vi "TCE.vi"() -> (11 "placeholder image":T1(plugin-control))   [LabVIEW 2020]
uses:
  <vilib>/vision/Image Controls.llb/IMAQ Image.ctl
  DataCluster_TCAL.ctl
  TCE_Config.ctl
  <vilib>/Utility/file.llb/Read Delimited Spreadsheet (string).vi
  <vilib>/Utility/file.llb/Write Delimited Spreadsheet (string).vi
  <vilib>/Analysis/NI_AALBase.lvlib
panel:
  out "FreezeFract Concatinated":dbl[](array[numeric])
  in  "Correct Data":bool
  out "Offset Applied?":bool
  out "recentPaths":path[](array[path])=[path "D:/OneDrive/OneDrive - Aarhus Universitet/Data/D20_4/Result Data.csv"]
  out "version":string="version 0.0.0.1" caption="Version"
  out "Title":string="Thermal Camera Evaluation" caption="Version"
  in  "Remove_Correction":bool
  out "Offsets":dbl[](array[numeric])
  in  "Calc_All":bool
  in  "Well":i32=251
  in  "ImageIdx":u32(slide)=98 scale=0.0..527.0
  in  "Path":path
  out "MeltTemps":dbl[](array[numeric])=[-5.408275862068933, -5.766551724137912, -5.134827586206882, -4.684827586206836, -7.485172413793066, -5.2834482758620425, -5.345517241379298, -6.320689655172373, -3.992413793103424, -3.7082758620689447, -3.4782758620689265, -5.388275862068895, -5.597241379310333, -4.740689655172389, -4.031034482758571, -4.187241379310308, -6.245172413793114, -4.773793103448213, -4.427586206896535, -3.742413793103424, -4.568965517241338, -5.621379310344764, -4.7503448275861615, -5.029999999999973, -5.895517241379309, -4.551379310344771, -4.0196551724137635, -4.698965517241334, -4.126551724137926, -2.993448275862022, -4.383448275862065, -4.888965517241331, -5.901724137931012, -8.037586206896549, -3.918275862068924, -4.438620689655181, -5.749655172413782, -4.38241379310341, -4.932758620689583, -4.997586206896528, -4.125862068965489, -3.4279310344827536, -5.144482758620654, -2.891379310344803, -2.92999999999995, -3.1620689655172214, -3.216206896551739, -4.3248275862068795, -1.3320689655172373, -2.026551724137903, 0.5675862068965785, -0.5103448275861524, 0.4782758620689833, -1.9634482758620493, -0.1275862068965239, -0.1651724137930728, -0.9937931034482403, -0.6210344827586027, 0.2934482758620902, 0.6917241379310894, 1.3537931034483108, -1.852758620689599, -1.3782758620689037, 1.2606896551724844, -0.0275862068965012, -2.2548275862068294, -1.0710344827585914, -1.4565517241379098, -0.7220689655172237, -0.853793103448254, -0.2686206896551653, -0.5562068965517142, 0.0324137931034443, -0.2768965517241213, 1.1982758620689538, 1.2775862068966148, -0.6427586206896194, 0.5986206896552062, -0.3313793103448006, -0.6034482758620356, -2.0755172413792593, -2.182758620689583, -1.6548275862068635, -0.7234482758620402, -0.6872413793103078, -0.9086206896551516, -0.5427586206895967, -0.0527586206895876, 1.211379310344853, 0.2365517241379393, -0.526551724137903, -0.1537931034482085, 1.1865517241379848, 0.7089655172413813, -1.8837931034482267, 0.5872413793103988, -2.0686206896551766, -2.519310344827545, -2.2079310344827263, -2.2441379310344587, -2.0355172413792957, -2.3782758620689037, -2.0879310344827218, -1.998965517241345, -2.0948275862068613, -2.1227586206896376, -2.195517241379264, -1.969655172413752, -2.0175862068965102, -2.061724137931037, -2.028275862068938, -1.7403448275861706, -2.1765517241378802, -2.432758620689583, -2.186551724137928, -2.063448275862015, -2.331724137931019, -2.1351724137931, -2.0499999999999545, -2.1537931034482085, -2.235172413793066, -2.213793103448211, -2.082758620689617, -2.1703448275861774, -2.0434482758620334, -2.173448275862029, -1.9048275862068635, -1.683793103448238, -1.8931034482758378, -2.165172413793073, -2.068965517241338, -2.1862068965517096, -2.161034482758623, -2.085517241379307, -2.0631034482758537, -2.134137931034445, -2.104827586206852, -2.1775862068965353, -2.2255172413792934, -2.161724137931003, -2.0251724137930864, -2.0106896551724276, -2.211379310344796, -1.9093103448275315, -2.3158620689654867, -1.9827586206895944, -2.258275862068899, -2.2927586206895967, -2.0868965517241236, -2.0810344827585823, -2.17931034482757, -2.134137931034445, -2.151379310344794, -2.101034482758621, -2.2465517241379303, -2.339999999999975, -2.061379310344819, -2.082413793103399, -2.220689655172407, -2.0658620689654867, -2.1337931034482267, -2.0158620689654754, -2.1179310344827513, -2.1999999999999886, -2.130344827586157, -2.0489655172413563, -2.0534482758620243, -2.0851724137930887, -2.1079310344827036, -2.0241379310344882, -2.0693103448275565, -2.1348275862068817, -2.1431034482758378, -2.0268965517241213, -2.0317241379310076, -1.6172413793103146, -2.02103448275858, -2.331724137931019, -2.4068965517241168, -2.2337931034482494, -2.383103448275847, -2.1417241379310212, -2.1768965517240986, -2.2579310344827377, -2.1786206896551334, -2.032068965517226, -2.1162068965517165, -2.2706896551724185, -1.9220689655172123, -2.174482758620684, -2.11206896551721, -2.0858620689654686, -0.1458620689654708, -0.1541379310344837, -0.0103448275861524, -0.2106896551724162, -0.2299999999999613, -0.243448275862022, -0.2624137931034056, -0.2906896551724003, -0.3306896551724208, -0.3089655172413472, -0.2099999999999795, -0.276551724137903, -0.15896551724137, -0.0637931034482335, -0.2572413793103578, 0.1706896551724526, -0.0779310344827309, -0.0958620689654595, 0.0658620689655436, -0.1041379310344723, -0.4631034482758308, -0.1158620689654981, -0.1268965517240872, -0.3313793103448006, -0.2803448275861911, -0.1562068965517369, -0.06793103448274, -0.131379310344812, -0.0282758620689378, 0.0079310344827945, 0.0748275862069363, 0.2665517241379689, 0.0537931034482995, -0.2062068965516914, -0.1179310344827513, -0.3424137931033897, -0.0275862068965012, -0.2003448275861501, -0.1096551724137953, -0.0944827586206429, -0.4137931034482563, -0.5093103448275542, 0.0627586206896922, -0.1789655172413518, -0.0096551724137726, 0.0068965517241395, -0.0334482758620425, 0.2120689655172896, -0.1099999999999568, -0.2282758620689265, -0.1213793103447642, -0.1482758620689424, -0.2106896551724162, -0.0927586206896081, -0.1093103448275201, -0.076206896551696, -0.1593103448275315, -0.0886206896551585, -0.1924137931034124, -0.0558620689654958, -0.0313793103447892, -0.0799999999999841, -0.1262068965517074, 0.2117241379310713, -0.1141379310344632, -0.1796551724137885, -0.2003448275861501, -0.0327586206896058, 0.0655172413793252, -0.1886206896551812, -0.0327586206896058, -0.1424137931034011, -0.2406896551723889, -0.034827586206859, -0.1527586206896103, -0.1848275862068363, -0.0313793103447892, -0.0158620689654754, -0.0372413793103306, 0.2079310344827832, -0.2451724137931137, -0.6586206896551516, -0.0858620689654686, -0.2462068965517119, -0.2631034482758423, -0.0217241379310167, -0.2486206896551266, 0.0455172413793434, -0.2441379310344587, -0.1786206896551334, -0.230689655172398, -0.0131034482758423, -0.2613793103448074, -0.4093103448275315, -0.0124137931034056, 0.1572413793103919, 0.0, 0.0, 0.0, 1.7110344827586346, 1.5944827586206998, 1.9227586206896488, 0.1648275862069113, 1.3268965517241327, 0.0, 0.0, 0.0, 1.441379310344871, 0.8996551724138158, 2.017586206896567, 1.1068965517241622, 2.3413793103448484, 1.119655172413843, 1.9251724137931205, 1.484482758620743, 1.7410344827586641, 1.624137931034511, 1.9227586206896488, 1.88793103448279, 1.3758620689655459, -0.8037931034482426, 1.6562068965517938, 1.90758620689661, 2.0327586206896626, 1.5831034482758923, 2.1006896551724594, 2.216206896551796, 2.153448275862104, 1.9158620689655093, 2.1862068965517665, 1.9189655172414175, 2.0968965517241713, 1.4434482758620675, 1.914482758620693, 1.868620689655188, 1.9841379310345246, 2.0734482758621198, 1.9231034482759242, 1.7982758620689765, 1.852068965517276, 2.086551724137962, 2.055172413793173, 1.9510344827586437, 2.1220689655172578, 2.108620689655197, 2.3431034482758832, 0.0, 1.7272413793103851, 2.039655172413859, 1.9255172413793389, 2.2200000000000273, 1.5868965517241804, 1.914482758620693, 1.9610344827586343, 2.145517241379366, 1.9279310344828102, 1.8203448275862115, 2.199310344827609, 2.312413793103474, 2.407931034482772, 2.4206896551724526, 1.8224137931034647, 2.3637931034483017, 1.6882758620689629, 1.8193103448276133, 1.7324137931034898, 2.3037931034482995, 1.794137931034527, 2.011034482758646, 2.0013793103448734, 1.7558620689655413, 1.8893103448276065, 2.1520689655172873, 1.9962068965517685, 2.3103448275862206, 2.1217241379310963, 1.863103448275922, 1.9231034482759242, 1.5434482758620902, 1.6648275862069113, 1.8944827586207111, 1.63793103448279, 1.8379310344827786, 1.948620689655229, 2.157241379310392, 1.835517241379364, 1.950344827586207, 2.018275862069004, 1.9565517241379666, 1.7651724137931524, 2.068965517241395, 2.168275862068981]
  out "FreezeArray":bool[](array[boolean])=[TRUE, TRUE, TRUE, TRUE, TRUE, TRUE, TRUE, TRUE, TRUE, TRUE, TRUE, TRUE, TRUE, TRUE, TRUE, TRUE, TRUE, TRUE, TRUE, TRUE, TRUE, TRUE, TRUE, TRUE, TRUE, TRUE, TRUE, TRUE, TRUE, TRUE, TRUE, TRUE, TRUE, TRUE, TRUE, TRUE, TRUE, TRUE, TRUE, TRUE, TRUE, TRUE, TRUE, TRUE, TRUE, TRUE, TRUE, TRUE, TRUE, TRUE, TRUE, TRUE, TRUE, TRUE, TRUE, TRUE, TRUE, TRUE, TRUE, TRUE, TRUE, TRUE, TRUE, TRUE, TRUE, TRUE, TRUE, TRUE, TRUE, TRUE, TRUE, TRUE, TRUE, TRUE, TRUE, TRUE, TRUE, TRUE, TRUE, TRUE, TRUE, TRUE, TRUE, TRUE, TRUE, TRUE, TRUE, TRUE, TRUE, TRUE, TRUE, TRUE, TRUE, TRUE, TRUE, TRUE, TRUE, TRUE, TRUE, TRUE, TRUE, TRUE, TRUE, TRUE, TRUE, TRUE, TRUE, TRUE, TRUE, TRUE, TRUE, TRUE, TRUE, TRUE, TRUE, TRUE, TRUE, TRUE, TRUE, TRUE, TRUE, TRUE, TRUE, TRUE, TRUE, TRUE, TRUE, TRUE, TRUE, TRUE, TRUE, TRUE, TRUE, TRUE, TRUE, TRUE, TRUE, TRUE, TRUE, TRUE, TRUE, TRUE, TRUE, TRUE, TRUE, TRUE, TRUE, TRUE, TRUE, TRUE, TRUE, TRUE, TRUE, TRUE, TRUE, TRUE, TRUE, TRUE, TRUE, TRUE, TRUE, TRUE, TRUE, TRUE, TRUE, TRUE, TRUE, TRUE, TRUE, TRUE, TRUE, TRUE, TRUE, TRUE, TRUE, TRUE, TRUE, TRUE, TRUE, TRUE, TRUE, TRUE, TRUE, TRUE, TRUE, TRUE, TRUE, TRUE, TRUE, TRUE, TRUE, TRUE, TRUE, TRUE, TRUE, TRUE, TRUE, TRUE, TRUE, TRUE, TRUE, TRUE, TRUE, TRUE, TRUE, TRUE, TRUE, TRUE, TRUE, TRUE, TRUE, TRUE, TRUE, TRUE, TRUE, TRUE, TRUE, TRUE, TRUE, TRUE, TRUE, TRUE, TRUE, TRUE, TRUE, TRUE, TRUE, TRUE, TRUE, TRUE, TRUE, TRUE, TRUE, TRUE, TRUE, TRUE, TRUE, TRUE, TRUE, TRUE, TRUE, TRUE, TRUE, TRUE, TRUE, TRUE, TRUE, TRUE, TRUE, TRUE, TRUE, TRUE, TRUE, TRUE, TRUE, TRUE, TRUE, TRUE, TRUE, TRUE, TRUE, TRUE, TRUE, TRUE, TRUE, TRUE, TRUE, TRUE, TRUE, TRUE, TRUE, TRUE, TRUE, TRUE, TRUE, TRUE, TRUE, TRUE, TRUE, TRUE, TRUE, TRUE, TRUE, TRUE, TRUE, TRUE, TRUE, TRUE, FALSE, FALSE, FALSE, TRUE, TRUE, TRUE, TRUE, TRUE, FALSE, FALSE, FALSE, TRUE, TRUE, TRUE, TRUE, TRUE, TRUE, TRUE, TRUE, TRUE, TRUE, TRUE, TRUE, TRUE, TRUE, TRUE, TRUE, TRUE, TRUE, TRUE, TRUE, TRUE, TRUE, TRUE, TRUE, TRUE, TRUE, TRUE, TRUE, TRUE, TRUE, TRUE, TRUE, TRUE, TRUE, TRUE, TRUE, TRUE, TRUE, TRUE, FALSE, TRUE, TRUE, TRUE, TRUE, TRUE, TRUE, TRUE, TRUE, TRUE, TRUE, TRUE, TRUE, TRUE, TRUE, TRUE, TRUE, TRUE, TRUE, TRUE, TRUE, TRUE, TRUE, TRUE, TRUE, TRUE, TRUE, TRUE, TRUE, TRUE, TRUE, TRUE, TRUE, TRUE, TRUE, TRUE, TRUE, TRUE, TRUE, TRUE, TRUE, TRUE, TRUE, TRUE, TRUE, TRUE]
  out "ThermTemps":dbl[](array[numeric])
  out "PartitionArray":string[](array[string])=["A, MQ unfiltered", "A, MQ unfiltered", "A, MQ unfiltered", "A, MQ unfiltered", "A, MQ unfiltered", "A, MQ unfiltered", "A, MQ unfiltered", "A, MQ unfiltered", "A, MQ unfiltered", "A, MQ unfiltered", "A, MQ unfiltered", "A, MQ unfiltered", "A, MQ unfiltered", "A, MQ unfiltered", "A, MQ unfiltered", "A, MQ unfiltered", "A, MQ unfiltered", "A, MQ unfiltered", "A, MQ unfiltered", "A, MQ unfiltered", "A, MQ unfiltered", "A, MQ unfiltered", "A, MQ unfiltered", "A, MQ unfiltered", "A, MQ unfiltered", "A, MQ unfiltered", "A, MQ unfiltered", "A, MQ unfiltered", "A, MQ unfiltered", "A, MQ unfiltered", "A, MQ unfiltered", "A, MQ unfiltered", "A, MQ unfiltered", "A, MQ unfiltered", "A, MQ unfiltered", "A, MQ unfiltered", "A, MQ unfiltered", "A, MQ unfiltered", "A, MQ unfiltered", "A, MQ unfiltered", "A, MQ unfiltered", "A, MQ unfiltered", "A, MQ unfiltered", "A, MQ unfiltered", "A, MQ unfiltered", "A, MQ unfiltered", "A, MQ unfiltered", "A, MQ unfiltered", "B, D2O unfiltered", "B, D2O unfiltered", "B, D2O unfiltered", "B, D2O unfiltered", "B, D2O unfiltered", "B, D2O unfiltered", "B, D2O unfiltered", "B, D2O unfiltered", "B, D2O unfiltered", "B, D2O unfiltered", "B, D2O unfiltered", "B, D2O unfiltered", "B, D2O unfiltered", "B, D2O unfiltered", "B, D2O unfiltered", "B, D2O unfiltered", "B, D2O unfiltered", "B, D2O unfiltered", "B, D2O unfiltered", "B, D2O unfiltered", "B, D2O unfiltered", "B, D2O unfiltered", "B, D2O unfiltered", "B, D2O unfiltered", "B, D2O unfiltered", "B, D2O unfiltered", "B, D2O unfiltered", "B, D2O unfiltered", "B, D2O unfiltered", "B, D2O unfiltered", "B, D2O unfiltered", "B, D2O unfiltered", "B, D2O unfiltered", "B, D2O unfiltered", "B, D2O unfiltered", "B, D2O unfiltered", "B, D2O unfiltered", "B, D2O unfiltered", "B, D2O unfiltered", "B, D2O unfiltered", "B, D2O unfiltered", "B, D2O unfiltered", "B, D2O unfiltered", "B, D2O unfiltered", "B, D2O unfiltered", "B, D2O unfiltered", "B, D2O unfiltered", "B, D2O unfiltered", "C, 1mg/ml Snomax in MQ", "C, 1mg/ml Snomax in MQ", "C, 1mg/ml Snomax in MQ", "C, 1mg/ml Snomax in MQ", "C, 1mg/ml Snomax in MQ", "C, 1mg/ml Snomax in MQ", "C, 1mg/ml Snomax in MQ", "C, 1mg/ml Snomax in MQ", "C, 1mg/ml Snomax in MQ", "C, 1mg/ml Snomax in MQ", "C, 1mg/ml Snomax in MQ", "C, 1mg/ml Snomax in MQ", "C, 1mg/ml Snomax in MQ", "C, 1mg/ml Snomax in MQ", "C, 1mg/ml Snomax in MQ", "C, 1mg/ml Snomax in MQ", "C, 1mg/ml Snomax in MQ", "C, 1mg/ml Snomax in MQ", "C, 1mg/ml Snomax in MQ", "C, 1mg/ml Snomax in MQ", "C, 1mg/ml Snomax in MQ", "C, 1mg/ml Snomax in MQ", "C, 1mg/ml Snomax in MQ", "C, 1mg/ml Snomax in MQ", "C, 1mg/ml Snomax in MQ", "C, 1mg/ml Snomax in MQ", "C, 1mg/ml Snomax in MQ", "C, 1mg/ml Snomax in MQ", "C, 1mg/ml Snomax in MQ", "C, 1mg/ml Snomax in MQ", "C, 1mg/ml Snomax in MQ", "C, 1mg/ml Snomax in MQ", "C, 1mg/ml Snomax in MQ", "C, 1mg/ml Snomax in MQ", "C, 1mg/ml Snomax in MQ", "C, 1mg/ml Snomax in MQ", "C, 1mg/ml Snomax in MQ", "C, 1mg/ml Snomax in MQ", "C, 1mg/ml Snomax in MQ", "C, 1mg/ml Snomax in MQ", "C, 1mg/ml Snomax in MQ", "C, 1mg/ml Snomax in MQ", "C, 1mg/ml Snomax in MQ", "C, 1mg/ml Snomax in MQ", "C, 1mg/ml Snomax in MQ", "C, 1mg/ml Snomax in MQ", "C, 1mg/ml Snomax in MQ", "C, 1mg/ml Snomax in MQ", "C, 1mg/ml Snomax in MQ", "C, 1mg/ml Snomax in MQ", "C, 1mg/ml Snomax in MQ", "C, 1mg/ml Snomax in MQ", "C, 1mg/ml Snomax in MQ", "C, 1mg/ml Snomax in MQ", "C, 1mg/ml Snomax in MQ", "C, 1mg/ml Snomax in MQ", "C, 1mg/ml Snomax in MQ", "C, 1mg/ml Snomax in MQ", "C, 1mg/ml Snomax in MQ", "C, 1mg/ml Snomax in MQ", "C, 1mg/ml Snomax in MQ", "C, 1mg/ml Snomax in MQ", "C, 1mg/ml Snomax in MQ", "C, 1mg/ml Snomax in MQ", "C, 1mg/ml Snomax in MQ", "C, 1mg/ml Snomax in MQ", "C, 1mg/ml Snomax in MQ", "C, 1mg/ml Snomax in MQ", "C, 1mg/ml Snomax in MQ", "C, 1mg/ml Snomax in MQ", "C, 1mg/ml Snomax in MQ", "C, 1mg/ml Snomax in MQ", "C, 1mg/ml Snomax in MQ", "C, 1mg/ml Snomax in MQ", "C, 1mg/ml Snomax in MQ", "C, 1mg/ml Snomax in MQ", "C, 1mg/ml Snomax in MQ", "C, 1mg/ml Snomax in MQ", "C, 1mg/ml Snomax in MQ", "C, 1mg/ml Snomax in MQ", "C, 1mg/ml Snomax in MQ", "C, 1mg/ml Snomax in MQ", "C, 1mg/ml Snomax in MQ", "C, 1mg/ml Snomax in MQ", "C, 1mg/ml Snomax in MQ", "C, 1mg/ml Snomax in MQ", "C, 1mg/ml Snomax in MQ", "C, 1mg/ml Snomax in MQ", "C, 1mg/ml Snomax in MQ", "C, 1mg/ml Snomax in MQ", "C, 1mg/ml Snomax in MQ", "C, 1mg/ml Snomax in MQ", "C, 1mg/ml Snomax in MQ", "C, 1mg/ml Snomax in MQ", "C, 1mg/ml Snomax in MQ", "C, 1mg/ml Snomax in MQ", "D, 1mg/ml Snomax in 1:1 MQ:D2O", "D, 1mg/ml Snomax in 1:1 MQ:D2O", "D, 1mg/ml Snomax in 1:1 MQ:D2O", "D, 1mg/ml Snomax in 1:1 MQ:D2O", "D, 1mg/ml Snomax in 1:1 MQ:D2O", "D, 1mg/ml Snomax in 1:1 MQ:D2O", "D, 1mg/ml Snomax in 1:1 MQ:D2O", "D, 1mg/ml Snomax in 1:1 MQ:D2O", "D, 1mg/ml Snomax in 1:1 MQ:D2O", "D, 1mg/ml Snomax in 1:1 MQ:D2O", "D, 1mg/ml Snomax in 1:1 MQ:D2O", "D, 1mg/ml Snomax in 1:1 MQ:D2O", "D, 1mg/ml Snomax in 1:1 MQ:D2O", "D, 1mg/ml Snomax in 1:1 MQ:D2O", "D, 1mg/ml Snomax in 1:1 MQ:D2O", "D, 1mg/ml Snomax in 1:1 MQ:D2O", "D, 1mg/ml Snomax in 1:1 MQ:D2O", "D, 1mg/ml Snomax in 1:1 MQ:D2O", "D, 1mg/ml Snomax in 1:1 MQ:D2O", "D, 1mg/ml Snomax in 1:1 MQ:D2O", "D, 1mg/ml Snomax in 1:1 MQ:D2O", "D, 1mg/ml Snomax in 1:1 MQ:D2O", "D, 1mg/ml Snomax in 1:1 MQ:D2O", "D, 1mg/ml Snomax in 1:1 MQ:D2O", "D, 1mg/ml Snomax in 1:1 MQ:D2O", "D, 1mg/ml Snomax in 1:1 MQ:D2O", "D, 1mg/ml Snomax in 1:1 MQ:D2O", "D, 1mg/ml Snomax in 1:1 MQ:D2O", "D, 1mg/ml Snomax in 1:1 MQ:D2O", "D, 1mg/ml Snomax in 1:1 MQ:D2O", "D, 1mg/ml Snomax in 1:1 MQ:D2O", "D, 1mg/ml Snomax in 1:1 MQ:D2O", "D, 1mg/ml Snomax in 1:1 MQ:D2O", "D, 1mg/ml Snomax in 1:1 MQ:D2O", "D, 1mg/ml Snomax in 1:1 MQ:D2O", "D, 1mg/ml Snomax in 1:1 MQ:D2O", "D, 1mg/ml Snomax in 1:1 MQ:D2O", "D, 1mg/ml Snomax in 1:1 MQ:D2O", "D, 1mg/ml Snomax in 1:1 MQ:D2O", "D, 1mg/ml Snomax in 1:1 MQ:D2O", "D, 1mg/ml Snomax in 1:1 MQ:D2O", "D, 1mg/ml Snomax in 1:1 MQ:D2O", "D, 1mg/ml Snomax in 1:1 MQ:D2O", "D, 1mg/ml Snomax in 1:1 MQ:D2O", "D, 1mg/ml Snomax in 1:1 MQ:D2O", "D, 1mg/ml Snomax in 1:1 MQ:D2O", "D, 1mg/ml Snomax in 1:1 MQ:D2O", "D, 1mg/ml Snomax in 1:1 MQ:D2O", "D, 1mg/ml Snomax in 1:1 MQ:D2O", "D, 1mg/ml Snomax in 1:1 MQ:D2O", "D, 1mg/ml Snomax in 1:1 MQ:D2O", "D, 1mg/ml Snomax in 1:1 MQ:D2O", "D, 1mg/ml Snomax in 1:1 MQ:D2O", "D, 1mg/ml Snomax in 1:1 MQ:D2O", "D, 1mg/ml Snomax in 1:1 MQ:D2O", "D, 1mg/ml Snomax in 1:1 MQ:D2O", "D, 1mg/ml Snomax in 1:1 MQ:D2O", "D, 1mg/ml Snomax in 1:1 MQ:D2O", "D, 1mg/ml Snomax in 1:1 MQ:D2O", "D, 1mg/ml Snomax in 1:1 MQ:D2O", "D, 1mg/ml Snomax in 1:1 MQ:D2O", "D, 1mg/ml Snomax in 1:1 MQ:D2O", "D, 1mg/ml Snomax in 1:1 MQ:D2O", "D, 1mg/ml Snomax in 1:1 MQ:D2O", "D, 1mg/ml Snomax in 1:1 MQ:D2O", "D, 1mg/ml Snomax in 1:1 MQ:D2O", "D, 1mg/ml Snomax in 1:1 MQ:D2O", "D, 1mg/ml Snomax in 1:1 MQ:D2O", "D, 1mg/ml Snomax in 1:1 MQ:D2O", "D, 1mg/ml Snomax in 1:1 MQ:D2O", "D, 1mg/ml Snomax in 1:1 MQ:D2O", "D, 1mg/ml Snomax in 1:1 MQ:D2O", "D, 1mg/ml Snomax in 1:1 MQ:D2O", "D, 1mg/ml Snomax in 1:1 MQ:D2O", "D, 1mg/ml Snomax in 1:1 MQ:D2O", "D, 1mg/ml Snomax in 1:1 MQ:D2O", "D, 1mg/ml Snomax in 1:1 MQ:D2O", "D, 1mg/ml Snomax in 1:1 MQ:D2O", "D, 1mg/ml Snomax in 1:1 MQ:D2O", "D, 1mg/ml Snomax in 1:1 MQ:D2O", "D, 1mg/ml Snomax in 1:1 MQ:D2O", "D, 1mg/ml Snomax in 1:1 MQ:D2O", "D, 1mg/ml Snomax in 1:1 MQ:D2O", "D, 1mg/ml Snomax in 1:1 MQ:D2O", "D, 1mg/ml Snomax in 1:1 MQ:D2O", "D, 1mg/ml Snomax in 1:1 MQ:D2O", "D, 1mg/ml Snomax in 1:1 MQ:D2O", "D, 1mg/ml Snomax in 1:1 MQ:D2O", "D, 1mg/ml Snomax in 1:1 MQ:D2O", "D, 1mg/ml Snomax in 1:1 MQ:D2O", "D, 1mg/ml Snomax in 1:1 MQ:D2O", "D, 1mg/ml Snomax in 1:1 MQ:D2O", "D, 1mg/ml Snomax in 1:1 MQ:D2O", "D, 1mg/ml Snomax in 1:1 MQ:D2O", "D, 1mg/ml Snomax in 1:1 MQ:D2O", "D, 1mg/ml Snomax in 1:1 MQ:D2O", "E, 1mg/ml Snomax in D2O", "E, 1mg/ml Snomax in D2O", "E, 1mg/ml Snomax in D2O", "E, 1mg/ml Snomax in D2O", "E, 1mg/ml Snomax in D2O", "E, 1mg/ml Snomax in D2O", "E, 1mg/ml Snomax in D2O", "E, 1mg/ml Snomax in D2O", "E, 1mg/ml Snomax in D2O", "E, 1mg/ml Snomax in D2O", "E, 1mg/ml Snomax in D2O", "E, 1mg/ml Snomax in D2O", "E, 1mg/ml Snomax in D2O", "E, 1mg/ml Snomax in D2O", "E, 1mg/ml Snomax in D2O", "E, 1mg/ml Snomax in D2O", "E, 1mg/ml Snomax in D2O", "E, 1mg/ml Snomax in D2O", "E, 1mg/ml Snomax in D2O", "E, 1mg/ml Snomax in D2O", "E, 1mg/ml Snomax in D2O", "E, 1mg/ml Snomax in D2O", "E, 1mg/ml Snomax in D2O", "E, 1mg/ml Snomax in D2O", "E, 1mg/ml Snomax in D2O", "E, 1mg/ml Snomax in D2O", "E, 1mg/ml Snomax in D2O", "E, 1mg/ml Snomax in D2O", "E, 1mg/ml Snomax in D2O", "E, 1mg/ml Snomax in D2O", "E, 1mg/ml Snomax in D2O", "E, 1mg/ml Snomax in D2O", "E, 1mg/ml Snomax in D2O", "E, 1mg/ml Snomax in D2O", "E, 1mg/ml Snomax in D2O", "E, 1mg/ml Snomax in D2O", "E, 1mg/ml Snomax in D2O", "E, 1mg/ml Snomax in D2O", "E, 1mg/ml Snomax in D2O", "E, 1mg/ml Snomax in D2O", "E, 1mg/ml Snomax in D2O", "E, 1mg/ml Snomax in D2O", "E, 1mg/ml Snomax in D2O", "E, 1mg/ml Snomax in D2O", "E, 1mg/ml Snomax in D2O", "E, 1mg/ml Snomax in D2O", "E, 1mg/ml Snomax in D2O", "E, 1mg/ml Snomax in D2O", "E, 1mg/ml Snomax in D2O", "E, 1mg/ml Snomax in D2O", "E, 1mg/ml Snomax in D2O", "E, 1mg/ml Snomax in D2O", "E, 1mg/ml Snomax in D2O", "E, 1mg/ml Snomax in D2O", "E, 1mg/ml Snomax in D2O", "E, 1mg/ml Snomax in D2O", "E, 1mg/ml Snomax in D2O", "E, 1mg/ml Snomax in D2O", "E, 1mg/ml Snomax in D2O", "E, 1mg/ml Snomax in D2O", "E, 1mg/ml Snomax in D2O", "E, 1mg/ml Snomax in D2O", "E, 1mg/ml Snomax in D2O", "E, 1mg/ml Snomax in D2O", "E, 1mg/ml Snomax in D2O", "E, 1mg/ml Snomax in D2O", "E, 1mg/ml Snomax in D2O", "E, 1mg/ml Snomax in D2O", "E, 1mg/ml Snomax in D2O", "E, 1mg/ml Snomax in D2O", "E, 1mg/ml Snomax in D2O", "E, 1mg/ml Snomax in D2O", "E, 1mg/ml Snomax in D2O", "E, 1mg/ml Snomax in D2O", "E, 1mg/ml Snomax in D2O", "E, 1mg/ml Snomax in D2O", "E, 1mg/ml Snomax in D2O", "E, 1mg/ml Snomax in D2O", "E, 1mg/ml Snomax in D2O", "E, 1mg/ml Snomax in D2O", "E, 1mg/ml Snomax in D2O", "E, 1mg/ml Snomax in D2O", "E, 1mg/ml Snomax in D2O", "E, 1mg/ml Snomax in D2O", "E, 1mg/ml Snomax in D2O", "E, 1mg/ml Snomax in D2O", "E, 1mg/ml Snomax in D2O", "E, 1mg/ml Snomax in D2O", "E, 1mg/ml Snomax in D2O", "E, 1mg/ml Snomax in D2O", "E, 1mg/ml Snomax in D2O", "E, 1mg/ml Snomax in D2O", "E, 1mg/ml Snomax in D2O", "E, 1mg/ml Snomax in D2O", "E, 1mg/ml Snomax in D2O", "E, 1mg/ml Snomax in D2O"]
  out "FreezeTemps":dbl[](array[numeric])=[-17.102413793103437, -16.14275862068962, -19.01724137931032, -15.683103448275858, -25.12241379310342, -20.5310344827586, -21.968275862068907, -23.725862068965483, -16.464137931034486, -13.113793103448245, -11.636206896551698, -22.81517241379308, -23.049655172413765, -15.513103448275842, -18.779655172413783, -15.36448275862068, -23.218620689655154, -14.564137931034452, -14.352413793103437, -11.641724137931021, -17.657241379310335, -21.99793103448272, -23.813103448275854, -20.459310344827543, -22.592068965517228, -22.526206896551713, -16.890344827586148, -17.801724137931018, -17.235862068965474, -11.44310344827585, -16.035862068965457, -17.472413793103414, -17.914827586206854, -25.26724137931032, -15.10206896551722, -15.265862068965474, -22.079999999999984, -18.58586206896547, -20.5106896551724, -21.002758620689605, -21.88206896551722, -14.302068965517208, -23.049655172413765, -11.56448275862067, -9.727586206896547, -10.574482758620661, -10.471724137931005, -14.189999999999998, -18.853448275862036, -20.565517241379297, -14.187241379310308, -14.840344827586193, -14.906206896551737, -21.08172413793102, -19.829655172413766, -16.151379310344794, -20.792413793103407, -21.82482758620685, -14.474482758620638, -8.87551724137927, -5.148275862068942, -22.100689655172403, -21.813103448275854, -5.387931034482733, -13.19965517241377, -22.069655172413775, -20.66206896551722, -20.594137931034453, -19.319655172413775, -20.309999999999974, -16.707241379310346, -21.968275862068907, -18.70620689655172, -18.623448275862046, -6.637931034482733, -7.056206896551714, -22.052068965517208, -9.618275862068913, -16.901724137931012, -13.387241379310353, -20.70034482758618, -21.344137931034453, -21.40620689655171, -16.127241379310362, -20.572413793103408, -19.566206896551705, -19.49379310344824, -16.083448275862054, -5.782758620689606, -14.221034482758569, -19.863103448275837, -17.482068965517215, -5.9048275862068635, -8.006896551724083, -20.81793103448271, -11.433103448275858, -5.199999999999989, -5.525862068965466, -5.633448275862065, -5.417241379310326, -5.608965517241359, -5.6537931034482085, -5.74655172413793, -5.684482758620675, -5.691379310344814, -5.6758620689655, -5.808620689655129, -5.717586206896556, -5.676206896551719, -5.526896551724121, -5.435517241379273, -5.398620689655161, -5.285172413793077, -5.59172413793101, -5.664482758620636, -5.389999999999986, -5.610344827586175, -5.809999999999945, -5.582413793103399, -5.736896551724101, -5.824482758620661, -5.701379310344805, -5.67655172413788, -5.683103448275858, -5.648965517241322, -5.654482758620645, -5.394482758620654, -5.2789655172413745, -5.4324137931034215, -5.434482758620675, -5.513448275862061, -5.627931034482742, -5.778275862068938, -5.713103448275831, -5.601034482758621, -5.630689655172375, -5.699310344827552, -5.584482758620652, -5.70379310344822, -5.636896551724078, -5.628275862068904, -5.4948275862068385, -5.689310344827561, -5.402413793103392, -5.240689655172389, -5.448275862068897, -5.5555172413792775, -5.998965517241345, -5.548965517241356, -5.420689655172396, -5.645862068965471, -5.577931034482731, -5.6520689655172305, -5.590344827586193, -5.699999999999989, -5.640689655172423, -5.6299999999999955, -5.599310344827529, -5.45034482758615, -5.28793103448271, -5.263793103448222, -5.557931034482749, -5.471034482758569, -5.670344827586177, -5.626551724137926, -5.3606896551723935, -5.553448275862024, -5.736206896551721, -5.485517241379284, -5.536206896551732, -5.615862068965498, -5.4589655172413245, -5.904137931034484, -5.572413793103408, -5.5565517241379325, -5.072413793103408, -5.54482758620685, -5.425172413793064, -5.9865517241378825, -5.601724137931001, -5.816551724137923, -5.833448275862054, -5.495517241379275, -5.722068965517224, -5.5058620689654845, -5.552758620689588, -5.644137931034493, -5.5610344827586005, -5.523793103448213, -5.626551724137926, -5.5406896551724, -5.328275862068949, -2.799310344827518, -3.109999999999957, -3.088965517241377, -3.2558620689654845, -3.3810344827585936, -3.349310344827529, -3.327931034482731, -3.3241379310344428, -3.2679310344827286, -3.4796551724138, -3.1096551724137953, -3.299655172413793, -3.301379310344771, -3.1603448275861865, -2.941034482758596, -2.9506896551724253, -2.8889655172413313, -3.0858620689654686, -2.980689655172398, -3.146896551724126, -3.077931034482731, -3.2044827586206566, -3.164482758620636, -3.3927586206896194, -3.373103448275856, -3.2824137931033874, -3.2603448275861524, -3.264482758620659, -3.188275862068906, -3.086206896551687, -2.978965517241363, -2.9113793103447847, -2.8717241379310394, -3.0813793103448006, -3.0013793103448165, -2.8927586206896194, -3.1879310344827445, -3.2431034482758605, -3.254482758620668, -3.1889655172413427, -3.319655172413775, -3.3893103448275497, -3.1068965517241054, -2.8872413793103533, -2.9982758620689083, -3.2041379310344382, -3.2024137931034033, -2.812413793103417, -2.790344827586182, -3.00068965517238, -3.1693103448275224, -3.193103448275849, -3.195862068965482, -3.1141379310344632, -3.326896551724076, -3.2120689655172328, -3.224137931034477, -3.285862068965457, -3.215862068965464, -3.0582758620689106, -3.1924137931034124, -3.149655172413759, -3.17999999999995, -2.8662068965517165, -2.9058620689654617, -3.0134482758620607, -3.161724137931003, -3.131379310344812, -3.0813793103448006, -3.0351724137930773, -2.9986206896551266, -3.1968965517240804, -3.164482758620636, -3.0810344827585823, -3.220689655172407, -2.9931034482758605, -2.964137931034486, -3.17999999999995, -2.9920689655172055, -2.764827586206877, -2.886896551724078, -3.1758620689655004, -3.071724137931028, -3.196551724137919, -3.2237931034482585, -2.905172413793082, -3.262068965517244, -3.1627586206896012, -3.283793103448261, -3.164482758620636, -3.142413793103401, -3.1089655172413586, -3.034137931034479, -3.277586206896558, -3.0720689655172464, -2.629655172413777, 0.0, 0.0, 0.0, -0.7296551724137998, -1.1386206896551698, -1.0558620689654958, -1.305172413793116, -1.1862068965517096, 0.0, 0.0, 0.0, -1.1282758620689037, -1.1682758620689242, -0.5724137931034079, -1.1765517241378802, -0.2555172413792661, -1.0703448275861547, -0.7648275862068772, -1.057931034482749, -1.016551724137912, -0.9627586206896126, -1.0337931034482608, -0.9872413793103192, -1.2451724137931137, -1.3141379310344519, -1.0437931034482517, -1.0199999999999818, -0.95310344827584, -0.9817241379309962, -0.8799999999999955, -0.7527586206896331, -0.5689655172413381, -0.6779310344827536, -0.7651724137930955, -0.8879310344827331, -0.8582758620689219, -1.0286206896551562, -0.8986206896551607, -1.072413793103408, -0.8858620689654799, -0.9524137931034033, -0.9465517241379189, -0.9465517241379189, -0.6958620689654822, -0.9386206896551812, -0.6879310344827445, -0.8244827586206611, -0.540344827586182, -0.5341379310344792, -0.6255172413792707, 0.0, -0.8917241379310212, -0.8031034482758628, -0.7927586206895967, -0.3927586206896194, -1.0141379310344405, -0.7241379310344769, -0.8258620689654776, -0.8099999999999454, -0.7320689655172146, -0.8993103448275406, -0.6624137931034397, -0.5572413793103124, -0.355517241379289, 0.0244827586207066, -0.6931034482758491, -0.113103448275865, -0.8486206896551494, -0.581724137931019, -0.4658620689654641, -0.1306896551723753, -0.9151724137930728, -0.8689655172413495, -0.5741379310344428, -0.8624137931034284, -0.8899999999999864, -0.8365517241379052, -0.7541379310344496, -0.5631034482758537, -0.4710344827585686, -0.3586206896551403, -0.4551724137930933, -0.7186206896551539, -0.8586206896551403, -0.6134482758620265, -0.6841379310344564, -0.6020689655172191, -0.8358620689654686, -0.6906896551723776, -0.8324137931033988, -0.900689655172414, -0.5879310344827218, -0.8486206896551494, -0.6179310344827513, -0.4758620689654549, -0.4237931034482472]
  out "FreezeIdx":i32[](array[numeric])=[255, 242, 272, 236, 335, 287, 303, 320, 243, 209, 191, 311, 316, 234, 271, 238, 322, 225, 219, 192, 254, 301, 321, 283, 307, 309, 248, 257, 253, 193, 240, 259, 264, 335, 231, 232, 302, 265, 285, 291, 301, 219, 312, 192, 172, 182, 181, 221, 271, 285, 224, 228, 233, 290, 279, 240, 286, 296, 218, 162, 122, 305, 300, 128, 213, 302, 285, 284, 271, 280, 243, 297, 267, 262, 143, 147, 302, 170, 248, 214, 293, 293, 293, 240, 287, 272, 273, 236, 129, 217, 278, 252, 135, 153, 288, 192, 124, 131, 130, 125, 127, 127, 126, 129, 124, 127, 126, 126, 129, 126, 124, 128, 126, 126, 135, 125, 133, 136, 126, 131, 132, 131, 126, 125, 129, 132, 125, 128, 128, 127, 124, 126, 136, 130, 125, 129, 125, 134, 131, 126, 130, 125, 133, 128, 125, 130, 133, 137, 127, 124, 126, 124, 127, 126, 133, 130, 124, 133, 132, 124, 124, 129, 126, 128, 128, 123, 132, 131, 125, 127, 125, 124, 136, 126, 129, 126, 129, 126, 135, 126, 133, 130, 124, 126, 124, 124, 126, 123, 125, 125, 124, 129, 98, 100, 98, 105, 99, 102, 98, 100, 97, 104, 97, 98, 100, 99, 97, 99, 99, 105, 99, 106, 107, 99, 108, 104, 104, 100, 100, 98, 103, 98, 98, 99, 102, 106, 108, 96, 100, 108, 104, 99, 100, 108, 98, 97, 97, 99, 98, 98, 99, 99, 99, 110, 108, 100, 111, 100, 99, 107, 99, 98, 101, 99, 99, 99, 98, 98, 99, 99, 101, 107, 98, 99, 100, 98, 104, 98, 98, 99, 99, 98, 98, 99, 98, 100, 101, 100, 106, 101, 100, 99, 100, 99, 98, 102, 99, 98, 0, 0, 0, 71, 80, 75, 84, 81, 0, 0, 0, 74, 77, 72, 78, 75, 81, 73, 76, 80, 77, 76, 76, 82, 88, 77, 78, 79, 74, 74, 81, 78, 76, 75, 75, 77, 76, 82, 75, 74, 76, 83, 81, 72, 74, 73, 74, 74, 73, 79, 0, 79, 74, 75, 82, 76, 73, 80, 75, 73, 82, 73, 75, 79, 80, 77, 77, 74, 73, 73, 89, 77, 75, 71, 76, 76, 74, 74, 75, 73, 74, 71, 76, 78, 74, 74, 72, 75, 75, 75, 75, 73, 77, 73, 73, 75]
  out "maxSize":i32=527
  out "img":i32
  out "Slide":u8(slide) scale=0.0..100.0
  in  "Help":bool
  out "Tutorial":string="Load Image"
  out "Points":T2[](array[typedef])=[{"X"=62.0, "Y"=65.0}, {"X"=62.333332, "Y"=80.6}, {"X"=62.666668, "Y"=96.2}, {"X"=63.0, "Y"=111.8}, {"X"=63.333332, "Y"=127.4}, {"X"=63.666668, "Y"=143.0}, {"X"=64.0, "Y"=158.6}, {"X"=64.333336, "Y"=174.20001}, {"X"=64.666664, "Y"=189.8}, {"X"=65.0, "Y"=205.40001}, {"X"=65.333336, "Y"=221.0}, {"X"=65.666664, "Y"=236.6}, {"X"=66.0, "Y"=252.20001}, {"X"=66.333336, "Y"=267.8}, {"X"=66.666664, "Y"=283.40002}, {"X"=67.0, "Y"=299.0}, {"X"=77.565216, "Y"=64.695656}, {"X"=77.89855, "Y"=80.295654}, {"X"=78.23188, "Y"=95.89565}, {"X"=78.565216, "Y"=111.49565}, {"X"=78.89855, "Y"=127.09566}, {"X"=79.23188, "Y"=142.69565}, {"X"=79.565216, "Y"=158.29565}, {"X"=79.89855, "Y"=173.89566}, {"X"=80.23188, "Y"=189.49567}, {"X"=80.565216, "Y"=205.09566}, {"X"=80.89855, "Y"=220.69565}, {"X"=81.23188, "Y"=236.29565}, {"X"=81.565216, "Y"=251.89566}, {"X"=81.89855, "Y"=267.49567}, {"X"=82.23188, "Y"=283.09564}, {"X"=82.565216, "Y"=298.69565}, {"X"=93.13043, "Y"=64.391304}, {"X"=93.46377, "Y"=79.9913}, {"X"=93.797104, "Y"=95.59131}, {"X"=94.13043, "Y"=111.19131}, {"X"=94.46377, "Y"=126.791306}, {"X"=94.797104, "Y"=142.3913}, {"X"=95.13043, "Y"=157.9913}, {"X"=95.46377, "Y"=173.59131}, {"X"=95.797104, "Y"=189.19131}, {"X"=96.13043, "Y"=204.79132}, {"X"=96.46377, "Y"=220.39131}, {"X"=96.797104, "Y"=235.99132}, {"X"=97.13043, "Y"=251.59132}, {"X"=97.46377, "Y"=267.1913}, {"X"=97.797104, "Y"=282.79132}, {"X"=98.13043, "Y"=298.3913}, {"X"=108.69565, "Y"=64.08696}, {"X"=109.028984, "Y"=79.68696}, {"X"=109.36232, "Y"=95.28696}, {"X"=109.695656, "Y"=110.88696}, {"X"=110.028984, "Y"=126.48695}, {"X"=110.36232, "Y"=142.08696}, {"X"=110.695656, "Y"=157.68697}, {"X"=111.028984, "Y"=173.28696}, {"X"=111.36232, "Y"=188.88696}, {"X"=111.695656, "Y"=204.48697}, {"X"=112.028984, "Y"=220.08696}, {"X"=112.36232, "Y"=235.68697}, {"X"=112.695656, "Y"=251.28697}, {"X"=113.028984, "Y"=266.88696}, {"X"=113.36232, "Y"=282.48697}, {"X"=113.695656, "Y"=298.08698}, {"X"=124.260864, "Y"=63.782608}, {"X"=124.5942, "Y"=79.38261}, {"X"=124.927536, "Y"=94.982605}, {"X"=125.26087, "Y"=110.58261}, {"X"=125.5942, "Y"=126.18261}, {"X"=125.927536, "Y"=141.78261}, {"X"=126.26087, "Y"=157.38261}, {"X"=126.5942, "Y"=172.9826}, {"X"=126.927536, "Y"=188.58261}, {"X"=127.26087, "Y"=204.18262}, {"X"=127.5942, "Y"=219.78261}, {"X"=127.927536, "Y"=235.38261}, {"X"=128.26086, "Y"=250.98262}, {"X"=128.59421, "Y"=266.5826}, {"X"=128.92754, "Y"=282.18262}, {"X"=129.26086, "Y"=297.7826}, {"X"=139.82608, "Y"=63.47826}, {"X"=140.15942, "Y"=79.07826}, {"X"=140.49275, "Y"=94.67826}, {"X"=140.8261, "Y"=110.27826}, {"X"=141.15942, "Y"=125.878265}, {"X"=141.49275, "Y"=141.47827}, {"X"=141.8261, "Y"=157.07828}, {"X"=142.15942, "Y"=172.67827}, {"X"=142.49275, "Y"=188.27826}, {"X"=142.8261, "Y"=203.87827}, {"X"=143.15942, "Y"=219.47826}, {"X"=143.49275, "Y"=235.07826}, {"X"=143.8261, "Y"=250.67827}, {"X"=144.15942, "Y"=266.27826}, {"X"=144.49275, "Y"=281.87827}, {"X"=144.8261, "Y"=297.47827}, {"X"=155.3913, "Y"=63.173912}, {"X"=155.72464, "Y"=78.77391}, {"X"=156.05797, "Y"=94.37392}, {"X"=156.39131, "Y"=109.973915}, {"X"=156.72464, "Y"=125.57391}, {"X"=157.05797, "Y"=141.17392}, {"X"=157.39131, "Y"=156.77393}, {"X"=157.72464, "Y"=172.37392}, {"X"=158.05797, "Y"=187.9739}, {"X"=158.39131, "Y"=203.57393}, {"X"=158.72464, "Y"=219.17392}, {"X"=159.05797, "Y"=234.77393}, {"X"=159.39131, "Y"=250.37393}, {"X"=159.72464, "Y"=265.97394}, {"X"=160.05797, "Y"=281.5739}, {"X"=160.39131, "Y"=297.17392}, {"X"=170.95651, "Y"=62.869564}, {"X"=171.28986, "Y"=78.46957}, {"X"=171.62318, "Y"=94.069565}, {"X"=171.95653, "Y"=109.66957}, {"X"=172.28986, "Y"=125.26956}, {"X"=172.62318, "Y"=140.86957}, {"X"=172.95653, "Y"=156.46957}, {"X"=173.28986, "Y"=172.06958}, {"X"=173.62318, "Y"=187.66957}, {"X"=173.95653, "Y"=203.26958}, {"X"=174.28986, "Y"=218.86957}, {"X"=174.62318, "Y"=234.46957}, {"X"=174.95653, "Y"=250.06958}, {"X"=175.28986, "Y"=265.66956}, {"X"=175.62318, "Y"=281.2696}, {"X"=175.95653, "Y"=296.86957}, {"X"=186.52173, "Y"=62.565216}, {"X"=186.85507, "Y"=78.16522}, {"X"=187.1884, "Y"=93.76522}, {"X"=187.52174, "Y"=109.36522}, {"X"=187.85507, "Y"=124.96522}, {"X"=188.1884, "Y"=140.56522}, {"X"=188.52174, "Y"=156.16522}, {"X"=188.85507, "Y"=171.76523}, {"X"=189.1884, "Y"=187.36522}, {"X"=189.52174, "Y"=202.96523}, {"X"=189.85507, "Y"=218.56522}, {"X"=190.1884, "Y"=234.16522}, {"X"=190.52174, "Y"=249.76523}, {"X"=190.85507, "Y"=265.36523}, {"X"=191.1884, "Y"=280.9652}, {"X"=191.52174, "Y"=296.56522}, {"X"=202.08696, "Y"=62.260868}, {"X"=202.42029, "Y"=77.86087}, {"X"=202.75363, "Y"=93.46087}, {"X"=203.08696, "Y"=109.06087}, {"X"=203.42029, "Y"=124.66087}, {"X"=203.75363, "Y"=140.26086}, {"X"=204.08696, "Y"=155.86087}, {"X"=204.42029, "Y"=171.46088}, {"X"=204.75363, "Y"=187.06088}, {"X"=205.08696, "Y"=202.66087}, {"X"=205.42029, "Y"=218.26086}, {"X"=205.75363, "Y"=233.86087}, {"X"=206.08696, "Y"=249.46088}, {"X"=206.42029, "Y"=265.06085}, {"X"=206.75363, "Y"=280.6609}, {"X"=207.08696, "Y"=296.26086}, {"X"=217.65218, "Y"=61.95652}, {"X"=217.9855, "Y"=77.55652}, {"X"=218.31885, "Y"=93.156525}, {"X"=218.65218, "Y"=108.75652}, {"X"=218.9855, "Y"=124.35652}, {"X"=219.31885, "Y"=139.95651}, {"X"=219.65218, "Y"=155.55652}, {"X"=219.9855, "Y"=171.15652}, {"X"=220.31885, "Y"=186.75653}, {"X"=220.65218, "Y"=202.35654}, {"X"=220.9855, "Y"=217.95653}, {"X"=221.31885, "Y"=233.55653}, {"X"=221.65218, "Y"=249.15654}, {"X"=221.9855, "Y"=264.75653}, {"X"=222.31885, "Y"=280.35654}, {"X"=222.65218, "Y"=295.95654}, {"X"=233.21739, "Y"=61.652176}, {"X"=233.55072, "Y"=77.252174}, {"X"=233.88406, "Y"=92.85217}, {"X"=234.21739, "Y"=108.45218}, {"X"=234.55072, "Y"=124.05218}, {"X"=234.88406, "Y"=139.65218}, {"X"=235.21739, "Y"=155.25218}, {"X"=235.55072, "Y"=170.85217}, {"X"=235.88406, "Y"=186.45218}, {"X"=236.21739, "Y"=202.05219}, {"X"=236.55072, "Y"=217.65218}, {"X"=236.88406, "Y"=233.25218}, {"X"=237.21739, "Y"=248.85219}, {"X"=237.55072, "Y"=264.45218}, {"X"=237.88406, "Y"=280.0522}, {"X"=238.21739, "Y"=295.65216}, {"X"=248.78261, "Y"=61.347828}, {"X"=249.11594, "Y"=76.94783}, {"X"=249.44928, "Y"=92.54783}, {"X"=249.78261, "Y"=108.14783}, {"X"=250.11594, "Y"=123.74783}, {"X"=250.44928, "Y"=139.34782}, {"X"=250.78261, "Y"=154.94783}, {"X"=251.11594, "Y"=170.54782}, {"X"=251.44928, "Y"=186.14783}, {"X"=251.78261, "Y"=201.74783}, {"X"=252.11594, "Y"=217.34782}, {"X"=252.44928, "Y"=232.94783}, {"X"=252.78261, "Y"=248.54784}, {"X"=253.11594, "Y"=264.14783}, {"X"=253.44928, "Y"=279.74783}, {"X"=253.78261, "Y"=295.34784}, {"X"=264.34784, "Y"=61.04348}, {"X"=264.68115, "Y"=76.64348}, {"X"=265.0145, "Y"=92.24348}, {"X"=265.34784, "Y"=107.84348}, {"X"=265.68115, "Y"=123.44348}, {"X"=266.0145, "Y"=139.04349}, {"X"=266.34784, "Y"=154.6435}, {"X"=266.68115, "Y"=170.24348}, {"X"=267.0145, "Y"=185.84348}, {"X"=267.34784, "Y"=201.44348}, {"X"=267.68115, "Y"=217.04347}, {"X"=268.0145, "Y"=232.64348}, {"X"=268.34784, "Y"=248.24348}, {"X"=268.68115, "Y"=263.84348}, {"X"=269.0145, "Y"=279.44348}, {"X"=269.34784, "Y"=295.04346}, {"X"=279.91302, "Y"=60.739132}, {"X"=280.24637, "Y"=76.33913}, {"X"=280.5797, "Y"=91.93913}, {"X"=280.91306, "Y"=107.53914}, {"X"=281.24637, "Y"=123.13913}, {"X"=281.5797, "Y"=138.73914}, {"X"=281.91306, "Y"=154.33914}, {"X"=282.24637, "Y"=169.93913}, {"X"=282.5797, "Y"=185.53912}, {"X"=282.91306, "Y"=201.13914}, {"X"=283.24637, "Y"=216.73914}, {"X"=283.5797, "Y"=232.33914}, {"X"=283.91306, "Y"=247.93915}, {"X"=284.24637, "Y"=263.53912}, {"X"=284.5797, "Y"=279.13916}, {"X"=284.91306, "Y"=294.73914}, {"X"=295.47827, "Y"=60.434784}, {"X"=295.81158, "Y"=76.03478}, {"X"=296.14493, "Y"=91.63478}, {"X"=296.47827, "Y"=107.23479}, {"X"=296.81158, "Y"=122.834785}, {"X"=297.14493, "Y"=138.43478}, {"X"=297.47827, "Y"=154.03479}, {"X"=297.81158, "Y"=169.6348}, {"X"=298.14493, "Y"=185.23479}, {"X"=298.47827, "Y"=200.8348}, {"X"=298.81158, "Y"=216.43478}, {"X"=299.14493, "Y"=232.03479}, {"X"=299.47827, "Y"=247.6348}, {"X"=299.81158, "Y"=263.2348}, {"X"=300.14493, "Y"=278.83478}, {"X"=300.47827, "Y"=294.43478}, {"X"=311.04346, "Y"=60.130436}, {"X"=311.3768, "Y"=75.73044}, {"X"=311.71014, "Y"=91.33044}, {"X"=312.0435, "Y"=106.930435}, {"X"=312.3768, "Y"=122.53044}, {"X"=312.71014, "Y"=138.13043}, {"X"=313.0435, "Y"=153.73044}, {"X"=313.3768, "Y"=169.33044}, {"X"=313.71014, "Y"=184.93044}, {"X"=314.0435, "Y"=200.53044}, {"X"=314.3768, "Y"=216.13043}, {"X"=314.71014, "Y"=231.73044}, {"X"=315.0435, "Y"=247.33044}, {"X"=315.3768, "Y"=262.93042}, {"X"=315.71014, "Y"=278.53046}, {"X"=316.0435, "Y"=294.13043}, {"X"=326.6087, "Y"=59.826088}, {"X"=326.94205, "Y"=75.42609}, {"X"=327.27536, "Y"=91.02609}, {"X"=327.6087, "Y"=106.62609}, {"X"=327.94205, "Y"=122.22609}, {"X"=328.27536, "Y"=137.82608}, {"X"=328.6087, "Y"=153.42609}, {"X"=328.94205, "Y"=169.0261}, {"X"=329.27536, "Y"=184.6261}, {"X"=329.6087, "Y"=200.22609}, {"X"=329.94205, "Y"=215.82608}, {"X"=330.27536, "Y"=231.42609}, {"X"=330.6087, "Y"=247.0261}, {"X"=330.94205, "Y"=262.6261}, {"X"=331.27536, "Y"=278.22607}, {"X"=331.6087, "Y"=293.82608}, {"X"=342.17392, "Y"=59.52174}, {"X"=342.50726, "Y"=75.12174}, {"X"=342.84058, "Y"=90.72174}, {"X"=343.17392, "Y"=106.32175}, {"X"=343.50726, "Y"=121.92174}, {"X"=343.84058, "Y"=137.52173}, {"X"=344.17392, "Y"=153.12173}, {"X"=344.50726, "Y"=168.72174}, {"X"=344.84058, "Y"=184.32175}, {"X"=345.17392, "Y"=199.92175}, {"X"=345.50726, "Y"=215.52174}, {"X"=345.84058, "Y"=231.12175}, {"X"=346.17392, "Y"=246.72176}, {"X"=346.50726, "Y"=262.32175}, {"X"=346.84058, "Y"=277.92175}, {"X"=347.17392, "Y"=293.52173}, {"X"=357.73914, "Y"=59.217392}, {"X"=358.07248, "Y"=74.81739}, {"X"=358.4058, "Y"=90.41739}, {"X"=358.73914, "Y"=106.017395}, {"X"=359.07248, "Y"=121.61739}, {"X"=359.4058, "Y"=137.21739}, {"X"=359.73914, "Y"=152.8174}, {"X"=360.07248, "Y"=168.41739}, {"X"=360.4058, "Y"=184.0174}, {"X"=360.73914, "Y"=199.6174}, {"X"=361.07248, "Y"=215.21739}, {"X"=361.4058, "Y"=230.8174}, {"X"=361.73914, "Y"=246.4174}, {"X"=362.07248, "Y"=262.0174}, {"X"=362.4058, "Y"=277.6174}, {"X"=362.73914, "Y"=293.2174}, {"X"=373.30435, "Y"=58.913044}, {"X"=373.6377, "Y"=74.51305}, {"X"=373.971, "Y"=90.113045}, {"X"=374.30435, "Y"=105.71304}, {"X"=374.6377, "Y"=121.31305}, {"X"=374.971, "Y"=136.91304}, {"X"=375.30435, "Y"=152.51305}, {"X"=375.6377, "Y"=168.11305}, {"X"=375.971, "Y"=183.71304}, {"X"=376.30435, "Y"=199.31305}, {"X"=376.6377, "Y"=214.91304}, {"X"=376.971, "Y"=230.51305}, {"X"=377.30435, "Y"=246.11305}, {"X"=377.6377, "Y"=261.71304}, {"X"=377.971, "Y"=277.31305}, {"X"=378.30435, "Y"=292.91302}, {"X"=388.86957, "Y"=58.608696}, {"X"=389.2029, "Y"=74.208694}, {"X"=389.53622, "Y"=89.8087}, {"X"=389.86957, "Y"=105.4087}, {"X"=390.2029, "Y"=121.0087}, {"X"=390.53622, "Y"=136.6087}, {"X"=390.86957, "Y"=152.20871}, {"X"=391.2029, "Y"=167.8087}, {"X"=391.53622, "Y"=183.40869}, {"X"=391.86957, "Y"=199.0087}, {"X"=392.2029, "Y"=214.6087}, {"X"=392.53622, "Y"=230.20871}, {"X"=392.86957, "Y"=245.80872}, {"X"=393.2029, "Y"=261.4087}, {"X"=393.53622, "Y"=277.0087}, {"X"=393.86957, "Y"=292.6087}, {"X"=404.43478, "Y"=58.304348}, {"X"=404.76813, "Y"=73.90435}, {"X"=405.10144, "Y"=89.50435}, {"X"=405.43478, "Y"=105.104355}, {"X"=405.76813, "Y"=120.704346}, {"X"=406.10144, "Y"=136.30435}, {"X"=406.43478, "Y"=151.90436}, {"X"=406.76813, "Y"=167.50435}, {"X"=407.10144, "Y"=183.10435}, {"X"=407.43478, "Y"=198.70436}, {"X"=407.76813, "Y"=214.30435}, {"X"=408.10144, "Y"=229.90436}, {"X"=408.43478, "Y"=245.50436}, {"X"=408.76813, "Y"=261.10437}, {"X"=409.10144, "Y"=276.70435}, {"X"=409.43478, "Y"=292.30435}, {"X"=420.0, "Y"=58.0}, {"X"=420.33334, "Y"=73.6}, {"X"=420.66666, "Y"=89.2}, {"X"=421.0, "Y"=104.8}, {"X"=421.33334, "Y"=120.4}, {"X"=421.66666, "Y"=136.0}, {"X"=422.0, "Y"=151.6}, {"X"=422.33334, "Y"=167.20001}, {"X"=422.66666, "Y"=182.8}, {"X"=423.0, "Y"=198.40001}, {"X"=423.33334, "Y"=214.0}, {"X"=423.66666, "Y"=229.6}, {"X"=424.0, "Y"=245.20001}, {"X"=424.33334, "Y"=260.8}, {"X"=424.66666, "Y"=276.40002}, {"X"=425.0, "Y"=292.0}] {"Y" format="%.2f"; "X" format="%.2f"}
  out "Image":T1(plugin-control)
  out "MeltTemp":dbl=-0.0558620689654958 caption="Melt temp" format="%.3g °C"
  out "FreezeTemp":dbl=-3.0582758620689106 caption="Froze at" format="%.3g °C"
  out "Title 2":string="Well Data" caption="Version"
  out "Well":string="L16"
  out "CurTemp":dbl=-0.9882758620689174 caption="Temp" format="%.3g °C"
  out "Contents":string="D, 1mg/ml Snomax in 1:1 MQ:D2O"
  out "Temps":dbl[][](graph)
  out "Temps single":dbl[](graph)
  out "Fraction Single":dbl[](graph)=[0.0, 0.0, 0.0, 0.0, 0.0, 0.0, 0.0, 0.0, 0.0, 0.0, 0.0, 0.0, 0.0, 0.0, 0.0, 0.0, 0.0, 0.0, 0.0, 0.0, 0.0, 0.0, 0.0, 0.0, 0.0, 0.0, 0.0, 0.0, 0.0, 0.0, 0.0, 0.0, 0.0, 0.0, 0.0, 0.0, 0.0, 0.0, 0.0, 0.0, 0.0, 0.0, 0.0, 0.0, 0.0, 0.0, 0.0, 0.0, 0.0, 0.0, 0.0, 0.0, 0.0, 0.0, 0.0, 0.0, 0.0, 0.0, 0.0, 0.0, 0.0, 0.0, 0.0, 0.0, 0.0, 0.0, 0.0, 0.0, 0.0, 0.0, 0.0, 0.0, 0.0, 0.0, 0.0, 0.0, 0.0, 0.0, 0.0, 0.0, 0.0, 0.0, 0.0, 0.0, 0.0, 0.0, 0.0, 0.0, 0.0, 0.0, 0.0, 0.0, 0.0, 0.0, 0.0, 0.0, 0.0, 0.05263157894736842, 0.28421052631578947, 0.5578947368421052, 0.7052631578947368, 0.7473684210526316, 0.7789473684210526, 0.7894736842105263, 0.8421052631578947, 0.8631578947368421, 0.8947368421052632, 0.9263157894736842, 0.9789473684210527, 0.9789473684210527, 0.9894736842105263, 1.0, 1.0, 1.0, 1.0, 1.0, 1.0, 1.0, 1.0, 1.0, 1.0, 1.0, 1.0, 1.0, 1.0, 1.0, 1.0, 1.0, 1.0, 1.0, 1.0, 1.0, 1.0, 1.0, 1.0, 1.0, 1.0, 1.0, 1.0, 1.0, 1.0, 1.0, 1.0, 1.0, 1.0, 1.0, 1.0, 1.0, 1.0, 1.0, 1.0, 1.0, 1.0, 1.0, 1.0, 1.0, 1.0, 1.0, 1.0, 1.0, 1.0, 1.0, 1.0, 1.0, 1.0, 1.0, 1.0, 1.0, 1.0, 1.0, 1.0, 1.0, 1.0, 1.0, 1.0, 1.0, 1.0, 1.0, 1.0, 1.0, 1.0, 1.0, 1.0, 1.0, 1.0, 1.0, 1.0, 1.0, 1.0, 1.0, 1.0, 1.0, 1.0, 1.0, 1.0, 1.0, 1.0, 1.0, 1.0, 1.0, 1.0, 1.0, 1.0, 1.0, 1.0, 1.0, 1.0, 1.0, 1.0, 1.0, 1.0, 1.0, 1.0, 1.0, 1.0, 1.0, 1.0, 1.0, 1.0, 1.0, 1.0, 1.0, 1.0, 1.0, 1.0, 1.0, 1.0, 1.0, 1.0, 1.0, 1.0, 1.0, 1.0, 1.0, 1.0, 1.0, 1.0, 1.0, 1.0, 1.0, 1.0, 1.0, 1.0, 1.0, 1.0, 1.0, 1.0, 1.0, 1.0, 1.0, 1.0, 1.0, 1.0, 1.0, 1.0, 1.0, 1.0, 1.0, 1.0, 1.0, 1.0, 1.0, 1.0, 1.0, 1.0, 1.0, 1.0, 1.0, 1.0, 1.0, 1.0, 1.0, 1.0, 1.0, 1.0, 1.0, 1.0, 1.0, 1.0, 1.0, 1.0, 1.0, 1.0, 1.0, 1.0, 1.0, 1.0, 1.0, 1.0, 1.0, 1.0, 1.0, 1.0, 1.0, 1.0, 1.0, 1.0, 1.0, 1.0, 1.0, 1.0, 1.0, 1.0, 1.0, 1.0, 1.0, 1.0, 1.0, 1.0, 1.0, 1.0, 1.0, 1.0, 1.0, 1.0, 1.0, 1.0, 1.0, 1.0, 1.0, 1.0, 1.0, 1.0, 1.0, 1.0, 1.0, 1.0, 1.0, 1.0, 1.0, 1.0, 1.0, 1.0, 1.0, 1.0, 1.0, 1.0, 1.0, 1.0, 1.0, 1.0, 1.0, 1.0, 1.0, 1.0, 1.0, 1.0, 1.0, 1.0, 1.0, 1.0, 1.0, 1.0, 1.0, 1.0, 1.0, 1.0, 1.0, 1.0, 1.0, 1.0, 1.0, 1.0, 1.0, 1.0, 1.0, 1.0, 1.0, 1.0, 1.0, 1.0, 1.0, 1.0, 1.0, 1.0, 1.0, 1.0, 1.0, 1.0, 1.0, 1.0, 1.0, 1.0, 1.0, 1.0, 1.0, 1.0, 1.0, 1.0, 1.0, 1.0, 1.0, 1.0, 1.0, 1.0, 1.0, 1.0, 1.0, 1.0, 1.0, 1.0, 1.0, 1.0, 1.0, 1.0, 1.0, 1.0, 1.0, 1.0, 1.0, 1.0, 1.0, 1.0, 1.0, 1.0, 1.0, 1.0, 1.0, 1.0, 1.0, 1.0, 1.0, 1.0, 1.0, 1.0, 1.0, 1.0, 1.0, 1.0, 1.0, 1.0, 1.0, 1.0, 1.0, 1.0, 1.0, 1.0, 1.0, 1.0, 1.0, 1.0, 1.0, 1.0, 1.0, 1.0, 1.0, 1.0, 1.0, 1.0, 1.0, 1.0, 1.0, 1.0, 1.0, 1.0, 1.0, 1.0, 1.0, 1.0, 1.0, 1.0, 1.0, 1.0, 1.0, 1.0, 1.0, 1.0, 1.0, 1.0, 1.0, 1.0, 1.0, 1.0, 1.0, 1.0, 1.0, 1.0, 1.0, 1.0, 1.0, 1.0, 1.0, 1.0, 1.0, 1.0, 1.0, 1.0, 1.0, 1.0, 1.0, 1.0, 1.0, 1.0, 1.0, 1.0, 1.0, 1.0, 1.0, 1.0, 1.0, 1.0, 1.0, 1.0, 1.0, 1.0, 1.0, 1.0, 1.0, 1.0, 1.0, 1.0, 1.0, 1.0, 1.0, 1.0, 1.0, 1.0, 1.0, 1.0, 1.0, 1.0, 1.0, 1.0, 1.0, 1.0, 1.0, 1.0, 1.0]
  out "FrozenFractionGraph":dbl[][](graph)
  out "Temps single grad":dbl[](graph)
  out "Temps grads":dbl[][](graph)
  # "hints: \nUse the Mouse Wheel to zoom in and out"
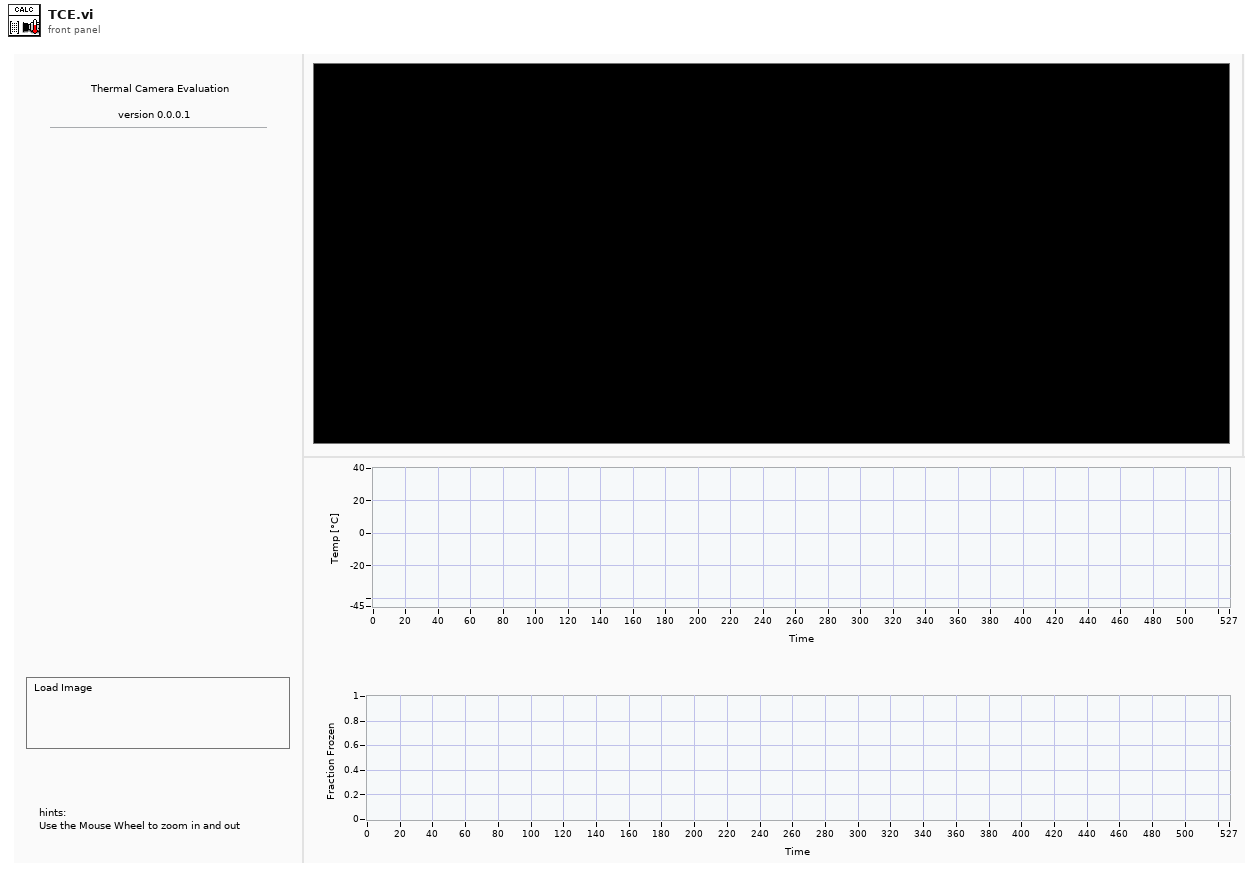
[diagram p1: front panel]
types:
  T1 = typedef "IMAQ Image.ctl" = refnum<image>
  T2 = typedef "IMAQ Point" = cluster{"X":sgl, "Y":sgl}
  T3 = enum32{"Invalid", "Standard", "Closed", "Hidden", "Minimized", "Maximized"}
  T4 = enum32{"invalid app kind", "Development System", "Run Time System", "Student Edition", "Embedded LabVIEW", "Evaluation", "Custom"}
  T5 = typedef "DataCluster_TCAL.ctl" = cluster{"Core":cluster{"Current VI Reference":refnum<vi>, "Close Panel on Exit?":bool}, "Image Out":T1, "State":i32, "Points":cluster{"Top Left":T2, "Top Right":T2, "Bottom Left":T2, "Bottom Right":T2, "x space 2":dbl, "y space 2":sgl, "x_space":sgl, "y_space":sgl, "Pixels":cluster{"X":i32, "Y":i32}[][], "Fixpoint":T2}, "img_array":T1[], "Temps":dbl[], "Temps_Array":dbl[][], "Scan Area":dbl, "Fixpoint Area":dbl, "Config":T6, "PCR Size":u16}
  T6 = typedef "TCE_Config.ctl" = cluster{"Freezing":cluster{"Cutoff":dbl}}
  T7 = cluster{"Global Rectangle":i32[], "Contours":cluster{"Contour Type":u32, "ROI Type":u32, "Points":i32[]}[]}
  T8 = enum8{"Enabled", "Disabled", "Disabled and Grayed Out"}
  T9 = cluster{"Desired Font (Application)":enum16{"User-specified Font", "Application Font", "System Font", "Dialog Font"}, "[User-specified Font]":cluster{"Font Name":string, "Size":i16, "Strikeout?":bool, "Italic?":bool, "Underline?":bool, "Outline?":bool, "Shadow?":bool, "Bold?":bool, "Rotation Angle":dbl}, "Horizontal Alignment":i16, "Vertical Alignment":i16}
  T10 = typedef "ROI Descriptor" = cluster{"Global Rectangle":i32[], "Contours":cluster{"ID":enum32{"External", "Internal"}, "Type":u32, "Coordinates":i32[]}[]}
  T11 = cluster{"Current VI Reference":refnum<vi>, "Close Panel on Exit?":bool}
  T12 = typedef "Image Type" = u32
  T13 = cluster{"Top Left":T2, "Top Right":T2, "Bottom Left":T2, "Bottom Right":T2, "x space 2":dbl, "y space 2":sgl, "x_space":sgl, "y_space":sgl, "Pixels":cluster{"X":i32, "Y":i32}[][], "Fixpoint":T2}
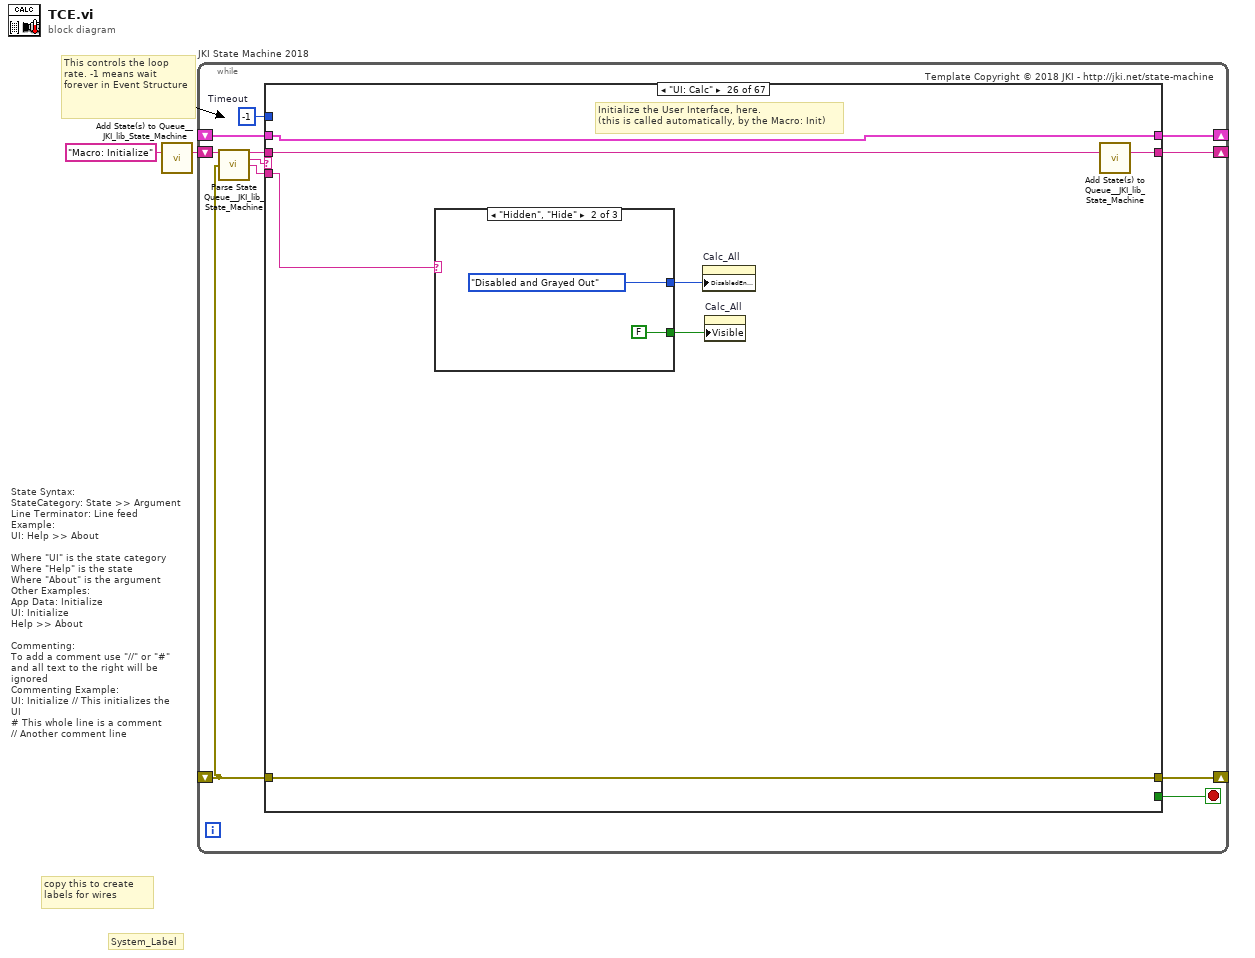
[diagram p0: block diagram]
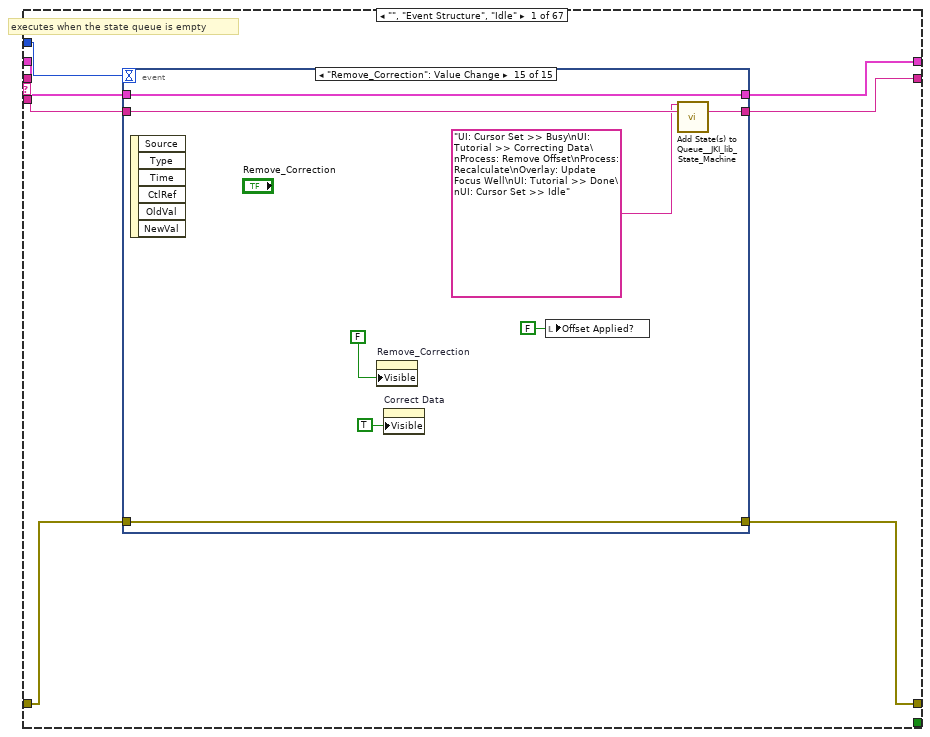
[diagram p2: hidden frame]
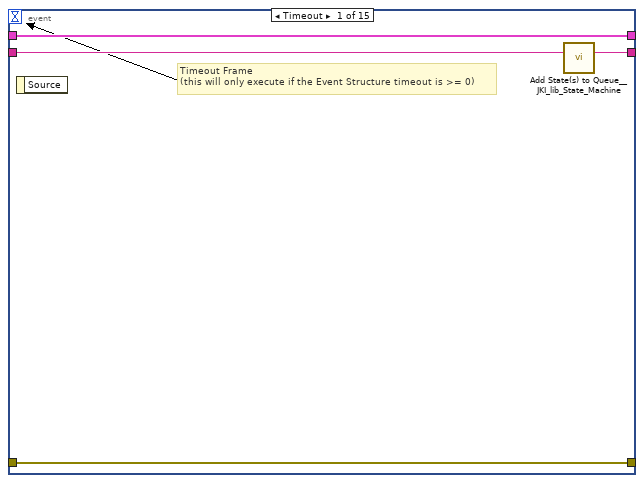
[diagram p3: hidden frame]
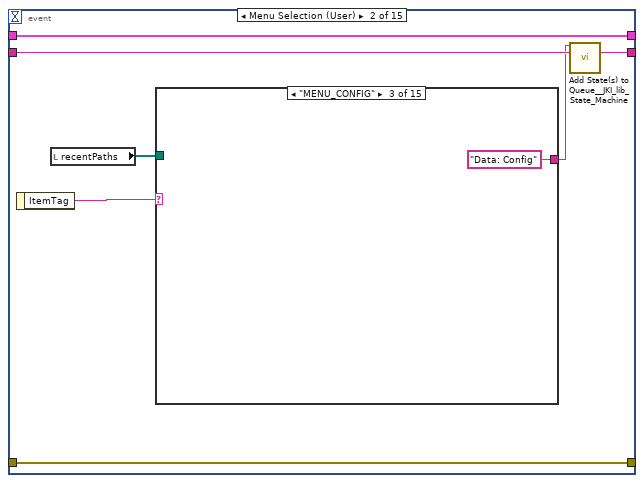
[diagram p4: hidden frame]
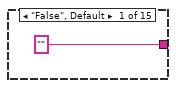
[diagram p5: hidden frame]
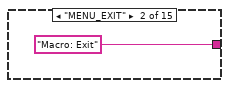
[diagram p6: hidden frame]
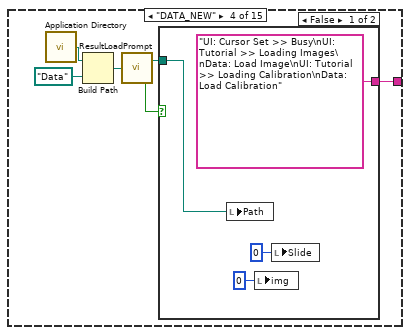
[diagram p7: hidden frame]
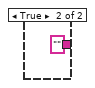
[diagram p8: hidden frame]
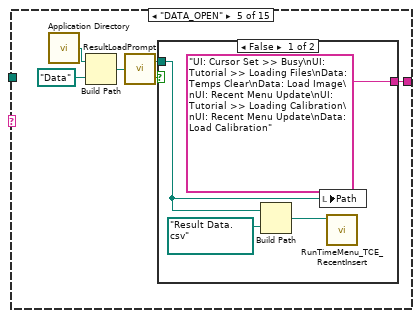
[diagram p9: hidden frame]
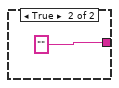
[diagram p10: hidden frame]
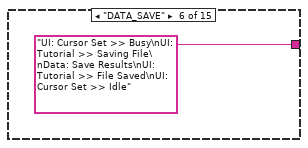
[diagram p11: hidden frame]
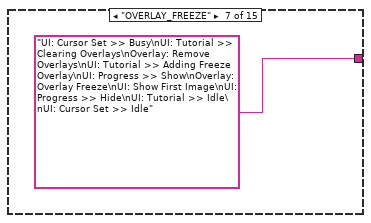
[diagram p12: hidden frame]
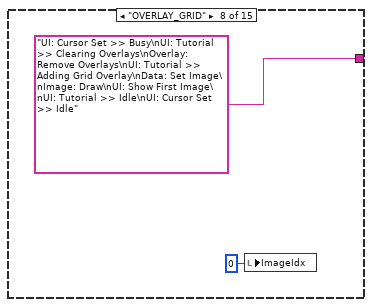
[diagram p13: hidden frame]
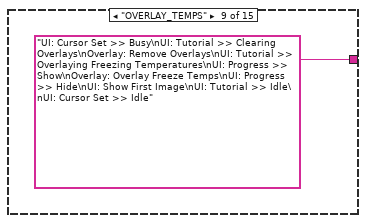
[diagram p14: hidden frame]
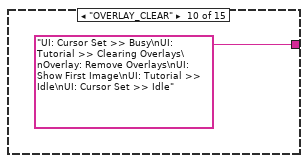
[diagram p15: hidden frame]
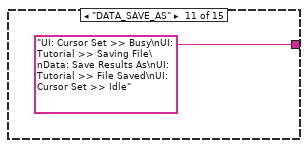
[diagram p16: hidden frame]
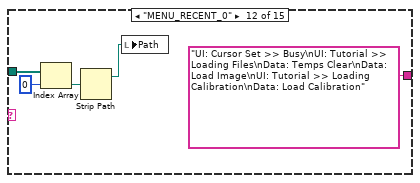
[diagram p17: hidden frame]
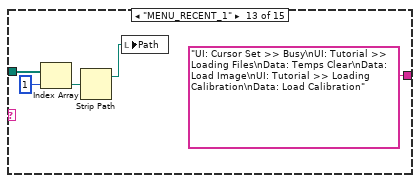
[diagram p18: hidden frame]
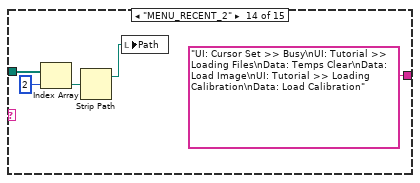
[diagram p19: hidden frame]
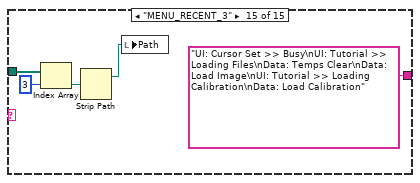
[diagram p20: hidden frame]
diagram:
  # "State Syntax:\nStateCategory: State >> Argument\nLine Terminator: Line feed\nExample:\nUI: Help >> About\n\nWhere \"UI\" is the state category\nWhere \"Help\" is the state\nWhere \"About\" is the argument\nOther Examples:\nApp Data: Initialize\nUI: Initialize\nHelp >> About\n\nCommenting:\nTo add a comment use \"//\" or \"#\" and all text to the right will be ignored\nCommenting Example:\nUI: Initialize // This initializes the UI\n# This whole line is a comment\n// Another comment line"
  # "copy this to create labels for wires"
  # "This controls the loop rate. -1 means wait forever in Event Structure"
  # "System_Label"
  n1 = call <vilib>:"Add State(s) to Queue__JKI_lib_State_Machine.vi"("State(s) in (\"\")"="Macro: Initialize") -> ("States Out"=w2:string)  [unwired: 14 in]
  n2 = while "JKI State Machine 2018" {
    shift-right: [w6] -> _
    shift-left: _ -> [w5]
    shift-right: [w9] -> _
    shift-left: _ -> [w3]
    shift-right: [w8] -> _
    shift-left: w2 -> [w10]
    stop <- w7 stop-if-true
    w4 = -1  # Timeout
    # "Template Copyright © 2018 JKI - http://jki.net/state-machine"
    n3 = call <vilib>:"Parse State Queue__JKI_lib_State_Machine.vi"("State Queue"=w10, "Error In (no error)"=w3) -> ("Remaining States"=w12:string, "Current State"=w13:string, "Arguments"=w11:string)  [unwired: 11 in]
    n4 = case shown="\"UI: Calc\"" w13 {
      selector: w13 -> [_ _ w200 _ _ _ _ _ _ _ _ _ _ _ _ _ _ _ _ _ _ _ _ _ _ _ _ _ _ _ _ _ _ _ _ _ _ _ _ _ _ _ _ _ _ _ _ _ _ _ _ _ _ _ _ _ _ _ _ _ _ _ _ _ _ _ _]
      tunnel: w12 -> [w20 w199 w204 w223 w229 w234 w238 w254 w263 w271 w287 w342 w370 w400 w405 w412 w419 w435 w486 w515 w550 w558 w566 w573 w578 w585 w597 w609 w619 w629 w640 w651 w720 w725 w735 w739 w744 w749 w766 w788 w832 w861 w885 w910 w931 w939 w946 w956 w963 w968 w973 w982 w1002 w1019 w1085 w1111 w1131 w1149 w1165 w1174 w1183 w1195 w1204 w1244 w1288 w1323 w1339]
      tunnel: w11 -> [_ _ _ _ _ _ _ _ _ _ _ _ _ _ _ _ _ _ _ _ _ w554 _ _ w574 w581 w592 w605 w615 w625 w636 w645 _ _ _ _ _ _ _ _ _ _ _ _ _ _ _ _ _ _ _ _ _ w1017 _ _ _ _ _ _ _ _ _ _ _ _ _]
      tunnel: w5 -> [w18 w196 w202 w216 w226 w232 w235 _ w261 w268 w274 w339 w363 w397 w401 w409 w416 w433 w477 w512 w548 w556 w564 w570 w576 w583 w595 w607 w617 w627 w638 w647 w717 w722 w732 w736 w741 w746 w755 w772 w818 w858 w876 w907 w928 w936 w943 w953 w960 w965 w970 w979 w983 w1015 w1072 w1102 w1122 w1140 w1154 w1172 w1178 w1192 w1201 w1241 w1283 w1320 w1330]
      tunnel: [w17 w197 w206 w220 errorcluster {"status"=FALSE, "code"=0, "source"=""} ("error out") w231 w236 w243 w260 w269 w276 w340 w368 w394 w403 w410 w417 w420 w471 w513 w547 w555 w563 w571 w575 w582 w593 w606 w616 w626 w637 w648 w718 w723 w733 w737 w742 w747 w764 w786 w830 w859 w883 w908 w929 w937 w944 w954 w961 w966 w971 w980 w1000 w1012 w1082 w1109 w1129 w1147 w1163 w1169 w1175 w1193 w1202 w1242 w1286 w1321 w1337] -> w9
      tunnel: w3 -> [w16 w197 w205 w220 w225 w231 w236 w243 w257 w269 w283 w340 w368 w394 w403 w410 w417 w420 w471 w513 w547 w555 w563 w571 w575 w582 w594 w606 w616 w626 w637 w649 w718 w723 w733 w737 w742 w747 w764 w786 w830 w859 w883 w908 w929 w937 w944 w954 w961 w966 w971 w980 w1000 w1013 w1082 w1109 w1129 w1147 w1163 w1170 w1177 w1193 w1202 w1242 w1286 w1321 w1337]
      tunnel: [w19 w198 w203 w222 w228 w233 w237 w253 w262 w270 w286 w341 w369 w399 w404 w411 w418 w434 w485 w514 w549 w557 w565 w572 w577 w584 w596 w608 w618 w628 w639 w650 w719 w724 w734 w738 w743 w748 w765 w787 w831 w860 w884 w909 w930 w938 w945 w955 w962 w967 w972 w981 w1001 w1018 w1084 w1110 w1130 w1148 w1164 w1173 w1182 w1194 w1203 w1243 w1287 w1322 w1338] -> w8
      tunnel: [_ _ _ _ _ TRUE _ _ _ _ _ _ _ _ _ _ _ _ _ _ _ _ _ _ _ _ _ _ _ _ _ _ _ _ _ _ _ _ _ _ _ _ _ _ _ _ _ _ _ _ _ _ _ _ _ _ _ _ _ _ _ _ _ _ _ _ _] -> w7
      tunnel: [w15 w196 w202 w221 w226 w232 w235 w252 w261 w267 w285 w339 w362 w398 w401 w409 w415 w433 w477 w512 w548 w556 w564 w570 w576 w583 w595 w607 w617 w627 w638 w647 w717 w722 w732 w736 w741 w746 w755 w771 w818 w858 w876 w907 w928 w936 w943 w953 w960 w965 w970 w979 w983 w1015 w1071 w1101 w1121 w1139 w1154 w1172 w1178 w1192 w1201 w1241 w1283 w1320 w1330] -> w6
      tunnel: w4 -> [w14 _ _ _ _ _ _ _ _ _ _ _ _ _ _ _ _ _ _ _ _ _ _ _ _ _ _ _ _ _ _ _ _ _ _ _ _ _ _ _ _ _ _ _ _ _ _ _ _ _ _ _ _ _ _ _ _ _ _ _ _ _ _ _ _ _ _]
      frame "", "Event Structure", "Idle" {
        # "executes when the state queue is empty"
        n5 = event shown="[14] \"Remove_Correction\": Value Change" {
          selector: _ -> [_ _ _ _ _ _ _ _ _ _ _ _ _ _ _]
          dyn-events: _ -> [_ _ _ _ _ _ _ _ _ _ _ _ _ _ _]
          timeout: w14 -> [_ _ _ _ _ _ _ _ _ _ _ _ _ _ _]
          tunnel: w20 -> [w24 w31 w87 w99 w109 w115 w124 w133 w142 w151 w160 w169 w179 w187 w195]
          tunnel: [w23 w30 w86 w98 w108 w114 w123 w132 w141 w150 w159 w168 w178 w186 w194] -> w19
          tunnel: w18 -> [w21 w28 w84 w96 w106 w112 w121 w130 w139 w148 w157 w166 w176 w184 w192]
          tunnel: [w22 w29 w85 w97 w107 w113 w122 w131 w140 w149 w158 w167 w177 w185 w193] -> w17
          tunnel: w16 -> [w22 w29 w85 w97 w107 w113 w122 w131 w140 w149 w158 w167 w177 w185 w193]
          tunnel: [w21 w28 w84 w96 w106 w112 w121 w130 w139 w148 w157 w166 w176 w184 w192] -> w15
          event Timeout {
            # "Timeout Frame\n(this will only execute if the Event Structure timeout is >= 0)"
            n6 = event-data() -> ()  [unwired: 1 in, 1 out]
            n7 = call <vilib>:"Add State(s) to Queue__JKI_lib_State_Machine.vi"("State(s) in (\"\")"=w24) -> ("States Out"=w23:string)  [unwired: 14 in]
          }
          event Menu Selection (User) {
            n8 = event-data() -> ("ItemTag"=w27:string)  [unwired: 1 in]
            n9 = local read "recentPaths"() -> (w25:path[])
            n10 = case shown="\"MENU_CONFIG\"" w27 {
              tunnel: ["" "Macro: Exit" "Data: Config" w40 w51 "UI: Cursor Set >> Busy\nUI: Tutorial >> Saving File\nData: Save Results\nUI: Tutorial >> File Saved\nUI: Cursor Set >> Idle" "UI: Cursor Set >> Busy\nUI: Tutorial >> Clearing Overlays\nOverlay: Remove Overlays\nUI: Tutorial >> Adding Freeze Overlay\nUI: Progress >> Show\nOverlay: Overlay Freeze\nUI: Show First Image\nUI: Progress >> Hide\nUI: Tutorial >> Idle\nUI: Cursor Set >> Idle" "UI: Cursor Set >> Busy\nUI: Tutorial >> Clearing Overlays\nOverlay: Remove Overlays\nUI: Tutorial >> Adding Grid Overlay\nData: Set Image\nImage: Draw\nUI: Show First Image\nUI: Tutorial >> Idle\nUI: Cursor Set >> Idle" "UI: Cursor Set >> Busy\nUI: Tutorial >> Clearing Overlays\nOverlay: Remove Overlays\nUI: Tutorial >> Overlaying Freezing Temperatures\nUI: Progress >> Show\nOverlay: Overlay Freeze Temps\nUI: Progress >> Hide\nUI: Show First Image\nUI: Tutorial >> Idle\nUI: Cursor Set >> Idle" "UI: Cursor Set >> Busy\nUI: Tutorial >> Clearing Overlays\nOverlay: Remove Overlays\nUI: Show First Image\nUI: Tutorial >> Idle\nUI: Cursor Set >> Idle" "UI: Cursor Set >> Busy\nUI: Tutorial >> Saving File\nData: Save Results As\nUI: Tutorial >> File Saved\nUI: Cursor Set >> Idle" "UI: Cursor Set >> Busy\nUI: Tutorial >> Loading Files\nData: Temps Clear\nData: Load Image\nUI: Tutorial >> Loading Calibration\nData: Load Calibration" "UI: Cursor Set >> Busy\nUI: Tutorial >> Loading Files\nData: Temps Clear\nData: Load Image\nUI: Tutorial >> Loading Calibration\nData: Load Calibration" "UI: Cursor Set >> Busy\nUI: Tutorial >> Loading Files\nData: Temps Clear\nData: Load Image\nUI: Tutorial >> Loading Calibration\nData: Load Calibration" "UI: Cursor Set >> Busy\nUI: Tutorial >> Loading Files\nData: Temps Clear\nData: Load Image\nUI: Tutorial >> Loading Calibration\nData: Load Calibration"] -> w26
              tunnel: w25 -> [_ _ _ _ _ _ _ _ _ _ _ w67 w72 w77 w82]
              frame "False", Default {
              }
              frame "MENU_EXIT" {
              }
              frame "MENU_CONFIG" {
              }
              frame "DATA_NEW" {
                n11 = call <vilib>:"Application Directory.vi"() -> ("Application Directory"=w39:path)
                n12 = Build Path(base path=w39, name or relative path=path "Data") -> (appended path=w38:path)
                n13 = call "ResultLoadPrompt.vi"("Path"=w38) -> ("selected path"=w35:path, "cancel?"=w36:bool)
                n14 = case shown="False" w36 {
                  tunnel: ["UI: Cursor Set >> Busy\nUI: Tutorial >> Loading Images\nData: Load Image\nUI: Tutorial >> Loading Calibration\nData: Load Calibration" ""] -> w40
                  tunnel: w35 -> [w41 _]
                  frame False {
                    n15 = local write "Path"(w41) -> ()
                    n16 = local write "img"(0 ("img")) -> ()
                    n17 = local write "Slide"(u8 0 ("Slide")) -> ()
                  }
                  frame True {
                  }
                }
              }
              frame "DATA_OPEN" {
                n18 = call <vilib>:"Application Directory.vi"() -> ("Application Directory"=w50:path)
                n19 = Build Path(base path=w50, name or relative path=path "Data") -> (appended path=w48:path)
                n20 = call "ResultLoadPrompt.vi"("Path"=w48) -> ("selected path"=w47:path, "cancel?"=w46:bool)
                n21 = case shown="False" w46 {
                  tunnel: ["UI: Cursor Set >> Busy\nUI: Tutorial >> Loading Files\nData: Temps Clear\nData: Load Image\nUI: Recent Menu Update\nUI: Tutorial >> Loading Calibration\nUI: Recent Menu Update\nData: Load Calibration" ""] -> w51
                  tunnel: w47 -> [w54 _]
                  frame False {
                    n22 = Build Path(base path=w54, name or relative path=path "Result Data.csv") -> (appended path=w52:path)
                    n23 = local write "Path"(w54) -> ()
                    n24 = call "RunTimeMenu_TCE_RecentInsert.vi"("NewPath"=w52) -> ()  [unwired: 11 in]
                  }
                  frame True {
                  }
                }
              }
              frame "DATA_SAVE" {
              }
              frame "OVERLAY_FREEZE" {
              }
              frame "OVERLAY_GRID" {
                n25 = local write "ImageIdx"(0 ("img")) -> ()
              }
              frame "OVERLAY_TEMPS" {
              }
              frame "OVERLAY_CLEAR" {
              }
              frame "DATA_SAVE_AS" {
              }
              frame "MENU_RECENT_0" {
                n26 = Index Array(array=w67, index=0) -> (element=w65:path)
                n27 = Strip Path(path=w65) -> (stripped path=w64:path)  [unwired: 1 out]
                n28 = local write "Path"(w64) -> ()
              }
              frame "MENU_RECENT_1" {
                n29 = Index Array(array=w72, index=1) -> (element=w70:path)
                n30 = Strip Path(path=w70) -> (stripped path=w69:path)  [unwired: 1 out]
                n31 = local write "Path"(w69) -> ()
              }
              frame "MENU_RECENT_2" {
                n32 = Index Array(array=w77, index=2) -> (element=w75:path)
                n33 = Strip Path(path=w75) -> (stripped path=w74:path)  [unwired: 1 out]
                n34 = local write "Path"(w74) -> ()
              }
              frame "MENU_RECENT_3" {
                n35 = Index Array(array=w82, index=3) -> (element=w80:path)
                n36 = Strip Path(path=w80) -> (stripped path=w79:path)  [unwired: 1 out]
                n37 = local write "Path"(w79) -> ()
              }
            }
            n38 = call <vilib>:"Add State(s) to Queue__JKI_lib_State_Machine.vi"("State(s) in Front (\"\")"=w26, "State(s) in (\"\")"=w31) -> ("States Out"=w30:string)  [unwired: 13 in]
          }
          event "Help": Value Change {
            # "Timeout Frame\n(this will only execute if the Event Structure timeout is >= 0)"
            n39 = event-data() -> ()  [unwired: 1 in, 6 out]
            n40 = call <vilib>:"Add State(s) to Queue__JKI_lib_State_Machine.vi"("State(s) in (\"\")"=w87) -> ("States Out"=w86:string)  [unwired: 14 in]
          }
          event "Image": Mouse Wheel {
            n41 = event-data() -> ("Delta"=w95:i32)  [unwired: 1 in, 1 out]
            n42 = property on="Image" class="ImageControl"() -> ("Last Mouse Position"=w89:cluster{"X":i32, "Y":i32}, "X Zoom"=w90:sgl)  [unwired: 2 in, 2 out]
            n43 = Greater Than 0?(x=w95) -> (x > 0?=w94:bool)
            n44 = Select(t=1.2, s=w94, f=0.8) -> (s? t:f=w91:dbl)
            n45 = Multiply(x=w91, y=w90) -> (x*y=w88:dbl)
            n46 = property on="Image" class="ImageControl"("X Zoom"=w88, "Y Zoom"=w88, "Image Center Position"=w89) -> ()  [unwired: 2 in, 2 out]
            n47 = call <vilib>:"Add State(s) to Queue__JKI_lib_State_Machine.vi"("State(s) in (\"\")"=w99) -> ("States Out"=w98:string)  [unwired: 14 in]
          }
          event "Image": Mouse Up {
            n48 = event-data() -> ()  [unwired: 1 in, 1 out]
            n49 = property on="Image" class="ImageControl"() -> ("Last Mouse Position"=w105:cluster{"X":i32, "Y":i32})  [unwired: 2 in, 2 out]
            n50 = local read "Temps"() -> (w100:dbl[][])
            n51 = local read "Points"() -> (w104:T2[])
            n52 = call "SingleWellUpdater.vi"("Temps"=w100, "Well Coordinates"=w104, "Last Mouse Position"=w105) -> ("Well idx"=w101:i32, "ROI Descriptor"=w102:T10, "State out"=w103:string)  [unwired: 6 in]
            n53 = property on="Image" class="ImageControl"("ROI"=w102) -> ()  [unwired: 2 in, 2 out]
            n54 = local write "Well"(w101) -> ()
            n55 = call <vilib>:"Add State(s) to Queue__JKI_lib_State_Machine.vi"("State(s) in Front (\"\")"=w103, "State(s) in (\"\")"=w109) -> ("States Out"=w108:string)  [unwired: 13 in]
          }
          event Panel Close? {
            # "Discard the event because we'll close the front panel ourselves in Macro: Exit"
            # "Close Panel button (pressed) Event\n(this executes Macro: Exit to terminate the VI)"
            n56 = event-data() -> ()  [unwired: 1 in, 1 out]
            n57 = call <vilib>:"Add State(s) to Queue__JKI_lib_State_Machine.vi"("State(s) in Front (\"\")"="Macro: Exit", "State(s) in (\"\")"=w115) -> ("States Out"=w114:string)  [unwired: 13 in]
            n58 = event-data("Discard?"=TRUE) -> ()  [unwired: 1 in, 1 out]
          }
          event "Temps single": Cursor Move {
            n59 = event-data() -> ()  [unwired: 1 in, 9 out]
            n60 = property on="Temps single" class="WFGraph (strict)"() -> ("Cursor.Cursor X"=w119:dbl)  [unwired: 2 in, 2 out]
            n61 = local read "maxSize"() -> (w118:i32)
            n62 = In Range and Coerce(upper limit=w118, x=w119, lower limit=0) -> (coerced(x)=w116:dbl)  [unwired: 1 out]
            n63 = local write "ImageIdx"(w116) -> ()
            n64 = call <vilib>:"Add State(s) to Queue__JKI_lib_State_Machine.vi"("State(s) in Front (\"\")"="Image: Set Cursors\nData: Set Image\nData: Show Img\nData: Update Well Temp", "State(s) in (\"\")"=w124) -> ("States Out"=w123:string)  [unwired: 13 in]
          }
          event "Temps": Cursor Move {
            n65 = event-data() -> ()  [unwired: 1 in, 1 out]
            n66 = property on="Temps" class="WFGraph (strict)"() -> ("Cursor.Cursor X"=w128:dbl)  [unwired: 2 in, 2 out]
            n67 = local read "maxSize"() -> (w126:i32)
            n68 = In Range and Coerce(upper limit=w126, x=w128, lower limit=0) -> (coerced(x)=w125:dbl)  [unwired: 1 out]
            n69 = local write "ImageIdx"(w125) -> ()
            n70 = call <vilib>:"Add State(s) to Queue__JKI_lib_State_Machine.vi"("State(s) in Front (\"\")"="Image: Set Cursors\nData: Set Image\nData: Show Img\nData: Update Well Temp", "State(s) in (\"\")"=w133) -> ("States Out"=w132:string)  [unwired: 13 in]
          }
          event "Temps single grad": Cursor Move {
            n71 = event-data() -> ()  [unwired: 1 in, 1 out]
            n72 = property on="Temps single grad" class="WFGraph (strict)"() -> ("Cursor.Cursor X"=w137:dbl)  [unwired: 2 in, 2 out]
            n73 = local read "maxSize"() -> (w135:i32)
            n74 = In Range and Coerce(upper limit=w135, x=w137, lower limit=0) -> (coerced(x)=w134:dbl)  [unwired: 1 out]
            n75 = local write "ImageIdx"(w134) -> ()
            n76 = call <vilib>:"Add State(s) to Queue__JKI_lib_State_Machine.vi"("State(s) in Front (\"\")"="Image: Set Cursors\nData: Set Image\nData: Show Img\nData: Update Well Temp", "State(s) in (\"\")"=w142) -> ("States Out"=w141:string)  [unwired: 13 in]
          }
          event "FrozenFractionGraph": Cursor Move {
            n77 = event-data() -> ()  [unwired: 1 in, 1 out]
            n78 = property on="FrozenFractionGraph" class="WFGraph (strict)"() -> ("Cursor.Cursor X"=w146:dbl)  [unwired: 2 in, 2 out]
            n79 = local read "maxSize"() -> (w144:i32)
            n80 = In Range and Coerce(upper limit=w144, x=w146, lower limit=0) -> (coerced(x)=w143:dbl)  [unwired: 1 out]
            n81 = local write "ImageIdx"(w143) -> ()
            n82 = call <vilib>:"Add State(s) to Queue__JKI_lib_State_Machine.vi"("State(s) in Front (\"\")"="Image: Set Cursors\nData: Set Image\nData: Show Img\nData: Update Well Temp", "State(s) in (\"\")"=w151) -> ("States Out"=w150:string)  [unwired: 13 in]
          }
          event "Fraction Single": Cursor Move {
            n83 = event-data() -> ()  [unwired: 1 in, 1 out]
            n84 = property on="Fraction Single" class="WFGraph (strict)"() -> ("Cursor.Cursor X"=w155:dbl)  [unwired: 2 in, 2 out]
            n85 = local read "maxSize"() -> (w153:i32)
            n86 = In Range and Coerce(upper limit=w153, x=w155, lower limit=0) -> (coerced(x)=w154:dbl)  [unwired: 1 out]
            n87 = local write "ImageIdx"(w154) -> ()
            n88 = call <vilib>:"Add State(s) to Queue__JKI_lib_State_Machine.vi"("State(s) in Front (\"\")"="Image: Set Cursors\nData: Set Image\nData: Show Img\nData: Update Well Temp", "State(s) in (\"\")"=w160) -> ("States Out"=w159:string)  [unwired: 13 in]
          }
          event "Temps grads": Value Change {
            n89 = event-data() -> ()  [unwired: 1 in, 1 out]
            n90 = property on="Temps grads" class="WFGraph (strict)"() -> ("Cursor.Cursor X"=w164:dbl)  [unwired: 2 in, 2 out]
            n91 = local read "maxSize"() -> (w163:i32)
            n92 = In Range and Coerce(upper limit=w163, x=w164, lower limit=0) -> (coerced(x)=w161:dbl)  [unwired: 1 out]
            n93 = local write "ImageIdx"(w161) -> ()
            n94 = call <vilib>:"Add State(s) to Queue__JKI_lib_State_Machine.vi"("State(s) in Front (\"\")"="Image: Set Cursors\nData: Set Image\nData: Show Img\nData: Update Well Temp", "State(s) in (\"\")"=w169) -> ("States Out"=w168:string)  [unwired: 13 in]
          }
          event "Calc_All": Value Change {
            w170 = FALSE ("Visible")
            w174 = u8 0 ("Slide")
            n95 = event-data() -> ()  [unwired: 1 in, 6 out]
            n96 = local write "ImageIdx"(w174) -> ()
            n97 = local write "img"(0 ("img")) -> ()
            n98 = local write "Slide"(w174) -> ()
            n99 = property on="Temps" class="WFGraph (strict)"("Visible"=TRUE) -> ()  [unwired: 2 in, 2 out]
            n100 = property on="Temps single" class="WFGraph (strict)"("Visible"=w170) -> ()  [unwired: 2 in, 2 out]
            n101 = property on="Temps single grad" class="WFGraph (strict)"("Visible"=w170) -> ()  [unwired: 2 in, 2 out]
            n102 = property on="Temp grads" class="WFGraph (strict)"("Visible"=w170) -> ()  [unwired: 2 in, 2 out]
            n103 = local write "Offset Applied?"(FALSE ("Offset Applied?")) -> ()
            n104 = call <vilib>:"Add State(s) to Queue__JKI_lib_State_Machine.vi"("State(s) in Front (\"\")"="Process: Calculate All", "State(s) in (\"\")"=w179) -> ("States Out"=w178:string)  [unwired: 13 in]
          }
          event "Correct Data": Value Change {
            n105 = event-data() -> ()  [unwired: 1 in, 6 out]
            n106 = property on="Correct Data" class="Bool"("Visible"=FALSE) -> ()  [unwired: 2 in, 2 out]
            n107 = property on="Remove_Correction" class="Bool"("Visible"=TRUE) -> ()  [unwired: 2 in, 2 out]
            n108 = call <vilib>:"Add State(s) to Queue__JKI_lib_State_Machine.vi"("State(s) in Front (\"\")"="UI: Cursor Set >> Busy\nUI: Tutorial >> Correcting Data\nProcess: Correct Offset\nProcess: Recalculate\nOverlay: Update Focus Well\nUI: Tutorial >> Done\nUI: Cursor Set >> Idle", "State(s) in (\"\")"=w187) -> ("States Out"=w186:string)  [unwired: 13 in]
            "Offset Applied?" <- TRUE ("Offset Applied?")
          }
          event "Remove_Correction": Value Change {
            n109 = event-data() -> ()  [unwired: 1 in, 6 out]
            n110 = property on="Remove_Correction" class="Bool"("Visible"=FALSE) -> ()  [unwired: 2 in, 2 out]
            n111 = property on="Correct Data" class="Bool"("Visible"=TRUE) -> ()  [unwired: 2 in, 2 out]
            n112 = local write "Offset Applied?"(FALSE ("Offset Applied?")) -> ()
            n113 = call <vilib>:"Add State(s) to Queue__JKI_lib_State_Machine.vi"("State(s) in Front (\"\")"="UI: Cursor Set >> Busy\nUI: Tutorial >> Correcting Data\nProcess: Remove Offset\nProcess: Recalculate\nOverlay: Update Focus Well\nUI: Tutorial >> Done\nUI: Cursor Set >> Idle", "State(s) in (\"\")"=w195) -> ("States Out"=w194:string)  [unwired: 13 in]
          }
        }
      }
      frame "---------- Core ----------" {
        # "Do not put any code in this frame.\n(it is a separator no-op)"
        n114 = call <vilib>:"Add State(s) to Queue__JKI_lib_State_Machine.vi"("State(s) in (\"\")"=w199) -> ("States Out"=w198:string)  [unwired: 14 in]
      }
      frame Default {
        w209 = 42 items=["No error", "Argument error", "Memory is full", "Out of zone", "End of file", "File already open", "Generic file I/O error", "File not found", "File permission error", "Disk is full", "Duplicate path", "Too many files open", "System feature not enabled", "Resource file not found", "Cannot add resource", "Resource not found", "Image not found", "Image memory error", "Pen does not exist", "Config type invalid", "Config token not found", "Config parse error", "Config memory error", "Bad external code format", "Bad external code offset", "External code not present", "Null window", "Destroy window error", "Null menu", "Print aborted", "Bad print record", "Print driver error", "Windows error during printing", "Memory error during printing", "Print dialog error", "Generic print error", "Invalid device refnum", "Device not found", "Device parameter error", "Device unit error", "Cannot open device", "Device call aborted", "Generic error", "Cancelled by user", "Object ID too low", "Object ID too high", "Object not in heap", "Unknown heap", "Unknown object (invalid DefProc)", "Unknown object (DefProc not in table)", "Message out of range", "Invalid (null) method", "Unknown message", "Manager call not supported", "Bad address", "Network operation in progress", "Network operation timed out", "Connection is busy", "Network attribute not supported", "Network error", "Address in use", "System out of memory", "Connection aborted", "Connection refused", "Not connected", "Already connected", "Connection closed", "Initialization error (interapplication manager)", "Bad occurrence", "Wait on unbound occurrence handler", "Occurrence queue overflow", "Datalog type conflict", "Unused", "Unrecognized type (interapplication manager)", "Memory corrupt", "Failed to make temporary DLL", "Old CIN version", "Drag socket not found", "Failed to load drop-object", "Failed to register OLE object", "Failed to release OLE object", "Format specifier type mismatch", "Unknown format specifier", "Too few format specifiers", "Too many format specifiers", "Scan failed", "Newer CIN version", "Error converting to variant", "Runtime menu error", "Password tampered", "Variant attribute not found", "Incompatible variant data type", "Event data is not available", "Event Store is not present", "Occurrence is not found", "Event Queue is not created", "Event info is not available", "Refnum passed is NULL", "Error retrieving Class GUID", "Error retrieving CoClass GUID", "Error retrieving TypeLib GUID.", "Bad built application magic bytes.", "Specific driver is different from the specific driver associated with the Logical Name.", "There is no session opened to the class driver.", "Max Error", "MAX - Error with config objects", "MAX - Error loading configuration", "MAX - Group not supported"]
        # "Current State"
        # "Do not delete, rename, or modify this frame.\n(this is used to capture unhandled states and typos)"
        # "Handle mistyped state name (developer tool)"
        n115 = Format Into String(format string="Software Exception: Unhandled State \"%s\"." ("message"), error in=w205, w200) -> (resulting string=w208:string, error out=w207:errorcluster)  [unwired: 1 in]
        n116 = call <vilib>:"Error Cluster From Error Code.vi"("show call chain? (False)"=TRUE, "error in (no error)"=w207, "error message (\"\")"=w208, "error code (0)"=w209) -> ("error out"=w206:errorcluster)  [unwired: 5 in]
        n117 = call <vilib>:"Add State(s) to Queue__JKI_lib_State_Machine.vi"("State(s) in (\"\")"=w204) -> ("States Out"=w203:string)  [unwired: 14 in]
      }
      frame "Initialize Core Data" {
        # "Do not delete, rename, or modify this frame.\n(this is used to determine panel behavior on exit)"
        # "originally closed?"
        # "exe?"
        # "If panel starts closed or is an EXE, then close it when we exit"
        n118 = property class="App"() -> ("App.Kind"=w219:T4)  [unwired: 2 in, 2 out]
        n119 = control-ref of="Current VI Reference"() -> (w214:refnum<vi>)
        n120 = property class="VI"() -> ("FP.State"=w213:T3)  [unwired: 2 in, 2 out]
        n121 = Equal?(x=w213, y=T3."Closed" ("Front Panel Window:State")) -> (x = y?=w211:bool)
        n122 = Equal?(x=w219, y=T4."Run Time System" ("Application:Kind")) -> (x = y?=w217:bool)
        n123 = Or(x=w211, y=w217) -> (x .or. y?=w215:bool)
        n124 = Bundle By Name(cluster=w216, "Core.Current VI Reference"=w214, "Core.Close Panel on Exit?"=w215) -> (w221:T5)
        n125 = call <vilib>:"Add State(s) to Queue__JKI_lib_State_Machine.vi"("State(s) in (\"\")"=w223) -> ("States Out"=w222:string)  [unwired: 14 in]
      }
      frame "Error Handler" {
        # "Unhandled Error -- Display it"
        # "Handle any errors here.\nYou can also output any states to clean-up after errors occur"
        # "Clear error"
        n126 = call <vilib>:"General Error Handler.vi"("error in (no error)"=w225) -> ()  [unwired: 10 in, 5 out]
        n127 = call <vilib>:"Add State(s) to Queue__JKI_lib_State_Machine.vi"("State(s) in Front (\"\")"="/* Post Error States", "State(s) in (\"\")"=w229) -> ("States Out"=w228:string)  [unwired: 13 in]
      }
      frame "Exit" {
        # "Do not put any code in this frame.\n(No errors that occur here will be handled.)"
        n128 = call <vilib>:"Add State(s) to Queue__JKI_lib_State_Machine.vi"("State(s) in (\"\")"=w234) -> ("States Out"=w233:string)  [unwired: 14 in]
      }
      frame "---------- Data ----------" {
        # "Do not put any code in this frame.\n(It is a separator no-op. You can make a copy of this frame to create a new Data frame)"
        n129 = call <vilib>:"Add State(s) to Queue__JKI_lib_State_Machine.vi"("State(s) in (\"\")"=w238) -> ("States Out"=w237:string)  [unwired: 14 in]
      }
      frame "Data: Initialize" {
        w242 = dbl[] [] ("Offsets")
        w244 = dbl[][] []  # Temps_Array
        w245 = dbl[] []  # Temps
        w248 = T1[] []  # img_array
        w250 = u32 1 items=["Zoom Tool"=8, "Selection Tool"=0, "Pan Tool"=9, "Point Tool"=1, "Line Tool"=2, "Rectangle Tool"=3, "Rotated Rectangle Tool"=12, "Polyline Tool"=10, "Polygon Tool"=5, "Freehand Tool"=11, "Closed Freehand Tool"=6, "Ellipse Tool"=4, "Annulus Tool"=7] ("Current ROI Tool")
        w247 = 0  # State
        w251 = T11 {"Current VI Reference"=refnum, "Close Panel on Exit?"=FALSE}  # Core
        # "Initialize the shift-register data, here.\n(data names are defined by what you wire into the bundle function)"
        n130 = property on="Image" class="ImageControl"("Current ROI Tool"=w250) -> ()  [unwired: 2 in, 2 out]
        n131 = local write "Offsets"(w242) -> ()
        n132 = local write "FreezeFract Concatinated"(w242) -> ()
        n133 = local write "ThermTemps"(w242) -> ()
        n134 = local write "Slide"(w247) -> ()
        n135 = call "TCE_Config_Load.vi"() -> ("error out"=w239:errorcluster, "Config"=w241:T6)  [unwired: 10 in]
        n136 = call "TCE_Config_Save.vi"("error in"=w239, "Config"=w241) -> ("Config dup"=w240:T6)  [unwired: 8 in, 1 out]
        n137 = Bundle By Name(cluster=T5 {"Core"={"Current VI Reference"=refnum, "Close Panel on Exit?"=FALSE}, "Image Out"=refnum, "State"=0, "Points"={"Top Left"={"X"=0.0, "Y"=0.0}, "Top Right"={"X"=0.0, "Y"=0.0}, "Bottom Left"={"X"=0.0, "Y"=0.0}, "Bottom Right"={"X"=0.0, "Y"=0.0}, "x space 2"=0.0, "y space 2"=0.0, "x_space"=0.0, "y_space"=0.0, "Pixels"=[], "Fixpoint"={"X"=0.0, "Y"=0.0}}, "img_array"=[], "Temps"=[], "Temps_Array"=[], "Scan Area"=0.0, "Fixpoint Area"=0.0, "Config"={"Freezing"={"Cutoff"=2.0}}, "PCR Size"=0} ("Cluster"), "Core"=w251, "Image Out"=T1 refnum, "State"=w247, "img_array"=w248, "Temps"=w245, "Temps_Array"=w244, "Config"=w240) -> (w252:T5)
        n138 = call <vilib>:"Add State(s) to Queue__JKI_lib_State_Machine.vi"("State(s) in (\"\")"=w254) -> ("States Out"=w253:string)  [unwired: 14 in]
      }
      frame "Data: Cleanup" {
        # "Cleanup any data and references, here.\n(this is called automatically, by the Macro: Exit)"
        n139 = Unbundle By Name(w261) -> ("Config"=w255:T6, "img_array"=w259:T1[], "Image Out"=w258:T1)
        n140 = call "TCE_Config_Save.vi"("Config"=w255) -> ()  [unwired: 9 in, 2 out]
        n141 = call "IMAQ Dispose"("Image"=w258, "error in (no error)"=w257) -> ("error out"=w256:errorcluster)  [unwired: 4 in]
        n142 = for {
          shift-right: [w265] -> w260
          shift-left: w256 -> [w266]
          tunnel: w259 -> [w264] mode=indexing
          n143 = call "IMAQ Dispose"("Image"=w264, "error in (no error)"=w266) -> ("error out"=w265:errorcluster)  [unwired: 4 in]
        }
        n144 = call <vilib>:"Add State(s) to Queue__JKI_lib_State_Machine.vi"("State(s) in (\"\")"=w263) -> ("States Out"=w262:string)  [unwired: 14 in]
      }
      frame "Data: Config" {
        # "Do not put any code in this frame.\n(It is a separator no-op. You can make a copy of this frame to create a new Data frame)"
        n145 = call "TCE_Config.vi"("Cluster"=w268) -> ("Config out"=w267:T5)  [unwired: 9 in, 1 out]
        n146 = call <vilib>:"Add State(s) to Queue__JKI_lib_State_Machine.vi"("State(s) in (\"\")"=w271) -> ("States Out"=w270:string)  [unwired: 14 in]
      }
      frame "Data: Load Image" {
        # "Do not put any code in this frame.\n(It is a separator no-op. You can make a copy of this frame to create a new Data frame)"
        n147 = local write "img"(0 ("img")) -> ()
        n148 = local write "Slide"(u8 0 ("Slide")) -> ()
        n149 = Empty String/Path?(string/path="Path") -> (empty?=w281:bool)
        n150 = case shown="False" w281 {
          tunnel: [w302 _] -> w284
          tunnel: w283 -> [w299 w332]
          tunnel: [w303 w332] -> w277
          tunnel: "Path" -> [w291 _]
          tunnel: [w301 _] -> w279
          tunnel: w274 -> [w293 _]
          frame False {
            n151 = Build Path(base path=w291, name or relative path=path "Images") -> (appended path=w294:path)
            n152 = List Folder(path=w294) -> (filenames=w289:string[])  [unwired: 3 in, 3 out]
            n153 = property on="Slide" class="Slide (strict)"(error in=w299, "Visible"=TRUE) -> (error out=w298:errorcluster)  [unwired: 1 in, 1 out]
            n154 = call "Partition_Extract.vi"("input cluster"=w293, "Path"=w291) -> ("PartitionArray"=→"PartitionArray":string[])
            n155 = call "Thermistor_Extract.vi"("Path"=w291, "filenames"=w289) -> ("ThermTemps"=→"ThermTemps":dbl[])
            n156 = Array Size(array=w289) -> (size(s)=w297:i32)
            n157 = Format Into String(w297) -> (resulting string=w296:string)  [unwired: 3 in, 1 out]
            n158 = for {
              tunnel: [w331] -> w305
              tunnel: [w315] -> w301 mode=indexing
              tunnel: [w318] -> _ mode=indexing
              tunnel: w289 -> [w323] mode=indexing
              tunnel: w294 -> [w322]
              tunnel: w297 -> [w317]
              tunnel: w298 -> [w318]
              workers-P: _ -> [_]
              tunnel: w296 -> [w307]
              i -> [w316]
              w326 = T12 7 items=["Grayscale (U8)", "Grayscale (I16)", "Grayscale (SGL)", "Complex (CSG)", "RGB (U32)", "HSL (U32)", "RGB (U64)", "Grayscale (U16)"] ("Image Type")
              n159 = Format Into String(w316) -> (resulting string=w324:string)  [unwired: 3 in, 1 out]
              n160 = local read "img"() -> (w314:i32)
              n161 = Concatenate Strings("img_" ("Image Name"), w324) -> (w325:string)
              n162 = Build Path(base path=w322, name or relative path=w323) -> (appended path=w321:path)
              n163 = Increment(x=w314) -> (x+1=w308:i32)
              n164 = call "IMAQ Create"("Image Name"=w325, "Image Type"=w326, "error in (no error)"=w318) -> ("New Image"=w329:T1, "error out"=w330:errorcluster)  [unwired: 2 in]
              n165 = Format Into String(w308) -> (resulting string=w311:string)  [unwired: 3 in, 1 out]
              n166 = local write "img"(w308) -> ()
              n167 = call "IMAQ ReadFile 2"("File Path"=w321, "error in (no error)"=w330, "Image"=w329) -> ("error out"=w328:errorcluster, "Image Out"=w306:T1)  [unwired: 4 in, 3 out]
              n168 = Divide(x=w308, y=w317) -> (x/y=w320:dbl)
              n169 = Concatenate Strings("Loading image " ("Tutorial"), w311, " of " ("Tutorial"), w307) -> (w312:string)
              n170 = Multiply(x=w320, y=100.0) -> (x*y=→"Slide":dbl)
              n171 = local write "Tutorial"(w312) -> ()
              n172 = call "IMAQ Clear Overlay"("error in (no error)"=w328, "Image"=w306) -> ("error out"=w331:errorcluster, "Image Out"=w315:T1)  [unwired: 8 in]
              n173 = local write "Image"(w315) -> ()
            }
            n174 = Decrement(x=w297) -> (x-1=→"maxSize":i32)
            n175 = Index Array(array=w301) -> (element=w302:T1)  [unwired: 1 in]
            "Image" <- w302
            n176 = property on="Image" class="ImageControl"(error in=w305, "ROI"=T7 {"Global Rectangle"=[], "Contours"=[]}) -> (error out=w303:errorcluster)  [unwired: 1 in, 1 out]
          }
          frame True {
            (unwired) FALSE ("Visible")
          }
        }
        n177 = property on="Slide" class="Slide (strict)"(error in=w277, "Visible"=FALSE) -> (error out=w276:errorcluster)  [unwired: 1 in, 1 out]
        n178 = Bundle By Name(cluster=w274, "Image Out"=w284, "img_array"=w279) -> (w285:T5)
        n179 = local write "ImageIdx"(u32 0 ("Image")) -> ()
        n180 = call <vilib>:"Add State(s) to Queue__JKI_lib_State_Machine.vi"("State(s) in Front (\"\")"="Image: Set Cursors\nImage: Draw" ("State(s) in Front (\"\")"), "State(s) in (\"\")"=w287) -> ("States Out"=w286:string)  [unwired: 13 in]
      }
      frame "Data: Load Results" {
        # "Do not put any code in this frame.\n(It is a separator no-op. You can make a copy of this frame to create a new Data frame)"
        n181 = local read "Path"() -> (w335:path)
        n182 = Build Path(base path=w335, name or relative path=path "Data.TCE") -> (appended path=w336:path)
        n183 = call <vilib>:"Check if File or Folder Exists.vi"("path"=w336) -> ("file or folder exists?"=w338:bool, "dup path"=w337:path)  [unwired: 8 in, 1 out]
        n184 = case shown="True" w338 {
          tunnel: w337 -> [_ w352]
          tunnel: ["" ("State(s) in Front (\"\")") "UI: Single Temps >> Hide" ("State(s) in Front (\"\")")] -> w333
          frame False {
          }
          frame True {
            n185 = call-poly <vilib>:"Read Delimited Spreadsheet.vi"("file path (dialog if empty)"=w352, "delimiter (\\t)"=";" ("delimiter (\\t)")) -> ("all rows"=w351:string[][])  [unwired: 8 in, 5 out]
            n186 = call <vilib>:"Application Directory.vi"() -> ("Application Directory"=w354:path)
            n187 = Path To String(path=w352) -> (string=w359:string)
            n188 = call "DataArray_Reformatter.vi"("Data Array"=w351) -> ("MeltTemps"=w344:dbl[], "Offsets"=w347:dbl[], "FreezeTemps"=w350:dbl[], "Temps"=w349:dbl[][], "Offset Applied"=w346:bool)
            n189 = Build Path(base path=w354, name or relative path=path "TCEM.ini" ("file path (dialog if empty)")) -> (appended path=w355:path)
            n190 = Build Array(w359) -> (w358:string[])
            n191 = Not(x=w346) -> (.not. x?=w345:bool)
            n192 = local write "Offsets"(w347) -> ()
            n193 = local write "Offset Applied?"(w346) -> ()
            n194 = local write "MeltTemps"(w344) -> ()
            n195 = property on="Remove_Correction" class="Bool"("Visible"=w346) -> ()  [unwired: 2 in, 2 out]
            n196 = local write "Temps"(w349) -> ()
            n197 = local write "FreezeTemps"(w350) -> ()
            n198 = call-poly <vilib>:"Write Delimited Spreadsheet.vi"("file path (dialog if empty)"=w355, "1D data"=w358, "append to file? (new file:F)"=TRUE) -> ()  [unwired: 11 in, 2 out]
            n199 = property on="Correct Data" class="Bool"("Visible"=w345) -> ()  [unwired: 2 in, 2 out]
          }
        }
        n200 = call <vilib>:"Add State(s) to Queue__JKI_lib_State_Machine.vi"("State(s) in Front (\"\")"=w333, "State(s) in (\"\")"=w342) -> ("States Out"=w341:string)  [unwired: 13 in]
      }
      frame "Data: Load Calibration" {
        # "Do not put any code in this frame.\n(It is a separator no-op. You can make a copy of this frame to create a new Data frame)"
        n201 = local read "Path"() -> (w361:path)
        n202 = Build Path(base path=w361, name or relative path=path "TCC.cal") -> (appended path=w366:path)
        n203 = call <vilib>:"Check if File or Folder Exists.vi"("path"=w366) -> ("file or folder exists?"=w367:bool, "dup path"=w364:path)  [unwired: 8 in, 1 out]
        n204 = case shown="True" w367 {
          tunnel: w364 -> [_ w392]
          tunnel: w363 -> [w372 w391]
          tunnel: [w373 w390] -> w362
          tunnel: w361 -> [w376 _]
          tunnel: [w371 "Image: Draw\nData: Load Results\nData: Set Image\nProcess: Recalculate\nUI: Calc >> True\nUI: Menu Overlay Grid >> True\nUI: Menu Overlay Temps >> True\nUI: Progress >> Hide\nUI: Cursor Set >> Idle\nUI: Tutorial >> Click on a Well to show single or click outside the plate to show all."] -> w360
          frame False {
            n205 = call "CalibrationLoadPrompt.vi"("Root Path"=w376) -> ("cancel?"=w374:bool, "selected path"=w375:path)  [unwired: 9 in]
            n206 = case shown="False" w374 {
              tunnel: w375 -> [w380 _]
              tunnel: [w378 w385] -> w373
              tunnel: w372 -> [w379 w385]
              tunnel: ["Image: Draw\nData: Load Results\nData: Set Image\nProcess: Recalculate\nUI: Menu Overlay Grid >> True\nUI: Menu Overlay Temps >> True\nUI: Calc >> True\nUI: Progress >> Hide\nUI: Cursor Set >> Idle\nUI: Tutorial >> Click on a Well to show single or click outside the plate to show all." "UI: Calc >> Disable\nUI: Progress >> Hide\nUI: Cursor Set >> Idle\nUI: Tutorial >> Error: Missing Calibration File!"] -> w371
              frame False {
                n207 = call "TCam_Calibration_LoadSettings.vi"("path"=w380) -> ("Fixpoint Area"=w381:dbl, "Scan Area"=w382:dbl, "Points"=w383:T13)  [unwired: 7 in, 1 out]
                n208 = Bundle By Name(cluster=w379, "Points"=w383, "Scan Area"=w382, "Fixpoint Area"=w381) -> (w378:T5)
              }
              frame True {
              }
            }
          }
          frame True {
            n209 = call "TCam_Calibration_LoadSettings.vi"("path"=w392) -> ("Fixpoint Area"=w388:dbl, "Scan Area"=w389:dbl, "Points"=w386:T13)  [unwired: 7 in, 1 out]
            n210 = Bundle By Name(cluster=w391, "Points"=w386, "Scan Area"=w389, "Fixpoint Area"=w388) -> (w390:T5)
          }
        }
        n211 = call <vilib>:"Add State(s) to Queue__JKI_lib_State_Machine.vi"("State(s) in Front (\"\")"=w360, "State(s) in (\"\")"=w370) -> ("States Out"=w369:string)  [unwired: 13 in]
      }
      frame "Data: Set Image" {
        # "Do not put any code in this frame.\n(It is a separator no-op. You can make a copy of this frame to create a new Data frame)"
        n212 = Unbundle By Name(w397) -> ("img_array"=w396:T1[])
        n213 = Index Array(array=w396, index="ImageIdx") -> (element=w393:T1)
        n214 = Bundle By Name(cluster=w397, "Image Out"=w393) -> (w398:T5)
        n215 = call <vilib>:"Add State(s) to Queue__JKI_lib_State_Machine.vi"("State(s) in (\"\")"=w400) -> ("States Out"=w399:string)  [unwired: 14 in]
      }
      frame "Data: Show Img" {
        # "Do not put any code in this frame.\n(It is a separator no-op. You can make a copy of this frame to create a new Data frame)"
        n216 = Unbundle By Name(w401) -> ("Image Out"=w402:T1)
        n217 = local write "Image"(w402) -> ()
        n218 = call <vilib>:"Add State(s) to Queue__JKI_lib_State_Machine.vi"("State(s) in (\"\")"=w405) -> ("States Out"=w404:string)  [unwired: 14 in]
      }
      frame "Data: Update Well Temp" {
        # "Initialize the shift-register data, here.\n(data names are defined by what you wire into the bundle function)"
        n219 = local read "Temps single"() -> (w407:dbl[])
        n220 = local read "ImageIdx"() -> (w408:u32)
        n221 = Index Array(array=w407, index=w408) -> (element=w406:dbl)
        n222 = local write "CurTemp"(w406) -> ()
        n223 = call <vilib>:"Add State(s) to Queue__JKI_lib_State_Machine.vi"("State(s) in (\"\")"=w412) -> ("States Out"=w411:string)  [unwired: 14 in]
      }
      frame "Data: Temps Clear" {
        w413 = dbl[][] [] ("Temps_Array")
        w414 = dbl[] []  # Temps
        # "Initialize the shift-register data, here.\n(data names are defined by what you wire into the bundle function)"
        n224 = local write "Temps single"(w414) -> ()
        n225 = local write "Temps grads"(w413) -> ()
        n226 = local write "Temps"(w413) -> ()
        n227 = local write "Temps single grad"(w414) -> ()
        n228 = Bundle By Name(cluster=w416, "Temps"=w414, "Temps_Array"=w413) -> (w415:T5)
        n229 = call <vilib>:"Add State(s) to Queue__JKI_lib_State_Machine.vi"("State(s) in (\"\")"=w419) -> ("States Out"=w418:string)  [unwired: 14 in]
      }
      frame "Data: Save Results" {
        # "Initialize the shift-register data, here.\n(data names are defined by what you wire into the bundle function)"
        n230 = local read "FreezeFract Concatinated"() -> (w430:dbl[])
        n231 = local read "Offset Applied?"() -> (w426:bool)
        n232 = local read "PartitionArray"() -> (w428:string[])
        n233 = local read "FreezeTemps"() -> (w431:dbl[])
        n234 = local read "MeltTemps"() -> (w429:dbl[])
        n235 = local read "Offsets"() -> (w427:dbl[])
        n236 = local read "Temps"() -> (w432:dbl[][])
        n237 = call "TCE_SaveConfiguration.vi"("input cluster"=w433, "Temps"=w432, "FreezeTemps"=w431, "MeltTemps"=w429, "FrozenFraction"=w430, "PartitionArray"=w428, "Offsets"=w427, "Offset Applied?"=w426) -> ("Save Array out"=w424:string[][], "Full Array"=w423:string[][], "Canceled"=w422:bool)  [unwired: 9 in]
        n238 = case shown="False" w422 {
          tunnel: w420 -> [w450 w470]
          tunnel: w424 -> [w443 _]
          tunnel: [w442 "" ("State(s) in Front (\"\")")] -> w425
          tunnel: w423 -> [w438 _]
          tunnel: [w437 w470] -> w421
          frame False {
            n239 = local read "Path"() -> (w440:path)
            n240 = Build Path(base path=w440, name or relative path=path "Result Data.csv") -> (appended path=w445:path)
            n241 = Build Path(base path=w440, name or relative path=path "Data.TCE") -> (appended path=w439:path)
            n242 = call <vilib>:"Check if File or Folder Exists.vi"("path"=w445) -> ("file or folder exists?"=w448:bool, "dup path"=w444:path)  [unwired: 8 in, 1 out]
            n243 = case shown="False" w448 {
              selector: w448 -> [_ w456]
              tunnel: w440 -> [w454 _]
              tunnel: [w453 w455] -> w447
              tunnel: [w451 w456] -> w446
              tunnel: w444 -> [_ w455]
              frame False {
                n244 = call "ResultSavePrompt.vi"("Path"=w454) -> ("selected path"=w453:path, "cancel?"=w452:bool)
                n245 = Not(x=w452) -> (.not. x?=w451:bool)
              }
              frame True {
              }
            }
            n246 = case shown="True" w446 {
              tunnel: w443 -> [_ w468]
              tunnel: w450 -> [w457 w467]
              tunnel: w447 -> [_ w466]
              tunnel: ["" ("State(s) in Front (\"\")") "UI: Recent Menu Update" ("State(s) in Front (\"\")")] -> w442
              tunnel: w439 -> [_ w464]
              tunnel: w438 -> [_ w463]
              tunnel: [w457 w460] -> w437
              frame False {
              }
              frame True {
                w462 = ";" ("delimiter (\\t)")
                n247 = call-poly <vilib>:"Write Delimited Spreadsheet.vi"("file path (dialog if empty)"=w466, "2D data"=w468, "error in (no error)"=w467, "delimiter (\\t)"=w462) -> ("error out"=w461:errorcluster)  [unwired: 10 in, 1 out]
                n248 = call-poly <vilib>:"Write Delimited Spreadsheet.vi"("file path (dialog if empty)"=w464, "2D data"=w463, "error in (no error)"=w461, "delimiter (\\t)"=w462) -> ("new file path (Not A Path if cancelled)"=w459:path, "error out"=w460:errorcluster)  [unwired: 10 in]
                n249 = call "RunTimeMenu_TCE_RecentInsert.vi"("NewPath"=w459) -> ()  [unwired: 11 in]
              }
            }
          }
          frame True {
          }
        }
        n250 = case shown="Error .." w421 {
          frame No Error {
          }
          frame Error {
            n251 = One Button Dialog(message="File Save Error!\nClose file if open.") -> ()  [unwired: 1 in, 1 out]
          }
        }
        n252 = call <vilib>:"Add State(s) to Queue__JKI_lib_State_Machine.vi"("State(s) in Front (\"\")"=w425, "State(s) in (\"\")"=w435) -> ("States Out"=w434:string)  [unwired: 13 in]
      }
      frame "Data: Save Results As" {
        # "Initialize the shift-register data, here.\n(data names are defined by what you wire into the bundle function)"
        n253 = local read "FreezeFract Concatinated"() -> (w482:dbl[])
        n254 = local read "Offset Applied?"() -> (w478:bool)
        n255 = local read "PartitionArray"() -> (w480:string[])
        n256 = local read "FreezeTemps"() -> (w483:dbl[])
        n257 = local read "MeltTemps"() -> (w481:dbl[])
        n258 = local read "Offsets"() -> (w479:dbl[])
        n259 = local read "Temps"() -> (w484:dbl[][])
        n260 = call "TCE_SaveConfiguration.vi"("input cluster"=w477, "Temps"=w484, "FreezeTemps"=w483, "MeltTemps"=w481, "FrozenFraction"=w482, "PartitionArray"=w480, "Offsets"=w479, "Offset Applied?"=w478) -> ("Save Array out"=w476:string[][], "Full Array"=w473:string[][], "Canceled"=w474:bool)  [unwired: 9 in]
        n261 = case shown="False" w474 {
          tunnel: w471 -> [w495 w510]
          tunnel: w476 -> [w492 _]
          tunnel: [w491 "" ("State(s) in Front (\"\")")] -> w475
          tunnel: [w489 w510] -> w472
          tunnel: w473 -> [w488 _]
          frame False {
            n262 = local read "Path"() -> (w490:path)
            n263 = call "ResultSavePrompt.vi"("Path"=w490) -> ("selected path"=w494:path, "cancel?"=w493:bool)
            n264 = case shown="False" w493 {
              tunnel: w492 -> [w507 _]
              tunnel: w495 -> [w506 w508]
              tunnel: w494 -> [w505 _]
              tunnel: ["UI: Recent Menu Update" ("State(s) in Front (\"\")") "" ("State(s) in Front (\"\")")] -> w491
              tunnel: w490 -> [w503 _]
              tunnel: [w499 w508] -> w489
              tunnel: w488 -> [w498 _]
              frame False {
                w497 = ";" ("delimiter (\\t)")
                n265 = call-poly <vilib>:"Write Delimited Spreadsheet.vi"("file path (dialog if empty)"=w505, "2D data"=w507, "error in (no error)"=w506, "delimiter (\\t)"=w497) -> ("error out"=w500:errorcluster)  [unwired: 10 in, 1 out]
                n266 = Build Path(base path=w503, name or relative path=path "Data.TCE") -> (appended path=w501:path)
                n267 = call-poly <vilib>:"Write Delimited Spreadsheet.vi"("file path (dialog if empty)"=w501, "2D data"=w498, "error in (no error)"=w500, "delimiter (\\t)"=w497) -> ("new file path (Not A Path if cancelled)"=w496:path, "error out"=w499:errorcluster)  [unwired: 10 in]
                n268 = call "RunTimeMenu_TCE_RecentInsert.vi"("NewPath"=w496) -> ()  [unwired: 11 in]
              }
              frame True {
              }
            }
          }
          frame True {
          }
        }
        n269 = case shown="Error .." w472 {
          frame No Error {
          }
          frame Error {
            n270 = One Button Dialog(message="File Save Error!\nClose file if open.") -> ()  [unwired: 1 in, 1 out]
          }
        }
        n271 = call <vilib>:"Add State(s) to Queue__JKI_lib_State_Machine.vi"("State(s) in Front (\"\")"=w475, "State(s) in (\"\")"=w486) -> ("States Out"=w485:string)  [unwired: 13 in]
      }
      frame "---------- UI ----------" {
        # "Do not put any code in this frame.\n(It is a separator no-op. You can make a copy of this frame to create a new UI frame)"
        n272 = call <vilib>:"Add State(s) to Queue__JKI_lib_State_Machine.vi"("State(s) in (\"\")"=w515) -> ("States Out"=w514:string)  [unwired: 14 in]
      }
      frame "UI: Initialize" {
        w524 = FALSE ("Visible")
        w535 = T12 4 items=["Grayscale (U8)", "Grayscale (I16)", "Grayscale (SGL)", "Complex (CSG)", "RGB (U32)", "HSL (U32)", "RGB (U64)", "Grayscale (U16)"] ("Image Type")
        w516 = FALSE ("Visible")
        w523 = TRUE ("Zoom to Fit Mode")
        w520 = 0.0 ("X Scale.Range:Minimum")
        w522 = dbl[] []
        w519 = 0.0 ("Cursor.Cursor Position:Cursor X")
        w521 = dbl[][] []
        # "Initialize the User Interface, here.\n(this is called automatically, by the Macro: Init)"
        n273 = property on="Temps grads" class="WFGraph (strict)"("Visible"=w524) -> ()  [unwired: 2 in, 2 out]
        n274 = property on="Temps single grad" class="WFGraph (strict)"("Visible"=w524) -> ()  [unwired: 2 in, 2 out]
        n275 = control-ref of="Splitter 4"() -> (w526:refnum<vi>)
        n276 = local write "Offset Applied?"(FALSE ("Offset Applied?")) -> ()
        n277 = property on="FrozenFractionGraph" class="WFGraph (strict)"("Active Plot"=u32 0, "Legend Visible"=FALSE ("Legend:Visible")) -> ()  [unwired: 2 in, 2 out]
        n278 = property on="Image" class="ImageControl"("Zoom to Fit Mode"=w523) -> ()  [unwired: 2 in, 2 out]
        n279 = property on="FrozenFractionGraph" class="WFGraph (strict)"("Visible"=w523) -> ()  [unwired: 2 in, 2 out]
        n280 = property on="Temps" class="WFGraph (strict)"("XScale.Minimum"=w520) -> ()  [unwired: 2 in, 2 out]
        n281 = property on="FrozenFractionGraph" class="WFGraph (strict)"("XScale.Minimum"=w520) -> ()  [unwired: 2 in, 2 out]
        n282 = call "ShowHideSplit.vi"("Splitter in"=w526, "Show Split"=w516) -> ()  [unwired: 1 in]
        n283 = property on="Contents" class="Str"("Visible"=w516) -> ()  [unwired: 2 in, 2 out]
        n284 = property on="Calc_All" class="Bool"("Visible"=w516) -> ()  [unwired: 2 in, 2 out]
        n285 = property on="CurTemp" class="DigNum (strict)"("Visible"=FALSE) -> ()  [unwired: 2 in, 2 out]
        n286 = property on="Fraction Single" class="WFGraph (strict)"("Visible"=w516) -> ()  [unwired: 2 in, 2 out]
        n287 = call <vilib>:"Application Directory.vi"() -> ("Application Directory"=w539:path)
        n288 = property on="Well" class="Str"("Visible"=w516) -> ()  [unwired: 2 in, 2 out]
        n289 = call "Read Exe Version.vi"("Application name"=path "TCE.exe") -> ("FileVersion"=w531:string)  [unwired: 7 in, 3 out]
        n290 = Path To String(path=w539) -> (string=w541:string)
        n291 = Concatenate Strings("version " ("string"), w531) -> (→"version":string)
        n292 = property on="Remove_Correction" class="Bool"("Visible"=w516) -> ()  [unwired: 2 in, 2 out]
        n293 = property on="Correct Data" class="Bool"("Visible"=w516) -> ()  [unwired: 2 in, 2 out]
        n294 = call "IMAQ Create"("Image Name"="placeholder_img_TCE", "Image Type"=w535) -> ("New Image"=w538:T1)  [unwired: 3 in, 1 out]
        n295 = Concatenate Strings(w541, "\\camera_placeholder.png") -> (w540:string)
        n296 = String To Path(string=w540) -> (path=w542:path)
        n297 = call "IMAQ ReadFile 2"("Use File Path Image Type"=FALSE, "File Path"=w542, "Image"=w538) -> ("Image Out"=w533:T1)  [unwired: 4 in, 4 out]
        "placeholder image" <- w533
        n298 = local write "Image"(w533) -> ()
        n299 = local write "Path"(path "" ("Path")) -> ()
        n300 = local write "Temps single"(w522) -> ()
        n301 = local write "Temps single grad"(w522) -> ()
        n302 = local write "FrozenFractionGraph"(w521) -> ()
        n303 = local write "Temps"(w521) -> ()
        n304 = property on="Temps single" class="WFGraph (strict)"("Cursor.Cursor X"=w519) -> ()  [unwired: 2 in, 2 out]
        n305 = property on="Temps" class="WFGraph (strict)"("Cursor.Cursor X"=w519) -> ()  [unwired: 2 in, 2 out]
        n306 = local write "Temps grads"(w521) -> ()
        n307 = property on="Temps grads" class="WFGraph (strict)"("Cursor.Cursor X"=w519) -> ()  [unwired: 2 in, 2 out]
        n308 = property on="Temps single grad" class="WFGraph (strict)"("Cursor.Cursor X"=w519) -> ()  [unwired: 2 in, 2 out]
        n309 = property on="FrozenFractionGraph" class="WFGraph (strict)"("Cursor.Cursor X"=w519) -> ()  [unwired: 2 in, 2 out]
        n310 = call <vilib>:"Add State(s) to Queue__JKI_lib_State_Machine.vi"("State(s) in Front (\"\")"="UI: Tutorial\nUI: Recent Menu Update\nUI: Progress >> Hide\nUI: Menu Save >> Hide\nUI: Menu Overlay Grid >> Hide\nUI: Menu Overlay Temps >> Hide" ("State(s) in Front (\"\")"), "State(s) in (\"\")"=w550) -> ("States Out"=w549:string)  [unwired: 13 in]
        "img" <- 0
        "Title" <- "Thermal Camera Evaluation" ("Title")
        "Title 2" <- "Well Data" ("Title 2")
      }
      frame "UI: Progress" {
        # "Initialize the User Interface, here.\n(this is called automatically, by the Macro: Init)"
        n311 = case shown="\"Show\"" w554 {
          tunnel: [FALSE ("Visible") TRUE ("Visible")] -> w553
          frame "Hide", Default {
          }
          frame "Show" {
          }
        }
        n312 = local write "img"(0 ("img")) -> ()
        n313 = local write "Slide"(u8 0 ("Slide")) -> ()
        n314 = property on="Slide" class="Slide (strict)"("Visible"=w553) -> ()  [unwired: 2 in, 2 out]
        n315 = call <vilib>:"Add State(s) to Queue__JKI_lib_State_Machine.vi"("State(s) in (\"\")"=w558) -> ("States Out"=w557:string)  [unwired: 14 in]
      }
      frame "UI: Recent Menu Update" {
        # "Initialize the User Interface, here.\n(this is called automatically, by the Macro: Init)"
        n316 = Current VI's Menubar() -> (w562:refnum<k9>)
        n317 = call "RunTimeMenu_Initialize_TCE.vi"("Menu in"=w562) -> ("paths"=→"recentPaths":path[])  [unwired: 9 in, 1 out]
        n318 = call <vilib>:"Add State(s) to Queue__JKI_lib_State_Machine.vi"("State(s) in (\"\")"=w566) -> ("States Out"=w565:string)  [unwired: 14 in]
      }
      frame "UI: Show First Image" {
        w567 = 0.0 ("Cursor.Cursor Position:Cursor X")
        # "Initialize the User Interface, here.\n(this is called automatically, by the Macro: Init)"
        n319 = Unbundle By Name(w570) -> ("img_array"=w569:T1[])
        n320 = property on="Temps" class="WFGraph (strict)"("Cursor.Cursor X"=w567) -> ()  [unwired: 2 in, 2 out]
        n321 = property on="Temps grads" class="WFGraph (strict)"("Cursor.Cursor X"=w567) -> ()  [unwired: 2 in, 2 out]
        n322 = property on="Temps single grad" class="WFGraph (strict)"("Cursor.Cursor X"=w567) -> ()  [unwired: 2 in, 2 out]
        n323 = property on="Temps single" class="WFGraph (strict)"("Cursor.Cursor X"=w567) -> ()  [unwired: 2 in, 2 out]
        n324 = property on="FrozenFractionGraph" class="WFGraph (strict)"("Cursor.Cursor X"=w567) -> ()  [unwired: 2 in, 2 out]
        n325 = property on="Fraction Single" class="WFGraph (strict)"("Cursor.Cursor X"=w567) -> ()  [unwired: 2 in, 2 out]
        n326 = Index Array(array=w569) -> (element=w568:T1)  [unwired: 1 in]
        n327 = local write "Image"(w568) -> ()
        n328 = call <vilib>:"Add State(s) to Queue__JKI_lib_State_Machine.vi"("State(s) in (\"\")"=w573) -> ("States Out"=w572:string)  [unwired: 14 in]
      }
      frame "UI: Tutorial" {
        # "Initialize the User Interface, here.\n(this is called automatically, by the Macro: Init)"
        n329 = call <vilib>:"Add State(s) to Queue__JKI_lib_State_Machine.vi"("State(s) in (\"\")"=w578) -> ("States Out"=w577:string)  [unwired: 14 in]
        "Tutorial" <- w574
      }
      frame "UI: Calc" {
        # "Initialize the User Interface, here.\n(this is called automatically, by the Macro: Init)"
        n330 = case shown="\"Hidden\", \"Hide\"" w581 {
          tunnel: [T8."Disabled and Grayed Out" ("Disabled") T8."Disabled and Grayed Out" ("Disabled") T8."Enabled" ("Disabled")] -> w580
          tunnel: [TRUE FALSE TRUE] -> w579
          frame "Disable", "False", Default {
          }
          frame "Hidden", "Hide" {
          }
          frame "True" {
          }
        }
        n331 = property on="Calc_All" class="Bool"("DisabledEnum"=w580) -> ()  [unwired: 2 in, 2 out]
        n332 = property on="Calc_All" class="Bool"("Visible"=w579) -> ()  [unwired: 2 in, 2 out]
        n333 = call <vilib>:"Add State(s) to Queue__JKI_lib_State_Machine.vi"("State(s) in (\"\")"=w585) -> ("States Out"=w584:string)  [unwired: 14 in]
      }
      frame "UI: Cursor Set" {
        # "Argument"
        # "Set and Unset Cursor Busy.\n(Usage: \"UI: Cursor Set >> Busy|Idle\")"
        n334 = case shown="\"Busy\"" w592 {
          tunnel: w594 -> [w599 w601]
          tunnel: [w598 w600] -> w593
          frame "Idle", Default {
            n335 = call <vilib>:"Unset Busy.vi"("error in (no error)"=w599) -> ("error out"=w598:errorcluster)  [unwired: 10 in]
          }
          frame "Busy" {
            n336 = call <vilib>:"Set Busy.vi"("error in (no error)"=w601) -> ("error out"=w600:errorcluster)  [unwired: 9 in, 1 out]
          }
        }
        n337 = call <vilib>:"Add State(s) to Queue__JKI_lib_State_Machine.vi"("State(s) in (\"\")"=w597) -> ("States Out"=w596:string)  [unwired: 14 in]
      }
      frame "UI: Menu Save" {
        # "Argument"
        # "Set and Unset Cursor Busy.\n(Usage: \"UI: Cursor Set >> Busy|Idle\")"
        n338 = case shown="\"Active\", \"Show\", \"True\"" w605 {
          tunnel: [FALSE TRUE] -> w603
          frame "Disable", "False", Default {
          }
          frame "Active", "Show", "True" {
          }
        }
        n339 = Current VI's Menubar() -> (w604:refnum<k9>)
        n340 = call "RunTimeMenu_Save_State_TCE.vi"("enabled"=w603, "item tag"=string[] ["DATA_SAVE", "DATA_SAVE_AS"], "Menu in"=w604) -> ()  [unwired: 8 in, 1 out]
        n341 = call <vilib>:"Add State(s) to Queue__JKI_lib_State_Machine.vi"("State(s) in (\"\")"=w609) -> ("States Out"=w608:string)  [unwired: 14 in]
      }
      frame "UI: Menu Overlay Grid" {
        # "Argument"
        # "Set and Unset Cursor Busy.\n(Usage: \"UI: Cursor Set >> Busy|Idle\")"
        n342 = case shown="\"Active\", \"Show\", \"True\"" w615 {
          tunnel: [FALSE TRUE] -> w613
          frame "Disable", "False", Default {
          }
          frame "Active", "Show", "True" {
          }
        }
        n343 = Current VI's Menubar() -> (w614:refnum<k9>)
        n344 = call "RunTimeMenu_Save_State_TCE.vi"("enabled"=w613, "item tag"=string[] ["OVERLAY_GRID", "OVERLAY_CLEAR"], "Menu in"=w614) -> ()  [unwired: 8 in, 1 out]
        n345 = call <vilib>:"Add State(s) to Queue__JKI_lib_State_Machine.vi"("State(s) in (\"\")"=w619) -> ("States Out"=w618:string)  [unwired: 14 in]
      }
      frame "UI: Menu Overlay Temps" {
        # "Argument"
        # "Set and Unset Cursor Busy.\n(Usage: \"UI: Cursor Set >> Busy|Idle\")"
        n346 = case shown="\"Active\", \"Show\", \"True\"" w625 {
          tunnel: [FALSE TRUE] -> w623
          frame "Disable", "False", Default {
          }
          frame "Active", "Show", "True" {
          }
        }
        n347 = Current VI's Menubar() -> (w624:refnum<k9>)
        n348 = call "RunTimeMenu_Save_State_TCE.vi"("enabled"=w623, "item tag"=string[] ["OVERLAY_TEMPS", "OVERLAY_FREEZE"], "Menu in"=w624) -> ()  [unwired: 8 in, 1 out]
        n349 = call <vilib>:"Add State(s) to Queue__JKI_lib_State_Machine.vi"("State(s) in (\"\")"=w629) -> ("States Out"=w628:string)  [unwired: 14 in]
      }
      frame "UI: Single Temps" {
        w634 = FALSE ("Visible")
        # "Argument"
        # "Set and Unset Cursor Busy.\n(Usage: \"UI: Cursor Set >> Busy|Idle\")"
        n350 = control-ref of="Splitter 4"() -> (w635:refnum<vi>)
        n351 = case shown="\"Active\", \"Show\", \"True\"" w636 {
          tunnel: [w641 w644] -> w632
          tunnel: w635 -> [w642 w643]
          frame "Disable", "False", Default {
            w641 = FALSE
            n352 = call "ShowHideSplit.vi"("Splitter in"=w642, "Show Split"=w641) -> ()  [unwired: 1 in]
          }
          frame "Active", "Show", "True" {
            w644 = TRUE
            n353 = call "ShowHideSplit.vi"("Splitter in"=w643, "Show Split"=w644) -> ()  [unwired: 1 in]
          }
        }
        n354 = property on="Temps single" class="WFGraph (strict)"("Visible"=w632) -> ()  [unwired: 2 in, 2 out]
        n355 = Not(x=w632) -> (.not. x?=w633:bool)
        n356 = property on="Fraction Single" class="WFGraph (strict)"("Visible"=w632) -> ()  [unwired: 2 in, 2 out]
        n357 = property on="Temps" class="WFGraph (strict)"("Visible"=w633) -> ()  [unwired: 2 in, 2 out]
        n358 = property on="Temps grads" class="WFGraph (strict)"("Visible"=w634) -> ()  [unwired: 2 in, 2 out]
        n359 = property on="Temps single grad" class="WFGraph (strict)"("Visible"=w634) -> ()  [unwired: 2 in, 2 out]
        n360 = property on="FrozenFractionGraph" class="WFGraph (strict)"("Visible"=w633) -> ()  [unwired: 2 in, 2 out]
        n361 = property on="CurTemp" class="DigNum (strict)"("Visible"=w632) -> ()  [unwired: 2 in, 2 out]
        n362 = property on="Contents" class="Str"("Visible"=w632) -> ()  [unwired: 2 in, 2 out]
        n363 = property on="Well" class="Str"("Visible"=w632) -> ()  [unwired: 2 in, 2 out]
        n364 = call <vilib>:"Add State(s) to Queue__JKI_lib_State_Machine.vi"("State(s) in (\"\")"=w640) -> ("States Out"=w639:string)  [unwired: 14 in]
      }
      frame "UI: Front Panel State" {
        # "Argument"
        # "Set Front Panel Open or Closed\n(Usage: \"UI: Front Panel State >> Open|Close\")"
        n365 = Unbundle By Name(w647) -> ("Core.Current VI Reference"=w646:refnum<vi>)
        n366 = case shown="\"Minimize\", \"Minimized\"" w645 {
          tunnel: w649 -> [w657 w672 w683 w696 w709]
          tunnel: [w659 w673 w685 w698 w711] -> w648
          tunnel: w646 -> [w658 w670 w684 w697 w710]
          frame "Open", "Standard", Default {
            w652 = T3."Standard" ("State")
            n367 = property class="VI"(reference=w658, error in=w657) -> (reference out=w655:refnum<vi>, error out=w656:errorcluster, "FP.State"=w654:T3)
            n368 = Not Equal?(x=w654, y=w652) -> (x != y?=w653:bool)
            n369 = case shown="True" w653 {
              tunnel: [w663 w665] -> w659
              tunnel: w656 -> [w662 w665]
              tunnel: w655 -> [w661 _]
              tunnel: w652 -> [w660 _]
              frame True {
                n370 = invoke class="VI" method="FP.Open"(reference=w661, error in=w662, "Activate"=TRUE, "State"=w660) -> (error out=w663:errorcluster)  [unwired: 1 in, 4 out]
              }
              frame False {
              }
            }
          }
          frame "Close", "Closed" {
            n371 = property class="VI"(reference=w670, error in=w672) -> (reference out=w669:refnum<vi>, error out=w671:errorcluster, "FP.State"=w667:T3)
            n372 = Not Equal?(x=w667, y=T3."Closed" ("Front Panel Window:State")) -> (x != y?=w666:bool)
            n373 = case shown="True" w666 {
              tunnel: [w674 w677] -> w673
              tunnel: w671 -> [w674 w676]
              tunnel: w669 -> [_ w675]
              frame False {
              }
              frame True {
                n374 = invoke class="VI" method="FP.Close"(reference=w675, error in=w676) -> (error out=w677:errorcluster)  [unwired: 1 in, 2 out]
              }
            }
          }
          frame "Hidden", "Hide" {
            w678 = T3."Hidden" ("State")
            n375 = property class="VI"(reference=w684, error in=w683) -> (reference out=w681:refnum<vi>, error out=w682:errorcluster, "FP.State"=w680:T3)
            n376 = Not Equal?(x=w680, y=w678) -> (x != y?=w679:bool)
            n377 = case shown="True" w679 {
              tunnel: [w689 w690] -> w685
              tunnel: w682 -> [w688 w690]
              tunnel: w681 -> [w687 _]
              tunnel: w678 -> [w686 _]
              frame True {
                n378 = invoke class="VI" method="FP.Open"(reference=w687, error in=w688, "State"=w686) -> (error out=w689:errorcluster)  [unwired: 2 in, 4 out]
              }
              frame False {
              }
            }
          }
          frame "Minimize", "Minimized" {
            w691 = T3."Minimized" ("State")
            n379 = property class="VI"(reference=w697, error in=w696) -> (reference out=w694:refnum<vi>, error out=w695:errorcluster, "FP.State"=w693:T3)
            n380 = Not Equal?(x=w693, y=w691) -> (x != y?=w692:bool)
            n381 = case shown="True" w692 {
              tunnel: [w702 w703] -> w698
              tunnel: w695 -> [w701 w703]
              tunnel: w694 -> [w700 _]
              tunnel: w691 -> [w699 _]
              frame True {
                n382 = invoke class="VI" method="FP.Open"(reference=w700, error in=w701, "State"=w699) -> (error out=w702:errorcluster)  [unwired: 2 in, 4 out]
              }
              frame False {
              }
            }
          }
          frame "Maximize", "Maximized" {
            w704 = T3."Maximized" ("State")
            n383 = property class="VI"(reference=w710, error in=w709) -> (reference out=w707:refnum<vi>, error out=w708:errorcluster, "FP.State"=w706:T3)
            n384 = Not Equal?(x=w706, y=w704) -> (x != y?=w705:bool)
            n385 = case shown="True" w705 {
              tunnel: [w715 w716] -> w711
              tunnel: w708 -> [w714 w716]
              tunnel: w707 -> [w713 _]
              tunnel: w704 -> [w712 _]
              frame True {
                n386 = invoke class="VI" method="FP.Open"(reference=w713, error in=w714, "State"=w712) -> (error out=w715:errorcluster)  [unwired: 2 in, 4 out]
              }
              frame False {
              }
            }
          }
        }
        n387 = call <vilib>:"Add State(s) to Queue__JKI_lib_State_Machine.vi"("State(s) in (\"\")"=w651) -> ("States Out"=w650:string)  [unwired: 14 in]
      }
      frame "---------- Macro ----------" {
        # "Do not put any code in this frame.\n(It is a separator no-op. You can make a copy of this frame to create a new Macro frame)"
        n388 = call <vilib>:"Add State(s) to Queue__JKI_lib_State_Machine.vi"("State(s) in (\"\")"=w720) -> ("States Out"=w719:string)  [unwired: 14 in]
      }
      frame "Macro: Initialize" {
        w721 = "// UI: Cursor Set >> Busy\nData: Initialize\nInitialize Core Data\nUI: Initialize\nUI: Front Panel State >> Show\nUI: Tutorial >> Load Image\n// Image: Draw\n// UI: Cursor Set >> Idle"  # // UI: Cursor Set >> Busy Data: Initialize Initialize Core Data UI: Initialize UI: Front Panel State >> Show UI: Tutorial >> Load Image // Image: Draw // UI: Cursor Set >> Idle
        # "Initialization Macro\n(This is called once, when the VI starts)"
        n389 = call <vilib>:"Add State(s) to Queue__JKI_lib_State_Machine.vi"("State(s) in Front (\"\")"=w721, "State(s) in (\"\")"=w725) -> ("States Out"=w724:string)  [unwired: 13 in]
      }
      frame "Macro: Exit" {
        # "Exit Macro\n(This is called once, when the VI exits)"
        n390 = Unbundle By Name(w732) -> ("Core.Close Panel on Exit?"=w731:bool)
        n391 = Select(t="UI: Front Panel State >> Close", s=w731, f="") -> (s? t:f=w728:string)
        n392 = call <vilib>:"Add State(s) to Queue__JKI_lib_State_Machine.vi"("State(s) in (\"\")"=w728, "State(s) at Back (\"\")"="Data: Cleanup\nExit") -> ("States Out"=w726:string)  [unwired: 13 in]
        n393 = call <vilib>:"Add State(s) to Queue__JKI_lib_State_Machine.vi"("State(s) in Front (\"\")"=w726, "State(s) in (\"\")"=w735) -> ("States Out"=w734:string)  [unwired: 13 in]
      }
      frame "---------- Process ----------" {
        # "Template Separator\n(You can make a copy of, or modify, this frame)"
        n394 = call <vilib>:"Add State(s) to Queue__JKI_lib_State_Machine.vi"("State(s) in (\"\")"=w739) -> ("States Out"=w738:string)  [unwired: 14 in]
      }
      frame "Process: Calculate All" {
        # "Template Separator\n(You can make a copy of, or modify, this frame)"
        n395 = call <vilib>:"Add State(s) to Queue__JKI_lib_State_Machine.vi"("State(s) in Front (\"\")"="Data: Temps Clear\nData: Set Image\nUI: Cursor Set >> Busy\nUI: Progress >> Show\nProcess: Calculate All Temps\nProcess: Calculate Gradients\nProcess: Calculate Freezing Points\nProcess: Calculate Offset\nProcess: Calculate Melt Temp\nProcess: Calculate Freeze Fraction\nUI: Progress >> Hide\nUI: Cursor Set >> Idle\nUI: Tutorial >> Click on a Well to show single or click outside the plate to show all." ("State(s) in Front (\"\")"), "State(s) in (\"\")"=w744) -> ("States Out"=w743:string)  [unwired: 13 in]
      }
      frame "Process: Recalculate" {
        # "Template Separator\n(You can make a copy of, or modify, this frame)"
        n396 = call <vilib>:"Add State(s) to Queue__JKI_lib_State_Machine.vi"("State(s) in Front (\"\")"="Process: Calculate Gradients\nProcess: Calculate Freezing Points\nProcess: Calculate Melt Temp\nProcess: Calculate Freeze Fraction" ("State(s) in Front (\"\")"), "State(s) in (\"\")"=w749) -> ("States Out"=w748:string)  [unwired: 13 in]
      }
      frame "Process: Calculate Temps" {
        # "Your code here.\n(You can make a copy of, or modify, this frame)"
        n397 = Unbundle By Name(w755) -> ("Image Out"=w753:T1, "Points.Pixels"=w752:cluster{"X":i32, "Y":i32}[][], "Points.Top Left.X"=w763:sgl, "Points.Top Right.X"=w762:sgl, "Points.Bottom Left.X"=w761:sgl, "Points.Bottom Right.X"=w760:sgl)
        n398 = Equal To 0?(x=w763) -> (x = 0?=w759:bool)
        n399 = Equal To 0?(x=w762) -> (x = 0?=w758:bool)
        n400 = Equal To 0?(x=w761) -> (x = 0?=w757:bool)
        n401 = Equal To 0?(x=w760) -> (x = 0?=w756:bool)
        n402 = local read "Points"() -> (w751:T2[])
        n403 = Compound Arithmetic op=OR(w759, w758, w757, w756) -> (w754:bool)
        n404 = case shown="False" w754 {
          tunnel: w753 -> [w769 w770]
          tunnel: w752 -> [w768 _]
          tunnel: w751 -> [_ _]
          tunnel: [w767 w770] -> w750
          frame False {
            n405 = call "TCam_WellTemp.vi"("Pixels"=w768, "Image in"=w769) -> ("Image Out"=w767:T1)  [unwired: 7 in, 2 out]
          }
          frame True {
          }
        }
        n406 = local write "Image"(w750) -> ()
        n407 = call <vilib>:"Add State(s) to Queue__JKI_lib_State_Machine.vi"("State(s) in (\"\")"=w766) -> ("States Out"=w765:string)  [unwired: 14 in]
      }
      frame "Process: Calculate Well" {
        # "Your code here.\n(You can make a copy of, or modify, this frame)"
        n408 = Unbundle By Name(w772) -> ("Image Out"=w777:T1, "Points.Pixels"=w776:cluster{"X":i32, "Y":i32}[][], "Points.Top Left.X"=w785:sgl, "Points.Top Right.X"=w784:sgl, "Points.Bottom Left.X"=w783:sgl, "Points.Bottom Right.X"=w782:sgl)
        n409 = local read "Points"() -> (w775:T2[])
        n410 = Equal To 0?(x=w785) -> (x = 0?=w781:bool)
        n411 = Equal To 0?(x=w784) -> (x = 0?=w780:bool)
        n412 = Equal To 0?(x=w783) -> (x = 0?=w779:bool)
        n413 = Equal To 0?(x=w782) -> (x = 0?=w778:bool)
        n414 = Compound Arithmetic op=OR(w781, w780, w779, w778) -> (w774:bool)
        n415 = case shown="False" w774 {
          tunnel: w777 -> [w810 _]
          tunnel: w776 -> [w809 _]
          tunnel: w775 -> [w808 _]
          tunnel: [w803 _] -> w773
          tunnel: w772 -> [w796 _]
          tunnel: w772 -> [w794 w815]
          tunnel: [w793 w815] -> w771
          frame False {
            n416 = local read "ImageIdx"() -> (w790:u32)
            n417 = property on="ImageIdx" class="Slide (strict)"() -> ("Scale.Maximum"=w798:dbl)  [unwired: 2 in, 2 out]
            n418 = call "TCam_WellCalculater.vi"("DrawTempOverlay"=TRUE, "Well Pos"=w808, "Pixels"=w809, "Image in"=w810, "index"="Well") -> ("Image Out"=w807:T1, "mean"=w792:dbl)  [unwired: 5 in]
            n419 = Increment(x=w790) -> (x+1=w804:u32)
            n420 = local write "Image"(w807) -> ()
            n421 = Greater?(x=w804, y=w798) -> (0:w806:bool)
            n422 = case shown="False" w806 {
              tunnel: w804 -> [_ w814]
              tunnel: [w813 w814] -> w805
              tunnel: w804 -> [w813 _]
              tunnel: ["Data: Set Image\nProcess: Calculate Well" ("State(s) in Front (\"\")") _] -> w803
              tunnel: [TRUE _] -> w802
              frame False {
              }
              frame True {
              }
            }
            n423 = Unbundle By Name(w796) -> ("Temps"=w795:dbl[])
            n424 = Divide(x=w790, y=w798) -> (x/y=w801:dbl)
            n425 = property on="Temps single" class="WFGraph (strict)"("Cursor.Cursor X"=w790) -> ()  [unwired: 2 in, 2 out]
            n426 = Multiply(x=w801, y=100.0) -> (x*y=w799:dbl)
            n427 = Build Array (concatenate)(w795, w792) -> (w791:dbl[])
            "Temps single" <- w791
            n428 = local write "Slide"(w799) -> ()
            n429 = Bundle By Name(cluster=w794, "Temps"=w791) -> (w793:T5)
            n430 = local write "ImageIdx"(w805) -> ()
            n431 = property on="Slide" class="Slide (strict)"("Visible"=w802) -> ()  [unwired: 2 in, 2 out]
          }
          frame True {
          }
        }
        n432 = call <vilib>:"Add State(s) to Queue__JKI_lib_State_Machine.vi"("State(s) in Front (\"\")"=w773, "State(s) in (\"\")"=w788) -> ("States Out"=w787:string)  [unwired: 13 in]
      }
      frame "Process: Calculate All Temps" {
        # "Your code here.\n(You can make a copy of, or modify, this frame)"
        n433 = Unbundle By Name(w818) -> ("img_array"=w821:T1[], "Points.Pixels"=w820:cluster{"X":i32, "Y":i32}[][], "Points.Top Left.X"=w829:sgl, "Points.Top Right.X"=w828:sgl, "Points.Bottom Left.X"=w827:sgl, "Points.Bottom Right.X"=w826:sgl)
        n434 = Equal To 0?(x=w829) -> (x = 0?=w825:bool)
        n435 = Equal To 0?(x=w828) -> (x = 0?=w824:bool)
        n436 = Equal To 0?(x=w827) -> (x = 0?=w823:bool)
        n437 = Equal To 0?(x=w826) -> (x = 0?=w822:bool)
        n438 = Compound Arithmetic op=OR(w825, w824, w823, w822) -> (w819:bool)
        n439 = case shown="False" w819 {
          tunnel: w821 -> [w835 _]
          tunnel: w820 -> [w837 _]
          tunnel: [TRUE ("Visible") FALSE ("Visible")] -> w816
          tunnel: [w833 dbl[][] []] -> w817
          frame False {
            n440 = for {
              N -> [w840]
              tunnel: w835 -> [w851] mode=indexing
              tunnel: w837 -> [w850]
              tunnel: [w849] -> w836 mode=indexing
              workers-P: _ -> [_]
              i -> [w838]
              n441 = call "TCam_WellTemp.vi"("Pixels"=w850, "Image in"=w851) -> ("Temps"=w849:dbl[])  [unwired: 7 in, 2 out]
              n442 = property on="ImageIdx" class="Slide (strict)"() -> ("Scale.Maximum"=w846:dbl)  [unwired: 2 in, 2 out]
              n443 = local read "img"() -> (w848:i32)
              n444 = property on="Temps" class="WFGraph (strict)"("Cursor.Cursor X"=w838) -> ()  [unwired: 2 in, 2 out]
              n445 = Increment(x=w848) -> (x+1=w839:i32)
              n446 = Divide(x=w839, y=w846) -> (x/y=w853:dbl)
              n447 = local write "img"(w839) -> ()
              n448 = Format Into String(w839) -> (resulting string=w845:string)  [unwired: 3 in, 1 out]
              n449 = Multiply(x=w853, y=100.0) -> (x*y=w847:dbl)
              n450 = property on="Temps grads" class="WFGraph (strict)"("Cursor.Cursor X"=w838) -> ()  [unwired: 2 in, 2 out]
              n451 = Format Into String(w840) -> (resulting string=w841:string)  [unwired: 3 in, 1 out]
              n452 = local write "Slide"(w847) -> ()
              n453 = Concatenate Strings("Processing image " ("Tutorial"), w845, " of " ("Tutorial"), w841) -> (w844:string)
              n454 = property on="FrozenFractionGraph" class="WFGraph (strict)"("Cursor.Cursor X"=w838) -> ()  [unwired: 2 in, 2 out]
              n455 = local write "Tutorial"(w844) -> ()
            }
            n456 = Transpose 2D Array(2D array=w836) -> (transposed array=w833:dbl[][])
          }
          frame True {
          }
        }
        "Temps" <- w817
        n457 = property on="Correct Data" class="Bool"("Visible"=w816) -> ()  [unwired: 2 in, 2 out]
        n458 = call <vilib>:"Add State(s) to Queue__JKI_lib_State_Machine.vi"("State(s) in (\"\")"=w832) -> ("States Out"=w831:string)  [unwired: 14 in]
      }
      frame "Process: Calculate Gradients" {
        # "Your code here.\n(You can make a copy of, or modify, this frame)"
        n459 = local read "Temps"() -> (w857:dbl[][])
        n460 = for {
          tunnel: w857 -> [w866] mode=indexing
          workers-P: _ -> [_]
          tunnel: [w862] -> w856 mode=indexing
          n461 = Array Size(array=w866) -> (size(s)=w865:i32)
          n462 = Decrement(x=w865) -> (x-1=w864:i32)
          n463 = for {
            N: w864 -> [_]
            tunnel: w866 -> [w874]
            shift-right: [w868] -> w862
            shift-left: dbl[] [0.0] -> [w867]
            i -> [w873]
            n464 = Increment(x=w873) -> (x+1=w872:i32)
            n465 = Index Array(array=w874, index=w873) -> (element=w870:dbl)
            n466 = Index Array(array=w874, index=w872) -> (element=w871:dbl)
            n467 = Subtract(x=w871, y=w870) -> (x-y=w869:dbl)
            n468 = Build Array (concatenate)(w867, w869) -> (w868:dbl[])
          }
        }
        "Temps grads" <- w856
        n469 = call <vilib>:"Add State(s) to Queue__JKI_lib_State_Machine.vi"("State(s) in (\"\")"=w861) -> ("States Out"=w860:string)  [unwired: 14 in]
      }
      frame "Process: Calculate Freezing Points" {
        # "Your code here.\n(You can make a copy of, or modify, this frame)"
        n470 = local read "Temps grads"() -> (w882:dbl[][])
        n471 = Unbundle By Name(w876) -> ("Config.Freezing.Cutoff"=w875:dbl)
        n472 = local read "Temps"() -> (w881:dbl[][])
        n473 = for {
          tunnel: w882 -> [w889] mode=indexing
          workers-P: _ -> [_]
          tunnel: w881 -> [w898] mode=indexing
          tunnel: [w893] -> w880 mode=indexing
          tunnel: [w891] -> w879 mode=indexing
          tunnel: [w887] -> w878 mode=indexing
          tunnel: w875 -> [w886]
          # "Gradient Check"
          n474 = call <vilib>:"Std Deviation and Variance.vi"("X"=w889) -> ("standard deviation"=w888:dbl)  [unwired: 1 in, 2 out]
          n475 = Array Max & Min(array=w889) -> (max value=w896:dbl, max index (indices)=w892:i32)  [unwired: 2 out]
          n476 = Multiply(x=w886, y=w888) -> (x*y=w895:dbl)
          n477 = Array Subset(array=w898, length=w892) -> (w897:dbl[])  [unwired: 1 in]
          n478 = Greater?(x=w896, y=w895) -> (0:w894:bool)
          n479 = Array Max & Min(array=w897) -> (min value=w890:dbl)  [unwired: 3 out]
          n480 = case shown="False" w894 {
            selector: w894 -> [w900 w901]
            tunnel: [w899 w903] -> w893
            tunnel: w892 -> [_ w903]
            tunnel: [w899 w902] -> w891
            tunnel: w890 -> [_ w902]
            tunnel: [w900 w901] -> w887
            frame False {
              w899 = 0.0
            }
            frame True {
            }
          }
        }
        "FreezeIdx" <- w880
        "FreezeTemps" <- w879
        "FreezeArray" <- w878
        n481 = call <vilib>:"Add State(s) to Queue__JKI_lib_State_Machine.vi"("State(s) in Front (\"\")"="UI: Menu Save >> True\nUI: Menu Overlay Temps >> True" ("State(s) in Front (\"\")"), "State(s) in (\"\")"=w885) -> ("States Out"=w884:string)  [unwired: 13 in]
      }
      frame "Process: Calculate Melt Temp" {
        # "Your code here.\n(You can make a copy of, or modify, this frame)"
        n482 = local read "FreezeIdx"() -> (w906:i32[])
        n483 = local read "Temps"() -> (w905:dbl[][])
        n484 = for {
          tunnel: w906 -> [w911] mode=indexing
          workers-P: _ -> [_]
          tunnel: w905 -> [w916] mode=indexing
          tunnel: [w914] -> w904 mode=indexing
          n485 = Array Subset(array=w916, index=w911) -> (w915:dbl[])  [unwired: 1 in]
          n486 = Not Equal To 0?(x=w911) -> (x != 0?=w912:bool)
          n487 = Array Max & Min(array=w915) -> (max value=w913:dbl)  [unwired: 3 out]
          n488 = case shown="False" w912 {
            tunnel: [0.0 w918] -> w914
            tunnel: w913 -> [_ w918]
            frame False {
            }
            frame True {
            }
          }
        }
        "MeltTemps" <- w904
        n489 = call <vilib>:"Add State(s) to Queue__JKI_lib_State_Machine.vi"("State(s) in (\"\")"=w910) -> ("States Out"=w909:string)  [unwired: 14 in]
      }
      frame "Process: Calculate Freeze Fraction" {
        # "Your code here.\n(You can make a copy of, or modify, this frame)"
        n490 = property on="FrozenFractionGraph" class="WFGraph (strict)"("Active Plot"=u32 0, "Legend Visible"=TRUE ("Legend:Visible")) -> ()  [unwired: 2 in, 2 out]
        n491 = local read "PartitionArray"() -> (w922:string[])
        n492 = local read "FreezeTemps"() -> (w927:dbl[])
        n493 = local read "FreezeIdx"() -> (w925:i32[])
        n494 = local read "Temps"() -> (w926:dbl[][])
        n495 = call "FrozenFraction_Calcualte.vi"("FreezeIdx"=w925, "Temps"=w926, "FreezeTemps"=w927, "PartitionArray"=w922) -> ("FreezeFract Concatinated"=→"FreezeFract Concatinated":dbl[], "FrozenFractionGraph"=→"FrozenFractionGraph":dbl[][])  [unwired: 6 in]
        n496 = call "WellPartition_Index.vi"("PartitionArray"=w922) -> ("Unique Part Array"=w921:string[])  [unwired: 1 in, 1 out]
        n497 = for {
          tunnel: w921 -> [w933] mode=indexing
          i -> [w932]
          n498 = property on="FrozenFractionGraph" class="WFGraph (strict)"("Active Plot"=w932, "Plot.Plot Name"=w933) -> ()  [unwired: 2 in, 2 out]
        }
        n499 = call <vilib>:"Add State(s) to Queue__JKI_lib_State_Machine.vi"("State(s) in (\"\")"=w931) -> ("States Out"=w930:string)  [unwired: 14 in]
      }
      frame "Process: Calculate Offset" {
        # "Your code here.\n(You can make a copy of, or modify, this frame)"
        n500 = local read "ThermTemps"() -> (w935:dbl[])
        n501 = call "TCam_FixpointTemps.vi"("input cluster"=w936, "Therm_Temps"=w935) -> ("Offsets"=→"Offsets":dbl[])  [unwired: 1 out]
        n502 = call <vilib>:"Add State(s) to Queue__JKI_lib_State_Machine.vi"("State(s) in (\"\")"=w939) -> ("States Out"=w938:string)  [unwired: 14 in]
      }
      frame "Process: Correct Offset" {
        # "Your code here.\n(You can make a copy of, or modify, this frame)"
        n503 = local read "Temps"() -> (w942:dbl[][])
        n504 = local read "Offsets"() -> (w941:dbl[])
        n505 = for {
          tunnel: w942 -> [w949] mode=indexing
          tunnel: w941 -> [w948]
          tunnel: [w947] -> w940 mode=indexing
          n506 = Subtract(x=w949, y=w948) -> (x-y=w947:dbl[])
        }
        n507 = local write "Temps"(w940) -> ()
        n508 = call <vilib>:"Add State(s) to Queue__JKI_lib_State_Machine.vi"("State(s) in (\"\")"=w946) -> ("States Out"=w945:string)  [unwired: 14 in]
      }
      frame "Process: Remove Offset" {
        # "Your code here.\n(You can make a copy of, or modify, this frame)"
        n509 = local read "Temps"() -> (w952:dbl[][])
        n510 = local read "Offsets"() -> (w951:dbl[])
        n511 = for {
          tunnel: w952 -> [w959] mode=indexing
          tunnel: w951 -> [w958]
          tunnel: [w957] -> w950 mode=indexing
          n512 = Add(x=w959, y=w958) -> (x+y=w957:dbl[])
        }
        n513 = local write "Temps"(w950) -> ()
        n514 = call <vilib>:"Add State(s) to Queue__JKI_lib_State_Machine.vi"("State(s) in (\"\")"=w956) -> ("States Out"=w955:string)  [unwired: 14 in]
      }
      frame "---------- Image ----------" {
        # "Template Separator\n(You can make a copy of, or modify, this frame)"
        n515 = call <vilib>:"Add State(s) to Queue__JKI_lib_State_Machine.vi"("State(s) in (\"\")"=w963) -> ("States Out"=w962:string)  [unwired: 14 in]
      }
      frame "Image: Draw" {
        # "Template Separator\n(You can make a copy of, or modify, this frame)"
        n516 = call <vilib>:"Add State(s) to Queue__JKI_lib_State_Machine.vi"("State(s) in Front (\"\")"="UI: Cursor Set >> Busy\nImage: Clear ROI\nImage: Calculate BR\nImage: Calculate y space\nImage: Calculate x space\nImage: Calculate Positions\nImage: Drawlines\nImage: Draw Points\nUI: Cursor Set >> Idle" ("State(s) in Front (\"\")"), "State(s) in (\"\")"=w968) -> ("States Out"=w967:string)  [unwired: 13 in]
      }
      frame "Image: Redraw" {
        # "Template Separator\n(You can make a copy of, or modify, this frame)"
        n517 = call <vilib>:"Add State(s) to Queue__JKI_lib_State_Machine.vi"("State(s) in Front (\"\")"="UI: Cursor Set >> Busy\nImage: Clear ROI\nImage: Drawlines\nImage: Draw Points\nProcess: Calculate Temps\nUI: Cursor Set >> Idle" ("State(s) in Front (\"\")"), "State(s) in (\"\")"=w973) -> ("States Out"=w972:string)  [unwired: 13 in]
      }
      frame "Image: Set Cursors" {
        w974 = -45.0 ("X Scale.Range:Minimum")
        w975 = 40.0 ("Y Scale.Range:Maximum")
        w976 = 0 ("lower limit")
        # "Template Separator\n(You can make a copy of, or modify, this frame)"
        n518 = local read "ImageIdx"() -> (w978:u32)
        n519 = local read "maxSize"() -> (w977:i32)
        n520 = property on="Temps single" class="WFGraph (strict)"("Cursor.Cursor X"=w978, "XScale.Maximum"=w977, "XScale.Minimum"=w976, "YScale.Maximum"=w975, "YScale.Minimum"=w974) -> ()  [unwired: 2 in, 2 out]
        n521 = property on="Temps" class="WFGraph (strict)"("Cursor.Cursor X"=w978, "XScale.Maximum"=w977, "XScale.Minimum"=w976, "YScale.Maximum"=w975, "YScale.Minimum"=w974) -> ()  [unwired: 2 in, 2 out]
        n522 = property on="FrozenFractionGraph" class="WFGraph (strict)"("Cursor.Cursor X"=w978, "XScale.Maximum"=w977, "XScale.Minimum"=w976) -> ()  [unwired: 2 in, 2 out]
        n523 = property on="Fraction Single" class="WFGraph (strict)"("Cursor.Cursor X"=w978, "XScale.Maximum"=w977, "XScale.Minimum"=w976) -> ()  [unwired: 2 in, 2 out]
        n524 = property on="Temps single grad" class="WFGraph (strict)"("Cursor.Cursor X"=w978, "XScale.Maximum"=w977, "XScale.Minimum"=w976) -> ()  [unwired: 2 in, 2 out]
        n525 = property on="Temps" class="WFGraph (strict)"("Cursor.Cursor X"=w978, "XScale.Maximum"=w977, "XScale.Minimum"=w976) -> ()  [unwired: 2 in, 2 out]
        n526 = call <vilib>:"Add State(s) to Queue__JKI_lib_State_Machine.vi"("State(s) in (\"\")"=w982) -> ("States Out"=w981:string)  [unwired: 14 in]
      }
      frame "Image: Drawlines" {
        # "Template Separator\n(You can make a copy of, or modify, this frame)"
        n527 = Unbundle By Name(w983) -> ("Points.Top Left.X"=w999:sgl, "Points.Top Right.X"=w998:sgl, "Points.Bottom Left.X"=w997:sgl, "Points.Bottom Right.X"=w996:sgl)
        n528 = Equal To 0?(x=w999) -> (x = 0?=w995:bool)
        n529 = Equal To 0?(x=w998) -> (x = 0?=w994:bool)
        n530 = Equal To 0?(x=w997) -> (x = 0?=w985:bool)
        n531 = Equal To 0?(x=w996) -> (x = 0?=w986:bool)
        n532 = Or(x=w985, y=w986) -> (x .or. y?=w984:bool)
        n533 = Select(t="", s=w985, f="Image: Draw Line >> TL_BL\n") -> (s? t:f=w991:string)
        n534 = Select(t="", s=w984, f="Image: Draw Line >> TR_BR\nImage: Draw Line >> BL_BR\nImage: Draw Line >> Vertical\nImage: Draw Line >> Horizontal") -> (s? t:f=w988:string)
        n535 = case shown="False" w995 {
          tunnel: w994 -> [w1006 _]
          tunnel: w991 -> [w1005 _]
          tunnel: w988 -> [w1004 _]
          tunnel: [w1003 _] -> w987
          frame False {
            n536 = case shown="False" w1006 {
              tunnel: w1005 -> [w1009 _]
              tunnel: w1004 -> [w1008 _]
              tunnel: [w1007 _] -> w1003
              frame False {
                n537 = Concatenate Strings("Image: Draw Line >> TL_TR\n", w1009, w1008) -> (w1007:string)
              }
              frame True {
              }
            }
          }
          frame True {
          }
        }
        n538 = call <vilib>:"Add State(s) to Queue__JKI_lib_State_Machine.vi"("State(s) in Front (\"\")"=w987, "State(s) in (\"\")"=w1002) -> ("States Out"=w1001:string)  [unwired: 13 in]
      }
      frame "Image: Draw Line" {
        w1011 = u32 2  # Width
        # "Your code here.\n(You can make a copy of, or modify, this frame)"
        n539 = Unbundle By Name(w1015) -> ("Image Out"=w1016:T1)
        n540 = case shown="\"Vertical\"" w1017 {
          tunnel: w1016 -> [w1021 w1029 w1038 w1045 w1051 w1056 w1065]
          tunnel: w1015 -> [_ w1030 w1039 w1040 w1046 w1060 w1069]
          tunnel: [w1021 w1024 w1037 w1044 w1050 w1052 w1061] -> w1014
          tunnel: w1013 -> [w1020 w1028 w1036 w1043 w1049 w1054 w1064]
          tunnel: [w1020 w1023 w1035 w1042 w1048 w1053 w1063] -> w1012
          tunnel: w1011 -> [_ w1022 w1031 _ _ w1055 w1062]
          frame "False", Default {
          }
          frame "TL_TR" {
            n541 = Unbundle By Name(w1030) -> ("Points.Top Left"=w1027:T2, "Points.Top Right"=w1026:T2)
            n542 = Build Array(w1027, w1026) -> (w1025:T2[])
            n543 = call "IMAQ Overlay Multiple Lines 2"("Image"=w1029, "Line End Points"=w1025, "error in (no error)"=w1028, "Width"=w1022) -> ("Image Out"=w1024:T1, "error out"=w1023:errorcluster)  [unwired: 10 in]
          }
          frame "TL_BL" {
            n544 = Unbundle By Name(w1039) -> ("Points.Top Left"=w1034:T2, "Points.Bottom Left"=w1033:T2)
            n545 = Build Array(w1034, w1033) -> (w1032:T2[])
            n546 = call "IMAQ Overlay Multiple Lines 2"("Image"=w1038, "Line End Points"=w1032, "error in (no error)"=w1036, "Width"=w1031) -> ("Image Out"=w1037:T1, "error out"=w1035:errorcluster)  [unwired: 10 in]
          }
          frame "Vertical" {
            n547 = call "TCam_VerticalLines.vi"("Width"=u32 1, "error in (no error)"=w1043, "Cluster"=w1040, "Refnum in"=w1045) -> ("error out"=w1042:errorcluster, "Refnum out"=w1044:T1)  [unwired: 6 in]
          }
          frame "Horizontal" {
            n548 = call "TCam_HorizontalLines.vi"("Width"=u32 1, "error in (no error)"=w1049, "Cluster"=w1046, "Refnum in"=w1051) -> ("error out"=w1048:errorcluster, "Refnum out"=w1050:T1)  [unwired: 6 in]
          }
          frame "TR_BR" {
            n549 = Unbundle By Name(w1060) -> ("Points.Top Right"=w1059:T2, "Points.Bottom Right"=w1058:T2)
            n550 = Build Array(w1059, w1058) -> (w1057:T2[])
            n551 = call "IMAQ Overlay Multiple Lines 2"("Image"=w1056, "Line End Points"=w1057, "error in (no error)"=w1054, "Width"=w1055) -> ("Image Out"=w1052:T1, "error out"=w1053:errorcluster)  [unwired: 10 in]
          }
          frame "BL_BR" {
            n552 = Unbundle By Name(w1069) -> ("Points.Bottom Left"=w1068:T2, "Points.Bottom Right"=w1067:T2)
            n553 = Build Array(w1068, w1067) -> (w1066:T2[])
            n554 = call "IMAQ Overlay Multiple Lines 2"("Image"=w1065, "Line End Points"=w1066, "error in (no error)"=w1064, "Width"=w1062) -> ("Image Out"=w1061:T1, "error out"=w1063:errorcluster)  [unwired: 10 in]
          }
        }
        n555 = local write "Image"(w1014) -> ()
        n556 = call <vilib>:"Add State(s) to Queue__JKI_lib_State_Machine.vi"("State(s) in (\"\")"=w1019) -> ("States Out"=w1018:string)  [unwired: 14 in]
      }
      frame "Image: Draw Points" {
        # "Your code here.\n(You can make a copy of, or modify, this frame)"
        n557 = Unbundle By Name(w1072) -> ("Points.Top Left.X"=w1081:sgl, "Points.Top Right.X"=w1080:sgl, "Points.Bottom Left.X"=w1079:sgl, "Points.Bottom Right.X"=w1078:sgl)
        n558 = Equal To 0?(x=w1081) -> (x = 0?=w1077:bool)
        n559 = Equal To 0?(x=w1080) -> (x = 0?=w1076:bool)
        n560 = Equal To 0?(x=w1079) -> (x = 0?=w1075:bool)
        n561 = Equal To 0?(x=w1078) -> (x = 0?=w1074:bool)
        n562 = Unbundle By Name(w1072) -> ("Image Out"=w1083:T1, "Scan Area"=w1070:dbl)
        n563 = Compound Arithmetic op=OR(w1077, w1076, w1075, w1074) -> (w1073:bool)
        n564 = case shown="False" w1073 {
          tunnel: w1083 -> [w1092 _]
          tunnel: w1072 -> [w1089 w1093]
          tunnel: [w1087 w1093] -> w1071
          tunnel: w1070 -> [w1086 _]
          frame False {
            n565 = local read "Points"() -> (w1091:T2[])
            n566 = call "TCam_CenterArray.vi"("Size"=w1086, "Point Array"=w1091, "Image in"=w1092) -> ("Array"=w1088:cluster{"X":i32, "Y":i32}[][], "Image"=w1090:T1)  [unwired: 3 in]
            n567 = local write "Image"(w1090) -> ()
            n568 = Bundle By Name(cluster=w1089, "Points.Pixels"=w1088) -> (w1087:T5)
          }
          frame True {
          }
        }
        n569 = call <vilib>:"Add State(s) to Queue__JKI_lib_State_Machine.vi"("State(s) in (\"\")"=w1085) -> ("States Out"=w1084:string)  [unwired: 14 in]
      }
      frame "Image: Calculate x space" {
        # "Your code here.\n(You can make a copy of, or modify, this frame)"
        n570 = Unbundle By Name(w1102) -> ("Points.Top Left"=w1108:T2, "Points.Top Right"=w1107:T2, "PCR Size"=w1094:u16)
        n571 = case shown="0, Default" w1094 {
          tunnel: [24 12] -> w1095
          frame 0, Default {
          }
          frame 1 {
          }
        }
        n572 = Unbundle(w1108) -> ("X"=w1105:sgl, "Y"=w1103:sgl)
        n573 = Unbundle(w1107) -> ("X"=w1106:sgl, "Y"=w1104:sgl)
        n574 = Subtract(x=w1106, y=w1105) -> (x-y=w1099:sgl)
        n575 = Subtract(x=w1104, y=w1103) -> (x-y=w1097:sgl)
        n576 = Decrement(x=w1095) -> (x-1=w1098:i32)
        n577 = Divide(x=w1099, y=w1098) -> (x/y=w1100:sgl)
        n578 = Divide(x=w1097, y=w1098) -> (x/y=w1096:sgl)
        n579 = Bundle By Name(cluster=w1102, "Points.x_space"=w1100, "Points.y_space"=w1096) -> (w1101:T5)
        n580 = call <vilib>:"Add State(s) to Queue__JKI_lib_State_Machine.vi"("State(s) in (\"\")"=w1111) -> ("States Out"=w1110:string)  [unwired: 14 in]
      }
      frame "Image: Calculate BR" {
        # "Your code here.\n(You can make a copy of, or modify, this frame)"
        n581 = Unbundle By Name(w1122) -> ("Points.Top Left"=w1128:T2, "Points.Top Right"=w1127:T2, "Points.Bottom Left"=w1120:T2)
        n582 = Unbundle(w1128) -> ("X"=w1125:sgl, "Y"=w1123:sgl)
        n583 = Unbundle(w1120) -> ("X"=w1119:sgl, "Y"=w1117:sgl)
        n584 = Unbundle(w1127) -> ("X"=w1126:sgl, "Y"=w1124:sgl)
        n585 = Subtract(x=w1126, y=w1125) -> (x-y=w1118:sgl)
        n586 = Add(x=w1119, y=w1118) -> (x+y=w1114:sgl)
        n587 = Subtract(x=w1124, y=w1123) -> (x-y=w1116:sgl)
        n588 = Add(x=w1116, y=w1117) -> (x+y=w1115:sgl)
        n589 = Bundle By Name(cluster=w1122, "Points.Bottom Right.X"=w1114, "Points.Bottom Right.Y"=w1115) -> (w1121:T5)
        n590 = call <vilib>:"Add State(s) to Queue__JKI_lib_State_Machine.vi"("State(s) in (\"\")"=w1131) -> ("States Out"=w1130:string)  [unwired: 14 in]
      }
      frame "Image: Calculate y space" {
        # "Your code here.\n(You can make a copy of, or modify, this frame)"
        n591 = Unbundle By Name(w1140) -> ("Points.Top Left"=w1146:T2, "Points.Bottom Left"=w1145:T2, "PCR Size"=w1132:u16)
        n592 = case shown="1" w1132 {
          tunnel: [16 8] -> w1133
          frame 0, Default {
          }
          frame 1 {
          }
        }
        n593 = Unbundle(w1146) -> ("X"=w1143:sgl, "Y"=w1141:sgl)
        n594 = Unbundle(w1145) -> ("X"=w1144:sgl, "Y"=w1142:sgl)
        n595 = Subtract(x=w1144, y=w1143) -> (x-y=w1137:sgl)
        n596 = Subtract(x=w1142, y=w1141) -> (x-y=w1135:sgl)
        n597 = Decrement(x=w1133) -> (x-1=w1136:i32)
        n598 = Divide(x=w1137, y=w1136) -> (x/y=w1138:sgl)
        n599 = Divide(x=w1135, y=w1136) -> (x/y=w1134:sgl)
        n600 = Bundle By Name(cluster=w1140, "Points.x space 2"=w1138, "Points.y space 2"=w1134) -> (w1139:T5)
        n601 = call <vilib>:"Add State(s) to Queue__JKI_lib_State_Machine.vi"("State(s) in (\"\")"=w1149) -> ("States Out"=w1148:string)  [unwired: 14 in]
      }
      frame "Image: Calculate Positions" {
        # "Your code here.\n(You can make a copy of, or modify, this frame)"
        n602 = Unbundle By Name(w1154) -> ("Scan Area"=w1152:dbl, "Points.Top Left.X"=w1162:sgl, "Points.Top Right.X"=w1161:sgl, "Points.Bottom Left.X"=w1160:sgl, "Points.Bottom Right.X"=w1159:sgl)
        n603 = Equal To 0?(x=w1162) -> (x = 0?=w1158:bool)
        n604 = Equal To 0?(x=w1161) -> (x = 0?=w1157:bool)
        n605 = Equal To 0?(x=w1160) -> (x = 0?=w1156:bool)
        n606 = Equal To 0?(x=w1159) -> (x = 0?=w1155:bool)
        n607 = Compound Arithmetic op=OR(w1158, w1157, w1156, w1155) -> (w1153:bool)
        n608 = case shown="False" w1153 {
          tunnel: w1154 -> [w1167 _]
          tunnel: w1152 -> [w1166 _]
          frame False {
            n609 = call "TCam_PointCalculator.vi"("Cluster"=w1167, "Size"=w1166) -> ("Points"=→"Points":T2[])  [unwired: 9 in]
          }
          frame True {
          }
        }
        n610 = call <vilib>:"Add State(s) to Queue__JKI_lib_State_Machine.vi"("State(s) in (\"\")"=w1165) -> ("States Out"=w1164:string)  [unwired: 14 in]
      }
      frame "Image: Clear ROI" {
        # "Your code here.\n(You can make a copy of, or modify, this frame)"
        n611 = Unbundle By Name(w1172) -> ("Image Out"=w1171:T1)
        n612 = call "IMAQ Clear Overlay"("error in (no error)"=w1170, "Image"=w1171) -> ("error out"=w1169:errorcluster)  [unwired: 8 in, 1 out]
        n613 = call <vilib>:"Add State(s) to Queue__JKI_lib_State_Machine.vi"("State(s) in (\"\")"=w1174) -> ("States Out"=w1173:string)  [unwired: 14 in]
      }
      frame "Image: Set ROI" {
        # "Your code here.\n(You can make a copy of, or modify, this frame)"
        n614 = Unbundle By Name(w1178) -> ("State"=w1180:i32)
        n615 = case shown="0, Default" w1180 {
          tunnel: [w1184 w1187 w1189 w1191] -> w1179
          tunnel: w1178 -> [w1185 w1186 w1188 w1190]
          frame 0, Default {
            n616 = Unbundle By Name(w1185) -> ("Points.Top Left"=w1184:T2)
          }
          frame 1 {
            n617 = Unbundle By Name(w1186) -> ("Points.Top Right"=w1187:T2)
          }
          frame 2 {
            n618 = Unbundle By Name(w1188) -> ("Points.Bottom Left"=w1189:T2)
          }
          frame 3 {
            n619 = Unbundle By Name(w1190) -> ("Points.Bottom Right"=w1191:T2)
          }
        }
        n620 = call "IMAQ Convert Point to ROI"("error in (no error)"=w1177, "Point"=w1179) -> ("error out"=w1176:errorcluster, "ROI Descriptor"=w1181:T10)  [unwired: 7 in]
        n621 = property on="Image" class="ImageControl"(error in=w1176, "ROI"=w1181) -> (error out=w1175:errorcluster)  [unwired: 1 in, 1 out]
        n622 = call <vilib>:"Add State(s) to Queue__JKI_lib_State_Machine.vi"("State(s) in (\"\")"=w1183) -> ("States Out"=w1182:string)  [unwired: 14 in]
      }
      frame "---------- Overlay ----------" {
        # "Template Separator\n(You can make a copy of, or modify, this frame)"
        n623 = call <vilib>:"Add State(s) to Queue__JKI_lib_State_Machine.vi"("State(s) in (\"\")"=w1195) -> ("States Out"=w1194:string)  [unwired: 14 in]
      }
      frame "Overlay: Overlay Freeze" {
        # "Your code here.\n(You can make a copy of, or modify, this frame)"
        n624 = local read "FreezeArray"() -> (w1197:bool[])
        n625 = local read "FreezeIdx"() -> (w1198:i32[])
        n626 = local read "Points"() -> (w1199:T2[])
        n627 = Unbundle By Name(w1201) -> ("img_array"=w1200:T1[])
        n628 = call "OverlayFreezeRange.vi"("FreezeIdx"=w1198, "FreezeArray"=w1197) -> ("Range"=w1196:i32)
        n629 = for {
          N -> [w1207]
          tunnel: w1198 -> [w1219] mode=indexing
          tunnel: w1200 -> [w1220]
          tunnel: w1199 -> [w1218] mode=indexing
          tunnel: w1197 -> [w1217] mode=indexing
          tunnel: w1196 -> [w1216]
          n630 = local read "img"() -> (w1208:i32)
          n631 = case shown="True" w1217 {
            tunnel: w1220 -> [_ w1228]
            tunnel: w1219 -> [_ w1221]
            tunnel: w1218 -> [_ w1226]
            tunnel: w1216 -> [_ w1223]
            frame False {
            }
            frame True {
              n632 = Divide(x=w1221, y=w1223) -> (x/y=w1225:dbl)
              n633 = Array Subset(array=w1228, index=w1221) -> (w1227:T1[])  [unwired: 1 in]
              n634 = Multiply(x=w1225, y=30.0) -> (x*y=w1222:dbl)
              n635 = for {
                tunnel: w1227 -> [w1234] mode=indexing
                tunnel: w1226 -> [w1233]
                workers-P: _ -> [_]
                tunnel: w1222 -> [w1232]
                n636 = call "ColorRamp.vi"("Slide"=w1232) -> ("Color"=w1231:u32)
                n637 = call "IMAQ Overlay Text"("BG Color (Transparent)"=w1231, "Font, Size & Style"=T9 {"Desired Font (Application)"=enum."Application Font", "[User-specified Font]"={"Font Name"="", "Size"=1, "Strikeout?"=FALSE, "Italic?"=FALSE, "Underline?"=FALSE, "Outline?"=FALSE, "Shadow?"=FALSE, "Bold?"=FALSE, "Rotation Angle"=0.0}, "Horizontal Alignment"=1, "Vertical Alignment"=0}, "String"="   ", "Origin"=w1233, "Image"=w1234) -> ()  [unwired: 5 in, 2 out]
              }
            }
          }
          n638 = Increment(x=w1208) -> (x+1=w1215:i32)
          n639 = Divide(x=w1208, y=w1207) -> (x/y=w1214:dbl)
          n640 = local write "img"(w1215) -> ()
          n641 = Multiply(x=w1214, y=100.0) -> (x*y=w1213:dbl)
          n642 = local write "Slide"(w1213) -> ()
          n643 = Format Into String(initial string="Overlaying Well " ("Tutorial"), w1208) -> (resulting string=w1210:string)  [unwired: 2 in, 1 out]
          n644 = Format Into String(initial string=" of ", w1207) -> (resulting string=w1211:string)  [unwired: 2 in, 1 out]
          n645 = Concatenate Strings(w1210, w1211) -> (w1209:string)
          n646 = local write "Tutorial"(w1209) -> ()
        }
        n647 = call <vilib>:"Add State(s) to Queue__JKI_lib_State_Machine.vi"("State(s) in (\"\")"=w1204) -> ("States Out"=w1203:string)  [unwired: 14 in]
      }
      frame "Overlay: Overlay Freeze Temps" {
        # "Your code here.\n(You can make a copy of, or modify, this frame)"
        n648 = local read "FreezeTemps"() -> (w1238:dbl[])
        n649 = local read "FreezeArray"() -> (w1236:bool[])
        n650 = local read "FreezeIdx"() -> (w1237:i32[])
        n651 = local read "Points"() -> (w1239:T2[])
        n652 = Unbundle By Name(w1241) -> ("img_array"=w1240:T1[])
        n653 = call "OverlayFreezeRange.vi"("FreezeIdx"=w1237, "FreezeArray"=w1236) -> ("Range"=w1235:i32)
        n654 = for {
          N -> [w1245]
          tunnel: w1237 -> [w1260] mode=indexing
          tunnel: w1240 -> [w1261]
          tunnel: w1239 -> [w1259] mode=indexing
          tunnel: w1238 -> [w1258] mode=indexing
          tunnel: w1236 -> [w1257] mode=indexing
          tunnel: w1235 -> [w1256]
          n655 = local read "img"() -> (w1255:i32)
          n656 = case shown="True" w1257 {
            tunnel: w1261 -> [_ w1270]
            tunnel: w1260 -> [_ w1262]
            tunnel: w1259 -> [_ w1268]
            tunnel: w1258 -> [_ w1265]
            tunnel: w1256 -> [_ w1264]
            frame False {
            }
            frame True {
              n657 = Divide(x=w1262, y=w1264) -> (x/y=w1267:dbl)
              n658 = Array Subset(array=w1270, index=w1262) -> (w1269:T1[])  [unwired: 1 in]
              n659 = Multiply(x=w1267, y=30.0) -> (x*y=w1263:dbl)
              n660 = for {
                tunnel: w1269 -> [w1275] mode=indexing
                tunnel: w1268 -> [w1274]
                tunnel: w1265 -> [w1273]
                workers-P: _ -> [_]
                tunnel: w1263 -> [w1272]
                n661 = call "ColorRamp.vi"("Slide"=w1272) -> ("Color"=w1271:u32)
                n662 = Format Into String(format string="%3.2f", w1273) -> (resulting string=w1278:string)  [unwired: 2 in, 1 out]
                n663 = call "IMAQ Overlay Text"("BG Color (Transparent)"=w1271, "Font, Size & Style"=T9 {"Desired Font (Application)"=enum."Application Font", "[User-specified Font]"={"Font Name"="", "Size"=6, "Strikeout?"=FALSE, "Italic?"=FALSE, "Underline?"=FALSE, "Outline?"=FALSE, "Shadow?"=FALSE, "Bold?"=FALSE, "Rotation Angle"=0.0}, "Horizontal Alignment"=1, "Vertical Alignment"=0}, "String"=w1278, "Origin"=w1274, "Image"=w1275) -> ()  [unwired: 5 in, 2 out]
              }
            }
          }
          n664 = Increment(x=w1255) -> (x+1=w1249:i32)
          n665 = Divide(x=w1255, y=w1245) -> (x/y=w1250:dbl)
          n666 = local write "img"(w1249) -> ()
          n667 = Multiply(x=w1250, y=100.0) -> (x*y=w1251:dbl)
          n668 = local write "Slide"(w1251) -> ()
          n669 = Format Into String(initial string="Overlaying Well " ("Tutorial"), w1255) -> (resulting string=w1253:string)  [unwired: 2 in, 1 out]
          n670 = Format Into String(initial string=" of ", w1245) -> (resulting string=w1252:string)  [unwired: 2 in, 1 out]
          n671 = Concatenate Strings(w1253, w1252) -> (w1254:string)
          n672 = local write "Tutorial"(w1254) -> ()
        }
        n673 = call <vilib>:"Add State(s) to Queue__JKI_lib_State_Machine.vi"("State(s) in (\"\")"=w1244) -> ("States Out"=w1243:string)  [unwired: 14 in]
      }
      frame "Overlay: Overlay Freeze Old" {
        # "Your code here.\n(You can make a copy of, or modify, this frame)"
        n674 = local read "FreezeArray"() -> (w1280:bool[])
        n675 = Unbundle By Name(w1283) -> ("img_array"=w1285:T1[])
        n676 = local read "FreezeIdx"() -> (w1281:i32[])
        n677 = Unbundle By Name(w1283) -> ("Points.Pixels"=w1282:cluster{"X":i32, "Y":i32}[][])
        n678 = local read "Points"() -> (w1284:T2[])
        n679 = call "OverlayFreezeRange.vi"("FreezeIdx"=w1281, "FreezeArray"=w1280) -> ("Range"=w1279:i32)
        n680 = for {
          N -> [w1291]
          tunnel: w1281 -> [w1306] mode=indexing
          tunnel: w1285 -> [w1309]
          tunnel: w1284 -> [w1307] mode=indexing
          workers-P: _ -> [_]
          tunnel: w1279 -> [w1304]
          tunnel: w1282 -> [w1303] mode=indexing
          tunnel: w1280 -> [w1289] mode=indexing
          n681 = local read "img"() -> (w1292:i32)
          n682 = Increment(x=w1292) -> (x+1=w1297:i32)
          n683 = Divide(x=w1306, y=w1304) -> (x/y=w1305:dbl)
          n684 = Array Subset(array=w1309, index=w1306) -> (w1308:T1[])  [unwired: 1 in]
          n685 = local write "img"(w1297) -> ()
          n686 = Multiply(x=w1305, y=30.0) -> (x*y=w1302:dbl)
          n687 = Divide(x=w1292, y=w1291) -> (x/y=w1300:dbl)
          n688 = case shown="True" w1289 {
            tunnel: w1308 -> [_ w1313]
            tunnel: w1307 -> [_ w1312]
            tunnel: w1303 -> [_ w1311]
            tunnel: w1302 -> [_ w1310]
            frame False {
            }
            frame True {
              n689 = for {
                tunnel: w1313 -> [w1314] mode=indexing
                tunnel: w1312 -> [w1318]
                tunnel: w1310 -> [w1316]
                tunnel: w1311 -> [w1317]
                n690 = call "ColorRamp.vi"("Slide"=w1316) -> ("Color"=w1315:u32)
                n691 = call "IMAQ Overlay Points"("Color"=w1315, "Array of Points"=w1317, "Point"=w1318, "Image"=w1314) -> ()  [unwired: 6 in, 2 out]
              }
            }
          }
          n692 = Multiply(x=w1300, y=100.0) -> (x*y=w1299:dbl)
          n693 = local write "Slide"(w1299) -> ()
          n694 = Format Into String(w1292) -> (resulting string=w1295:string)  [unwired: 3 in, 1 out]
          n695 = Format Into String(w1291) -> (resulting string=w1296:string)  [unwired: 3 in, 1 out]
          n696 = Concatenate Strings("Overlaying Well " ("Tutorial"), w1295, " of " ("Tutorial"), w1296) -> (w1294:string)
          n697 = local write "Tutorial"(w1294) -> ()
        }
        n698 = call <vilib>:"Add State(s) to Queue__JKI_lib_State_Machine.vi"("State(s) in (\"\")"=w1288) -> ("States Out"=w1287:string)  [unwired: 14 in]
      }
      frame "Overlay: Remove Overlays" {
        # "Your code here.\n(You can make a copy of, or modify, this frame)"
        n699 = Unbundle By Name(w1320) -> ("img_array"=w1319:T1[])
        n700 = for {
          tunnel: w1319 -> [w1324] mode=indexing
          n701 = call "IMAQ Clear Overlay"("Image"=w1324) -> ()  [unwired: 9 in, 2 out]
        }
        n702 = call <vilib>:"Add State(s) to Queue__JKI_lib_State_Machine.vi"("State(s) in (\"\")"=w1323) -> ("States Out"=w1322:string)  [unwired: 14 in]
      }
      frame "Overlay: Update Focus Well" {
        # "Your code here.\n(You can make a copy of, or modify, this frame)"
        n703 = local read "FrozenFractionGraph"() -> (w1326:dbl[][])
        n704 = local read "FreezeIdx"() -> (w1328:i32[])
        n705 = local read "Temps"() -> (w1336:dbl[][])
        n706 = local read "PartitionArray"() -> (w1331:string[])
        n707 = local read "Temps grads"() -> (w1335:dbl[][])
        n708 = local read "MeltTemps"() -> (w1327:dbl[])
        n709 = call "PCRNameArray.vi"("input cluster"=w1330) -> ("WellArray"=w1329:string[])
        n710 = local read "FreezeTemps"() -> (w1334:dbl[])
        n711 = local read "Well"() -> (w1332:i32)
        n712 = Empty Array?(array=w1336) -> (empty?=w1333:bool)
        n713 = case shown="False" w1333 {
          tunnel: w1332 -> [w1342 _]
          tunnel: w1336 -> [w1358 _]
          tunnel: w1335 -> [w1357 _]
          tunnel: w1334 -> [w1356 _]
          tunnel: w1331 -> [w1341 _]
          tunnel: w1329 -> [w1353 _]
          tunnel: w1328 -> [w1349 _]
          tunnel: w1327 -> [w1348 _]
          tunnel: w1326 -> [w1346 _]
          frame False {
            n714 = call "WellPartition_Index.vi"("PartitionArray"=w1341, "Well"=w1342) -> ("Partition Index"=w1343:i32)  [unwired: 1 out]
            n715 = Index Array(array=w1348, index=w1342) -> (element=→"MeltTemp":dbl)
            n716 = Index Array(array=w1358, index (row)=w1342) -> (element=w1351:dbl[])  [unwired: 1 in]
            n717 = Index Array(array=w1356, index=w1342) -> (element=→"FreezeTemp":dbl)
            n718 = Index Array(array=w1357, index (row)=w1342) -> (element=→"Temps single grad":dbl[])  [unwired: 1 in]
            n719 = Index Array(array=w1341, index=w1342) -> (element=w1340:string)
            "Contents" <- w1340
            n720 = Index Array(array=w1353, index=w1342) -> (element=→"Well":string)
            n721 = Index Array(array=w1349, index=w1342) -> (element=w1344:i32)
            n722 = Index Array(array=w1346, index (row)=w1343) -> (element=→"Fraction Single":dbl[])  [unwired: 1 in]
            n723 = Index Array(array=w1351, index=w1344) -> (element=→"CurTemp":dbl)
            n724 = local write "ImageIdx"(w1344) -> ()
            n725 = local write "Temps single"(w1351) -> ()
            n726 = property on="Fraction Single" class="WFGraph (strict)"("Plot.Plot Name"=w1340) -> ()  [unwired: 2 in, 2 out]
          }
          frame True {
          }
        }
        n727 = call <vilib>:"Add State(s) to Queue__JKI_lib_State_Machine.vi"("State(s) in Front (\"\")"="Image: Set Cursors" ("State(s) in Front (\"\")"), "State(s) in (\"\")"=w1339) -> ("States Out"=w1338:string)  [unwired: 13 in]
      }
    }
  }
